vi "One Ring_2016_11_03_AMZ_LoopTPX_Beta.vi"() -> ()   [LabVIEW 2015]
uses:
  <vilib>/Platform/TimedLoop/XDataNode/timing_clust.ctl
  <vilib>/Platform/TimedLoop/XDataNode/nitl_modes.ctl
  <vilib>/Platform/TimedLoop/XDataNode/wakeup.ctl
  <vilib>/Utility/file.llb/Read From Spreadsheet File (DBL).vi
  <vilib>/Utility/file.llb/Write To Spreadsheet File (string).vi
  <vilib>/Platform/TimedLoop/XDataNode/XDataNode.xnode
  <vilib>/Platform/TimedLoop/XDataNode/XDNodeRunTimeDep.lvlib
  OE_Group/OE_Research/Programs/JW-PD/Instrument Libraries/Lake Shore 336/Lake Shore 336.lvlib
panel:
  in  "Stop \nCountdown 2":bool
  in  "Loop Wait 2":dbl format="%<%H:%M:%S>t"
  out "Wait Countdown 2":dbl format="%<%H:%M>t"
  out "all rows":dbl[][](array[numeric]) format="%0.3f"
  out "Repeat Loop":i32
  out "Measurement Repeat":bool
  out "Measurement Error":bool
  out "Stop buffer":dbl
  out "Start buffer":dbl
  out "Status":path
  out "Settle Time (s)":dbl
  out "Current Step":dbl
  out "D":dbl
  out "I":dbl
  out "P":dbl
  out "Out2 Ramp":dbl
  out "Out1 Ramp":dbl
  out "Temp Max Alarm":bool
  out "Temp Min Alarm":bool
  out "Out 2\nActive":bool
  out "Out 2\nRamp On":bool
  out "Out 1\nRamp On":bool
  out "Out 1\nActive":bool
  in  "Time Iteration (s)":dbl=30.0
  out "Electrical Measurements":path
  out "Temperature Measurements":path
  out "output control loop":dbl
  out "AutoTune Stage":dbl
  out "AutoTune Error":bool
  out "AutoTune Active":bool
  out "Array 2":i32[](array[numeric])
  out "Array":i32[](array[numeric])
  out "Start Time Num":dbl
  in  "Temp Sample Time (s)":dbl
  out "Current Rate (K/min)":dbl
  in  "Tab Control":T1(tab)
  in  "Light Bathe Cluster":T2={"TG to BG (TRF):  "=FALSE, "TG to BG Durration"=120.0, "TRF to TSP:   "=FALSE, "TG to BG Durration 2"=120.0, "Post Measure: "=TRUE, "TG to BG (TSP):"=FALSE, "TG to BG Durration 3"=120.0} {"TG to BG Durration 3" format="%<%H:%M:%S>t"; "TG to BG Durration 2" format="%<%H:%M:%S>t"; "TG to BG Durration" format="%<%H:%M:%S>t"}
  in  "Gated SMU4 is...":bool
  in  "Light is...":bool
  in  "SD Transport Tab":enum32{"Transport", "Gate Current"}(tab)
  out "Transport Graph":cluster{dbl[], "trace":dbl[]}[](graph) caption="Transfer"
  out "TSP Gate Current":cluster{"Y":dbl[], "Y":dbl[]}[](graph)
  in  "SD Transfer Tab":T3(tab)=enum."Saturation"
  out "Linear Transfer":cluster{"Y":dbl[], "Y":dbl[]}[](graph)
  out "Saturation Transfer":cluster{"Y":dbl[], "Y":dbl[]}[](graph)
  out "Linear Raw":cluster{"Y":dbl[], "Y":dbl[]}[](graph)
  out "Saturation Raw":cluster{"Y":dbl[], "Y":dbl[]}[](graph)
  out "TSF Gate Current":cluster{"Y":dbl[], "Y":dbl[]}[](graph)
  out "Off Current":dbl format="%#_3g"
  out "Mobility-Lin":dbl format="%#_3g"
  out "Trap Density-VT":dbl format="%#_3g"
  in  "First Step":dbl
  out "Trap Density-STS":dbl format="%#_3g"
  out "STS":dbl format="%#_3g"
  out "Vt":dbl format="%#_3g"
  in  "Transfer 2":bool=TRUE
  in  "Transport":bool=TRUE
  out "Error":errorcluster
  in  "Integration Time 3":u32(slide) scale=0.0..2.0
  in  "Integration Time":u32(slide) scale=0.0..2.0
  in  "Start 2":dbl=40.0 format="%.2f"
  in  "Stop 2":dbl=-40.0 format="%.2f"
  in  "Step 2":dbl=-1.0 format="%.2f"
  in  "Start":dbl=-2.0 format="%.2f"
  in  "Total Points":u16=2
  in  "Step":dbl=-38.0 format="%.2f"
  in  "Sample Properties:":T4={"Date Created"=timestamp(0 s since 1904-01-01), "Material"="", "Solvent"="", "Concentration"="", "Method"="", "Dielectric (d)"="", "Index (#)"="", "Index (ABC)"="", "Length"="", "Width"="", "Surface Treatment"="", "Comments"="", "T (K)"=294.0} {"T (K)" format="%#_4g"; "Date Created" format="%<%Y/%m/%d>T"}
  in  "Start":dbl format="%.2f"
  in  "Stop 3":dbl=-60.0 format="%.2f"
  in  "Step":dbl=-1.0 format="%.2f"
  in  "Start":dbl format="%.2f"
  in  "Total Points":u16=7
  in  "Step":dbl=-10.0 format="%.2f"
  out "TRF Path":path
  out "TSP Path":path
  in  "OK Button":bool
  in  "stop":bool
  out "Status LED":bool
  in  "Wait Time (s)":dbl format="%.1g"
  out "Wait Countdown":dbl format="%<%H:%M>t"
  out "Mobility-Sat":dbl format="%#_3g"
  out "On/Off":dbl format="%#_3g"
  in  "# of Loops":dbl=1.0
  in  "Loop Step":dbl
  in  "Loop Wait":dbl format="%<%H:%M:%S>t"
  in  "Stop \nCountdown":bool
  out "Delay Start":dbl format="%<%H:%M:%S>t"
  out "Light \nCount Down":dbl format="%<%H:%M:%S>t"
  in  "Light On Duration\n (min)":dbl
  in  "PR OVR":bool
  in  "PT OVR":bool
  in  "Reverse Scan (Y/N)":bool
  in  "Post Rate (K/min)":dbl format="%_2g"
  in  "Post Temp (K)":dbl format="%_4g"
  out "Status Table":string[][](table)
  out "Elapsed Time":dbl format="%<%H:%M:%S>t"
  out "Start Time":timestamp format="%<%I:%M:%S %p\n%x>T"
  out "Temp Graph":cluster{"Y":dbl[], "Y":dbl[]}[](graph)
  out "Room Temp (K)":dbl
  in  "Output 1 Range":enum16{"Off", "Low (On)", "Medium", "High"}(ring)=enum."High"
  in  "Output 2 Range":enum16{"Off", "Low (On)", "Medium", "High"}(ring)=enum."High" caption="Range (0:Off)"
  in  "Rate (K/min)":dbl=0.5 format="%.2f"
  out "Heater 3 Output":dbl format="%_3g"
  out "Heater 4 Output":dbl format="%_3g"
  in  "Sample Control":bool=TRUE
  in  "Radiation Sheild":bool=TRUE
  in  "Start (K)":dbl=80.0 format="%.2f"
  in  "# Steps":dbl=22.0
  in  "Stop (K)":dbl=300.0 format="%.2f"
  in  "Abort?":bool
  in  "TPX OK Button":bool
  out "TPX Transport Graph":cluster{"trace":dbl[], "trace":dbl[]}(graph)
  out "TPX Transfer Graph":cluster{"Y":dbl[], "Y":dbl[]}[](graph)
  out "Target":dbl caption="Target (K)"
  out "Setpoint (K)":dbl
  in  "Reset":bool
  out "Alarm":bool
  out "2":bool
  out "1":bool
  out "A:  Sample Stage":dbl format="%_6g"
  out "C:  Probe Arm":dbl format="%_6g"
  out "B:  Rad Shield":dbl format="%_6g"
  out "D:  Not Used":dbl format="%_6g"
  out "Heater 1 Output2":dbl format="%_3g"
  out "Heater 2 Output1":dbl format="%_3g"
  out "Mobility-Sat TPX":dbl caption="Mobility-Sat" format="%#_3g"
  out "On/Off TPX":dbl caption="On/Off" format="%#_3g"
  out "Vt TPX":dbl caption="Vt" format="%#_3g"
  out "STS TPX":dbl caption="STS" format="%#_3g"
  out "Trap Density STS TPX":dbl caption="Trap Density-STS" format="%#_3g"
  out "Trap Density VT TPX":dbl caption="Trap Density-VT" format="%#_3g"
  out "Mobility-Lin TPX":dbl caption="Mobility-Lin" format="%#_3g"
  out "Off Current TPX":dbl caption="Off Current" format="%#_3g"
  in  "User's Name":u16(ring) items=["Abdul", "Derek", "Jeremy", "Joshua", "Katelyn", "Oana", "Pete", "Zach"]
  in  "User's Email":string
  in  "Edit Users":bool
  in  "Top Gate Dielectric Properties":T5 {"Dielectric Constant (TG)" format="%#.2g"}
  in  "Gate Current Cluster":T6={"Gate Current (TSP)"={"Y2 axis on/off"=FALSE, "MINIMUM"=0.0, "MAXIMUM"=1.0, "Variable name"="Ig", "LIN or LOG axis"="LIN"}, "Gate Current (TRF)"={"Y2 axis on/off"=FALSE, "MINIMUM"=0.0, "MAXIMUM"=1.0, "Variable name"="Ig", "LIN or LOG axis"="LIN"}} {"Gate Current (TRF)"."MAXIMUM" format="%.3f"; "Gate Current (TRF)"."MINIMUM" format="%.3f"; "Gate Current (TSP)"."MAXIMUM" format="%.3f"; "Gate Current (TSP)"."MINIMUM" format="%.3f"}
  in  "Continue if error?":bool
  out "Error Loop #":dbl
  in  "Repeat if error?":bool
  in  "Name/Email List Location":path=path "C:/Program Files/One Ring 1.0/User_Directory.txt"
  in  "Text Editor Location":path=path "C:/Program Files/Notepad++/notepad++.exe"
  in  "Stability Time (s)":dbl=15.0
  in  "Setpoint Tolerance (K)":dbl=0.5
  in  "D: Low Alarm":dbl
  in  "D: High Alarm":dbl
  in  "Var1 sweep settings":T7={"sweep spacing (linear: 0)"=0, "sweep mode"=FALSE, "compliance (V)"=100.0, "compliance (A)"=0.001} {"compliance (A)" format="%^.2e"; "compliance (V)" format="%.2f"; "sweep spacing (linear: 0)" items=["linear", "log 10", "log 25", "log 50"]}
  in  "Var2 step settings":T8={"compliance (A)"=0.001, "compliance (V)"=100.0} {"compliance (V)" format="%.2f"; "compliance (A)" format="%^.2e"}
  in  "Var1 sweep settings 2":T7={"sweep spacing (linear: 0)"=0, "sweep mode"=FALSE, "compliance (V)"=100.0, "compliance (A)"=0.001} {"compliance (A)" format="%^.2e"; "compliance (V)" format="%.2f"; "sweep spacing (linear: 0)" items=["linear", "log 10", "log 25", "log 50"]}
  in  "Var2 step settings 2":T8={"compliance (A)"=0.001, "compliance (V)"=100.0} {"compliance (V)" format="%.2f"; "compliance (A)" format="%^.2e"}
  in  "B: Low Alarm":dbl
  in  "A: Low Alarm":dbl
  in  "B: High Alarm":dbl=350.0
  in  "A: High Alarm":dbl=350.0
  in  "C: Low Alarm":dbl
  in  "C: High Alarm":dbl
  in  "Alarm Reset 2":bool
  in  "P 2":dbl=200.0 caption="P"
  in  "I 2":dbl=50.0 caption="I"
  in  "D 2":dbl caption="D"
  in  "VISA Resource (TPX)":refnum<visa-resource-name>="GPIB9::12::INSTR"
  in  "SetPoint2\nOVR":dbl=294.0 caption="Setpoint Overide (K)"
  in  "VISA resource name":refnum<visa-resource-name>="GPIB0::17::INSTR"
  in  "Data Folder":path=path "C:/1DATA"
  in  "Image Folder:":path=path "C:/1Data/2012/zOops"
  out "Image File:":path=path "C:/Users/shuttle/Desktop"
  in  "Dielectric Constant:":dbl=3.9 format="%_2g"
  in  "Saved Folder:":path=path "C:/Users/shuttle/Desktop"
  # "Device Characteristics"
  # "Vg Sweep"
  # "Vd Step"
  # "Loops and Integration Time"
  # "Integration Time"
  # "Vd Step"
  # "Vg Step"
  # "Light Bath is..."
  # "Duration (hh:mm:ss)"
  # "Sample Properties:"
  # "%"
  # "nm"
  # "Device Properties:"
  # "um"
  # "um"
  # "Step 1:  Temperature Settings"
  # "Sample Stage"
  # "Radiation Shield"
  # "Instrument Status"
  # "Step 2:  Set the following in \"Super Duper\""
  # "%"
  # "%"
  # "K"
  # "K"
  # "1)   Sample Properties\n\n2)   Device Properties\n\n3)   Transfer and Transport Parameters"
  # "K"
  # "K"
  # "Step 3: End of Measurement Options"
  # "Device Characteristics"
  # "Lake Shore 336 Temperature Controller"
  # "Agilent 4155C Semiconductor Parameter Analyzer"
  # "One Ring Preferences"
  # "K"
  # "K"
  # "K"
  # "K"
  # "K"
  # "K"
  # "K"
  # "K"
  # "Notification Preferences"
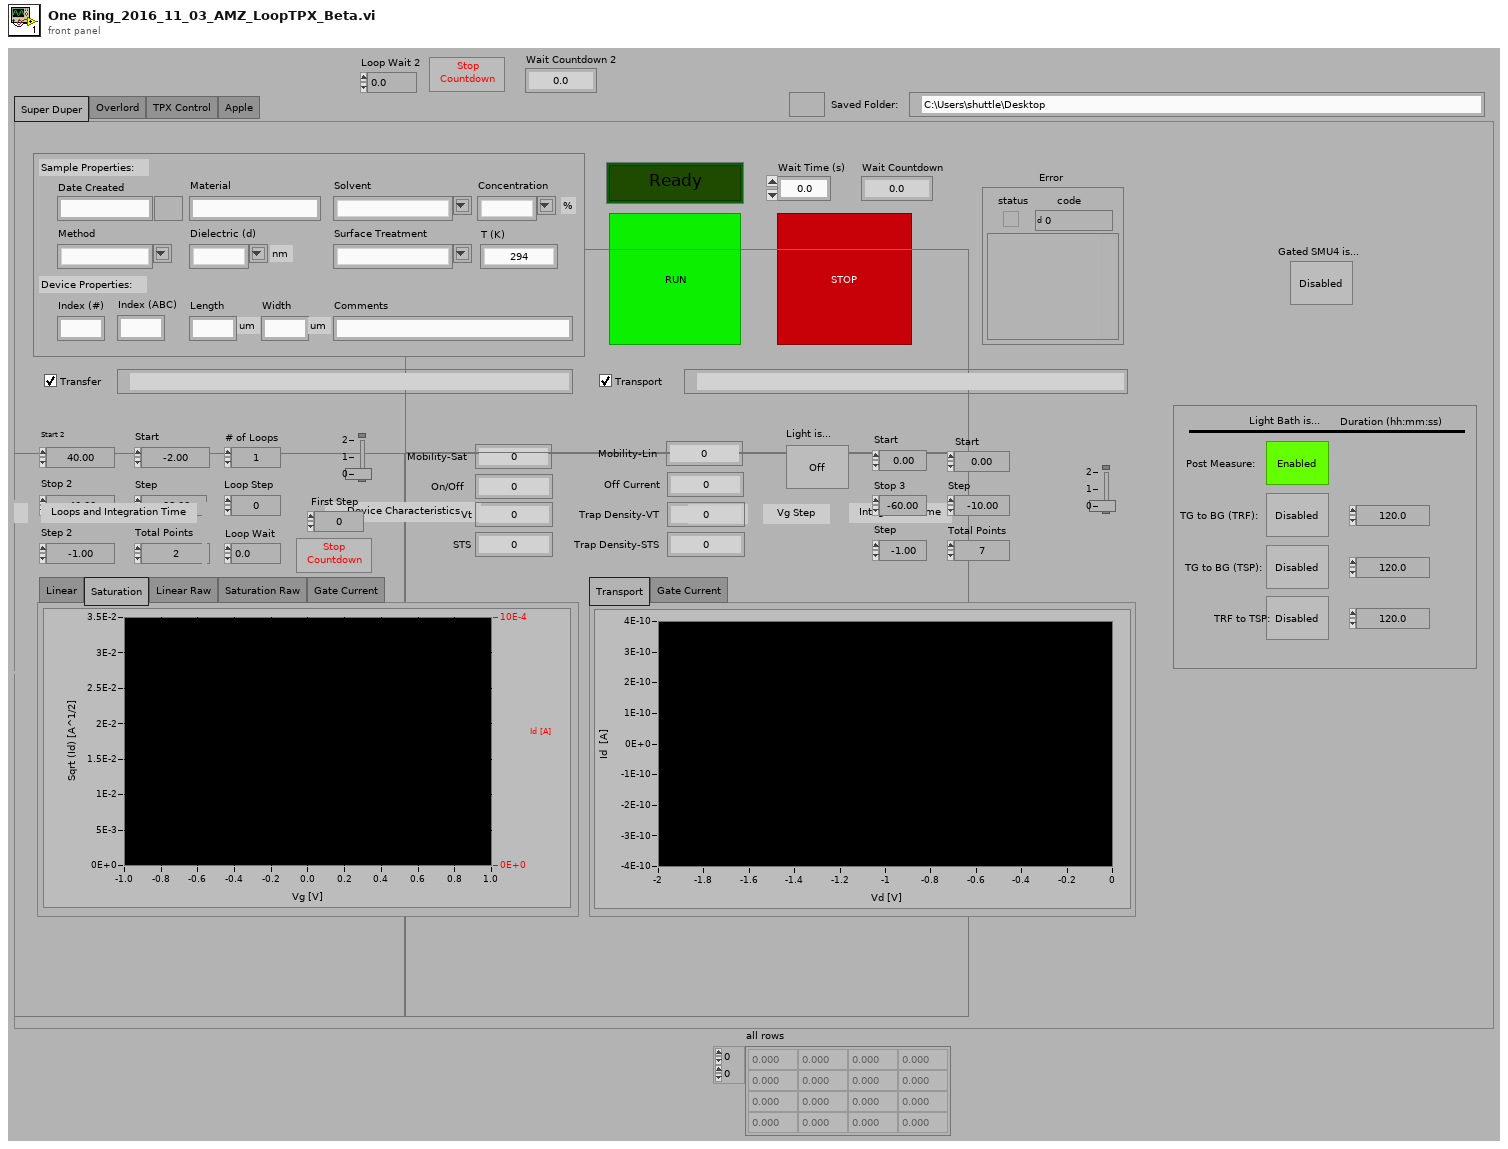
[diagram p1: front panel]
types:
  T1 = enum32{"Super Duper", "Overlord", "TPX Control", "Apple"}
  T2 = cluster{"TG to BG (TRF):  ":bool, "TG to BG Durration":dbl, "TRF to TSP:   ":bool, "TG to BG Durration 2":dbl, "Post Measure: ":bool, "TG to BG (TSP):":bool, "TG to BG Durration 3":dbl}
  T3 = enum32{"Linear", "Saturation", "Linear Raw", "Saturation Raw", "Gate Current"}
  T4 = cluster{"Date Created":timestamp, "Material":string, "Solvent":string, "Concentration":string, "Method":string, "Dielectric (d)":string, "Index (#)":string, "Index (ABC)":string, "Length":string, "Width":string, "Surface Treatment":string, "Comments":string, "T (K)":dbl}
  T5 = cluster{"Dielectric Constant (TG)":dbl, "Dielectric (d) (TG)":string}
  T6 = cluster{"Gate Current (TSP)":cluster{"Y2 axis on/off":bool, "MINIMUM":ext, "MAXIMUM":ext, "Variable name":string, "LIN or LOG axis":string}, "Gate Current (TRF)":cluster{"Y2 axis on/off":bool, "MINIMUM":ext, "MAXIMUM":ext, "Variable name":string, "LIN or LOG axis":string}}
  T7 = cluster{"sweep spacing (linear: 0)":u16, "sweep mode":bool, "compliance (V)":dbl, "compliance (A)":dbl}
  T8 = cluster{"compliance (A)":dbl, "compliance (V)":dbl}
  T9 = typedef "XDNodeRunTimeDep.lvlib/timing_clust.ctl" = cluster{"Expected End [f-1]":u64, "Actual End [f-1]":u64, "Finished Late? [f-1]":bool, "Expected End [i-1]":u64, "Actual End [i-1]":u64, "Finished Late? [i-1]":bool, "Expected Start [i]":u64, "Actual Start [i]":u64, "Expected Start [f]":u64, "Actual Start [f]":u64, "Source Name":string, "Structure Name":string, "Period":i64, "Deadline":i64, "Offset":i64, "Start":i64, "Priority":i32, "Timeout":i32, "Mode":T10, "Wakeup Reason":T11, "Error":errorcluster, "Source Type":string, "Secondary Source Type":string, "Global End Time":u64, "Global Start Time":u64, "Frame Duration":u64, "Iteration Duration":u64, "Assigned CPU":i32, "I/O Scan Engine Mode":u32}
  T10 = typedef "XDNodeRunTimeDep.lvlib/nitl_modes.ctl" = enum32{"No Change", "Process missed periods, maintain original phase", "Discard missed periods, maintain original phase", "Process missed periods, ignore original phase", "Discard missed periods, ignore original phase"}
  T11 = typedef "XDNodeRunTimeDep.lvlib/wakeup.ctl" = enum32{"Normal", "Aborted", "Asynchronous wakeup", "Timing source error", "Timed loop error", "Timeout"}
  T12 = cluster{"P":dbl, "I":dbl, "D":dbl, "SetPoint Out1":dbl, "SetPoint Out2":dbl, "1":bool, "2":bool, "output control loop":dbl, "AutoTune Error":bool, "AutoTune Active":bool, "AutoTune Stage":dbl, "Out1 Active":bool, "Out1 Ramp On":bool, "Out2 Active":bool, "Out2 Ramp On":bool, "Heater 2 Output 1":dbl, "Heater 1 Output 2":dbl, "Out1 Ramp":dbl, "Out2 Ramp":dbl}
  T13 = cluster{"A:  Sample Stage":dbl, "B:  Rad Shield":dbl, "B: Probe Arm":dbl, "Temp Max Alarm":bool, "Temp Min Alarm":bool}
  T14 = cluster{"Wait Countdown":dbl, "Wait Time (s)":dbl}
  T15 = cluster{"Step":dbl, "# of Loops":dbl, "Transfer 2":bool, "Start":dbl, "Total Points":u16, "Start 2":dbl, "Stop 2":dbl, "Step 2":dbl, "Loop Step":dbl, "Integration Time 3":u32, "Loop Wait":dbl, "First Step":dbl}
  T16 = cluster{bool, "Start":dbl, "Stop 3":dbl, "Step":dbl, "Start":dbl, "Step":dbl, "Total Points":u16, "Integration Time":u32}
  T17 = cluster{"Var1 sweep settings":cluster{"sweep spacing (linear: 0)":u16, "sweep mode":bool, "compliance (V)":dbl, "compliance (A)":dbl}, "Var1 sweep settings 2":cluster{"sweep spacing (linear: 0)":u16, "sweep mode":bool, "compliance (V)":dbl, "compliance (A)":dbl}, "Var2 step settings":cluster{"compliance (A)":dbl, "compliance (V)":dbl}, "Var2 step settings 2":cluster{"compliance (A)":dbl, "compliance (V)":dbl}}
  T18 = cluster{"Linear Transfer":cluster{dbl[], "trace":dbl[]}[], "Linear Raw":cluster{dbl[], dbl[]}[], "Saturation Transfer":cluster{dbl[], "trace":dbl[]}[], "Saturation Raw":cluster{dbl[], dbl[]}[], "Transport":cluster{dbl[], dbl[]}[], "TRF Gate Current":cluster{dbl[], dbl[]}[], "TSP Gate Current":cluster{dbl[], dbl[]}[]}
  T19 = cluster{"Mobility-Sat":dbl, "Mobility-Lin":dbl, "On/Off ":dbl, "Off I":dbl, "Vt":dbl, "STS":dbl, "Trap Density-VT":dbl, "Trap Density-STS":dbl}
  T20 = cluster{"Step":dbl, "# of Loops":dbl, bool, "Start":dbl, "Total Points":u16, "Start 2":dbl, "Stop 2":dbl, "Step 2":dbl, "Loop Step":dbl, "Integration Time 3":u32, "Loop Wait":dbl, "First Step":dbl}
  T21 = cluster{"Transport":bool, "Start":dbl, "Stop 3":dbl, "Step":dbl, "Start":dbl, "Step":dbl, "Total Points":u16, "Integration Time":u32}
  T22 = cluster{"Date Created":timestamp, "Material":string, "Solvent":string, "Concentration":string, "Method":string, "Dielectric (d)":string, "Index (#)":string, "Index (ABC)":string, "Length":string, "Width":string, "Surface Treatment":string, "Comments":string, "A:  Sample Stage":dbl}
  T23 = cluster{"Vt Max":i32, "Vt Min":i32, "Vt Ratio":i32, "Id Max":i32}
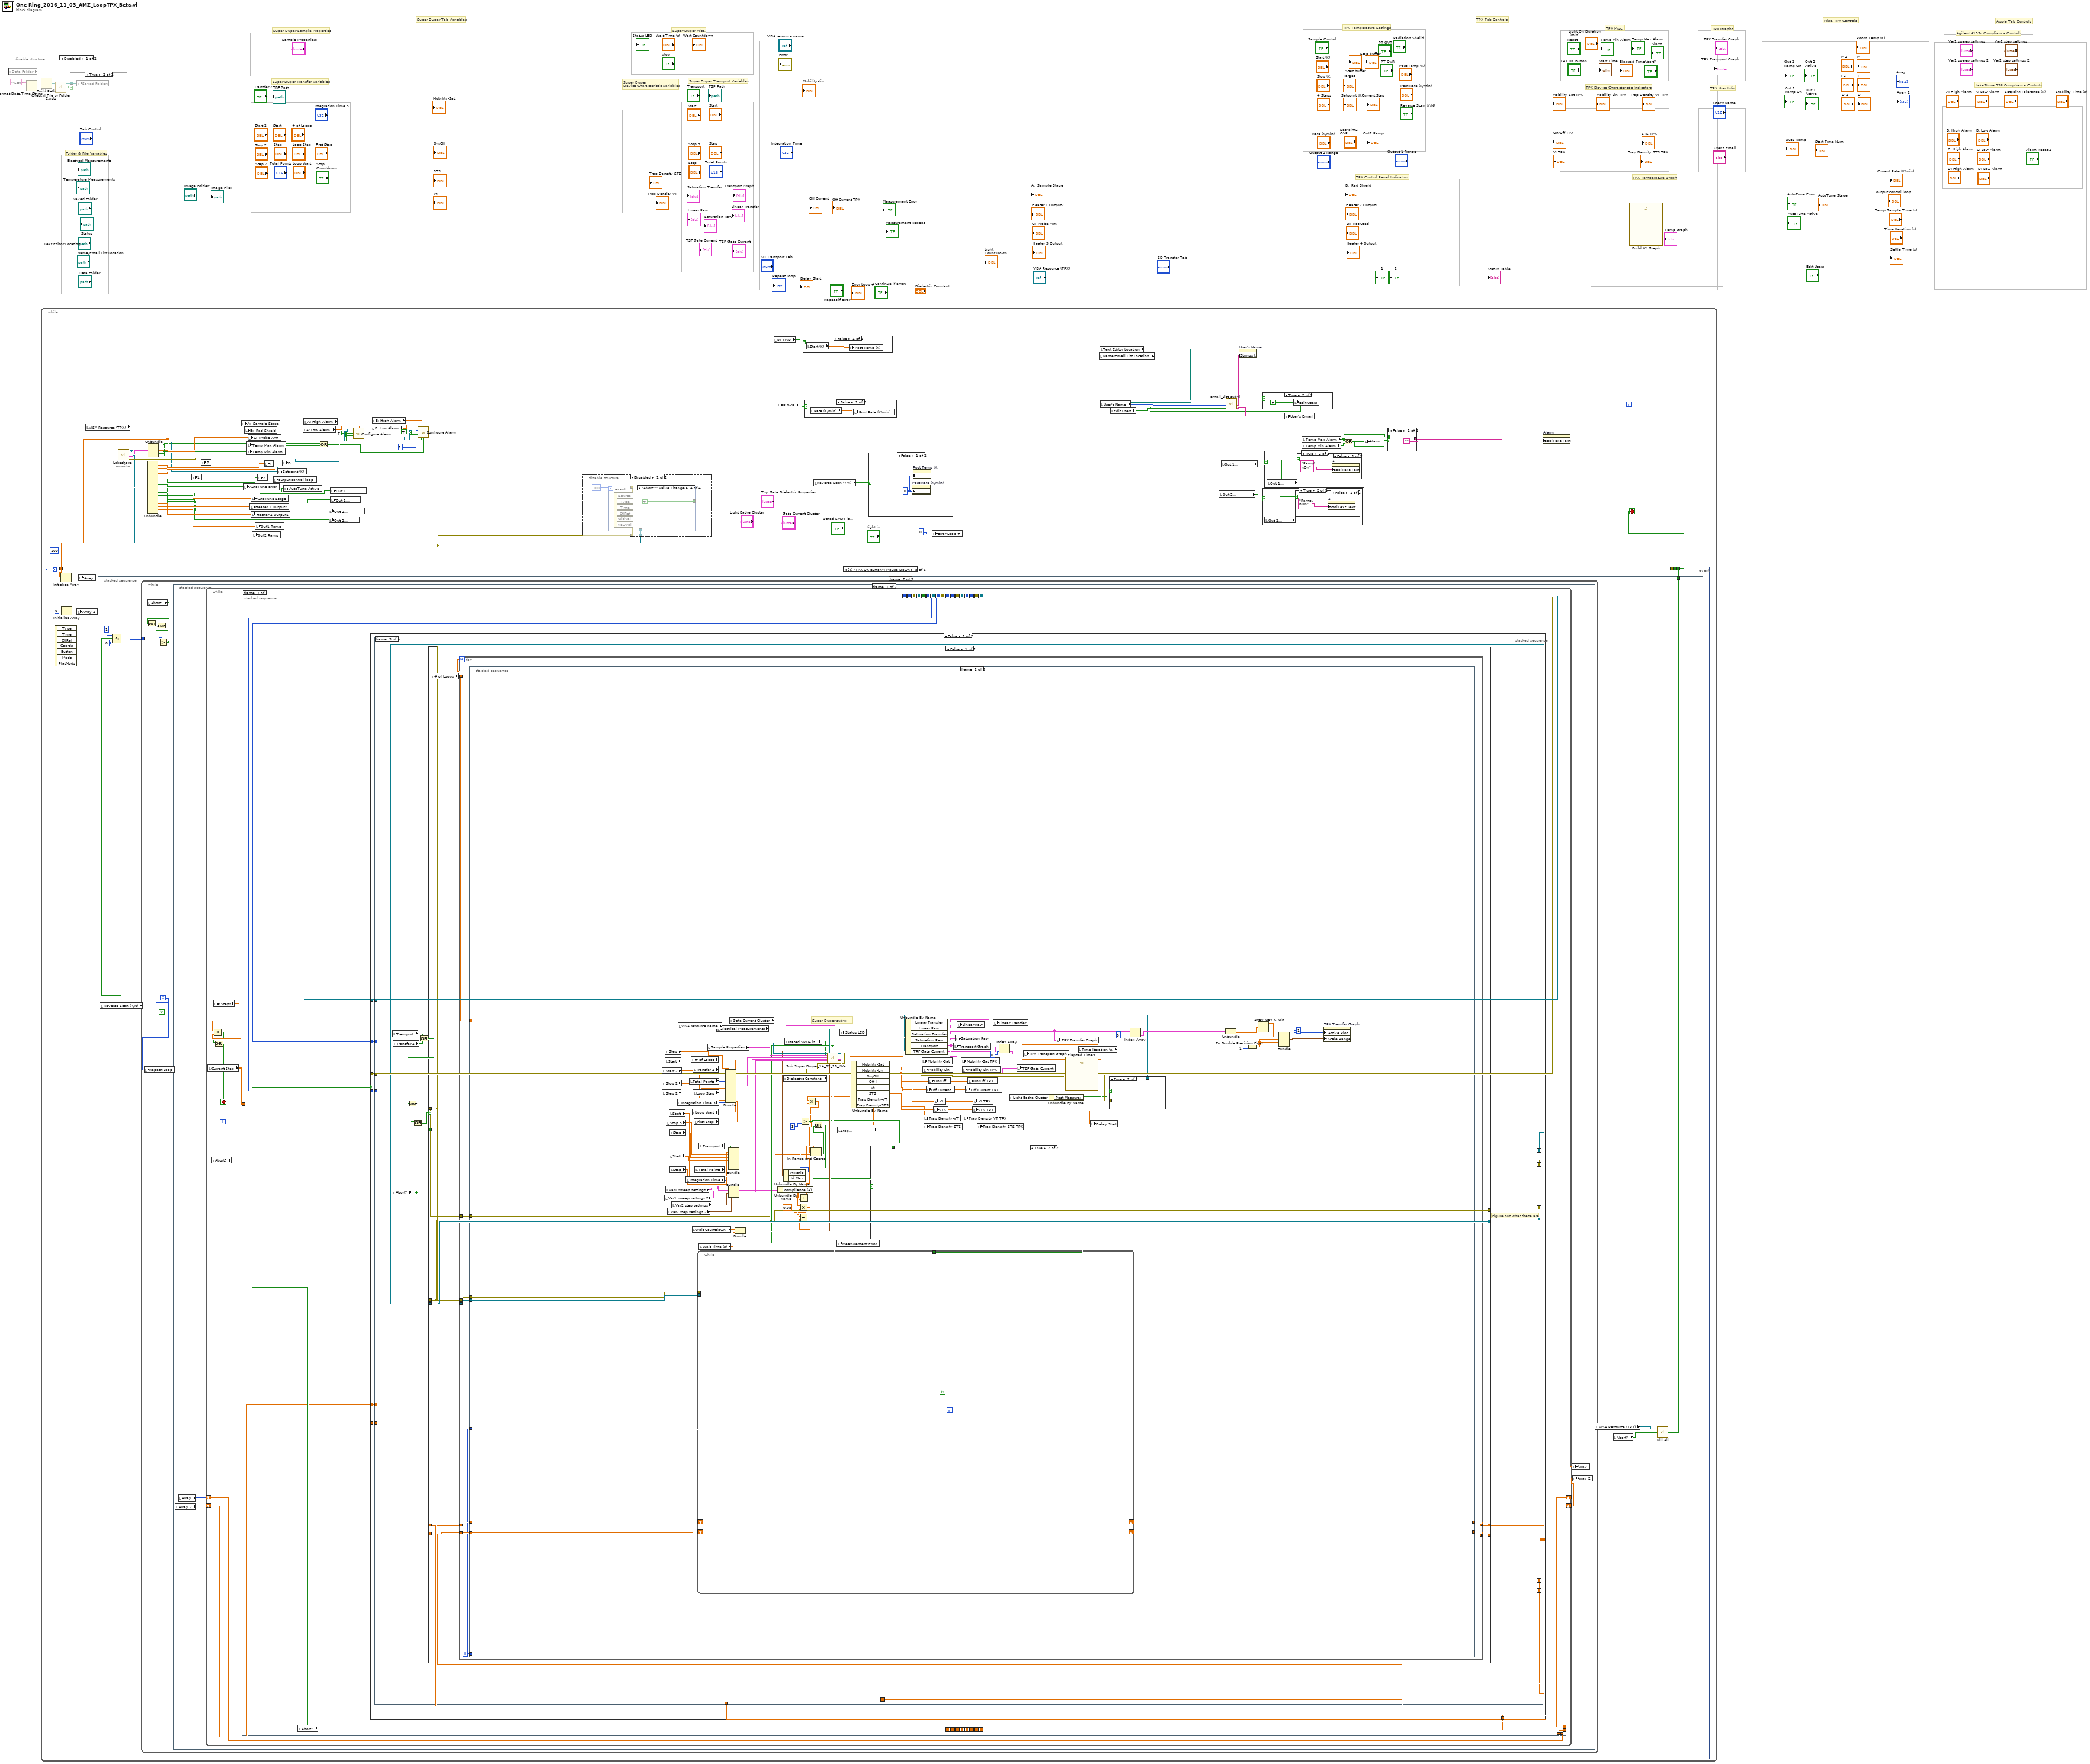
[diagram p0: block diagram]
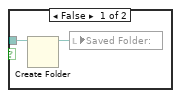
[diagram p2: hidden frame]
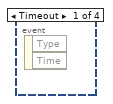
[diagram p4: hidden frame]
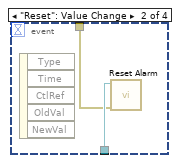
[diagram p5: hidden frame]
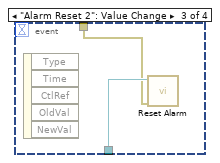
[diagram p6: hidden frame]
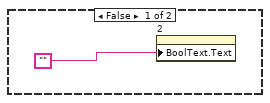
[diagram p8: hidden frame]
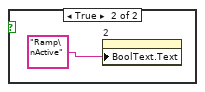
[diagram p9: hidden frame]
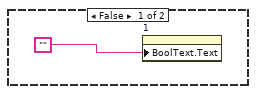
[diagram p10: hidden frame]
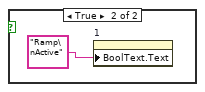
[diagram p11: hidden frame]
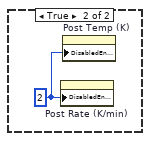
[diagram p14: hidden frame]
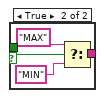
[diagram p16: hidden frame]
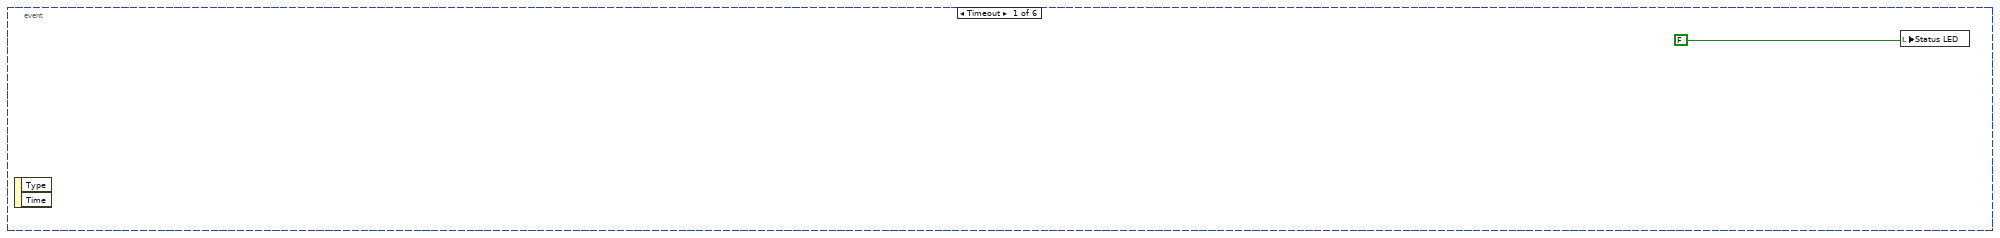
[diagram p17: hidden frame]
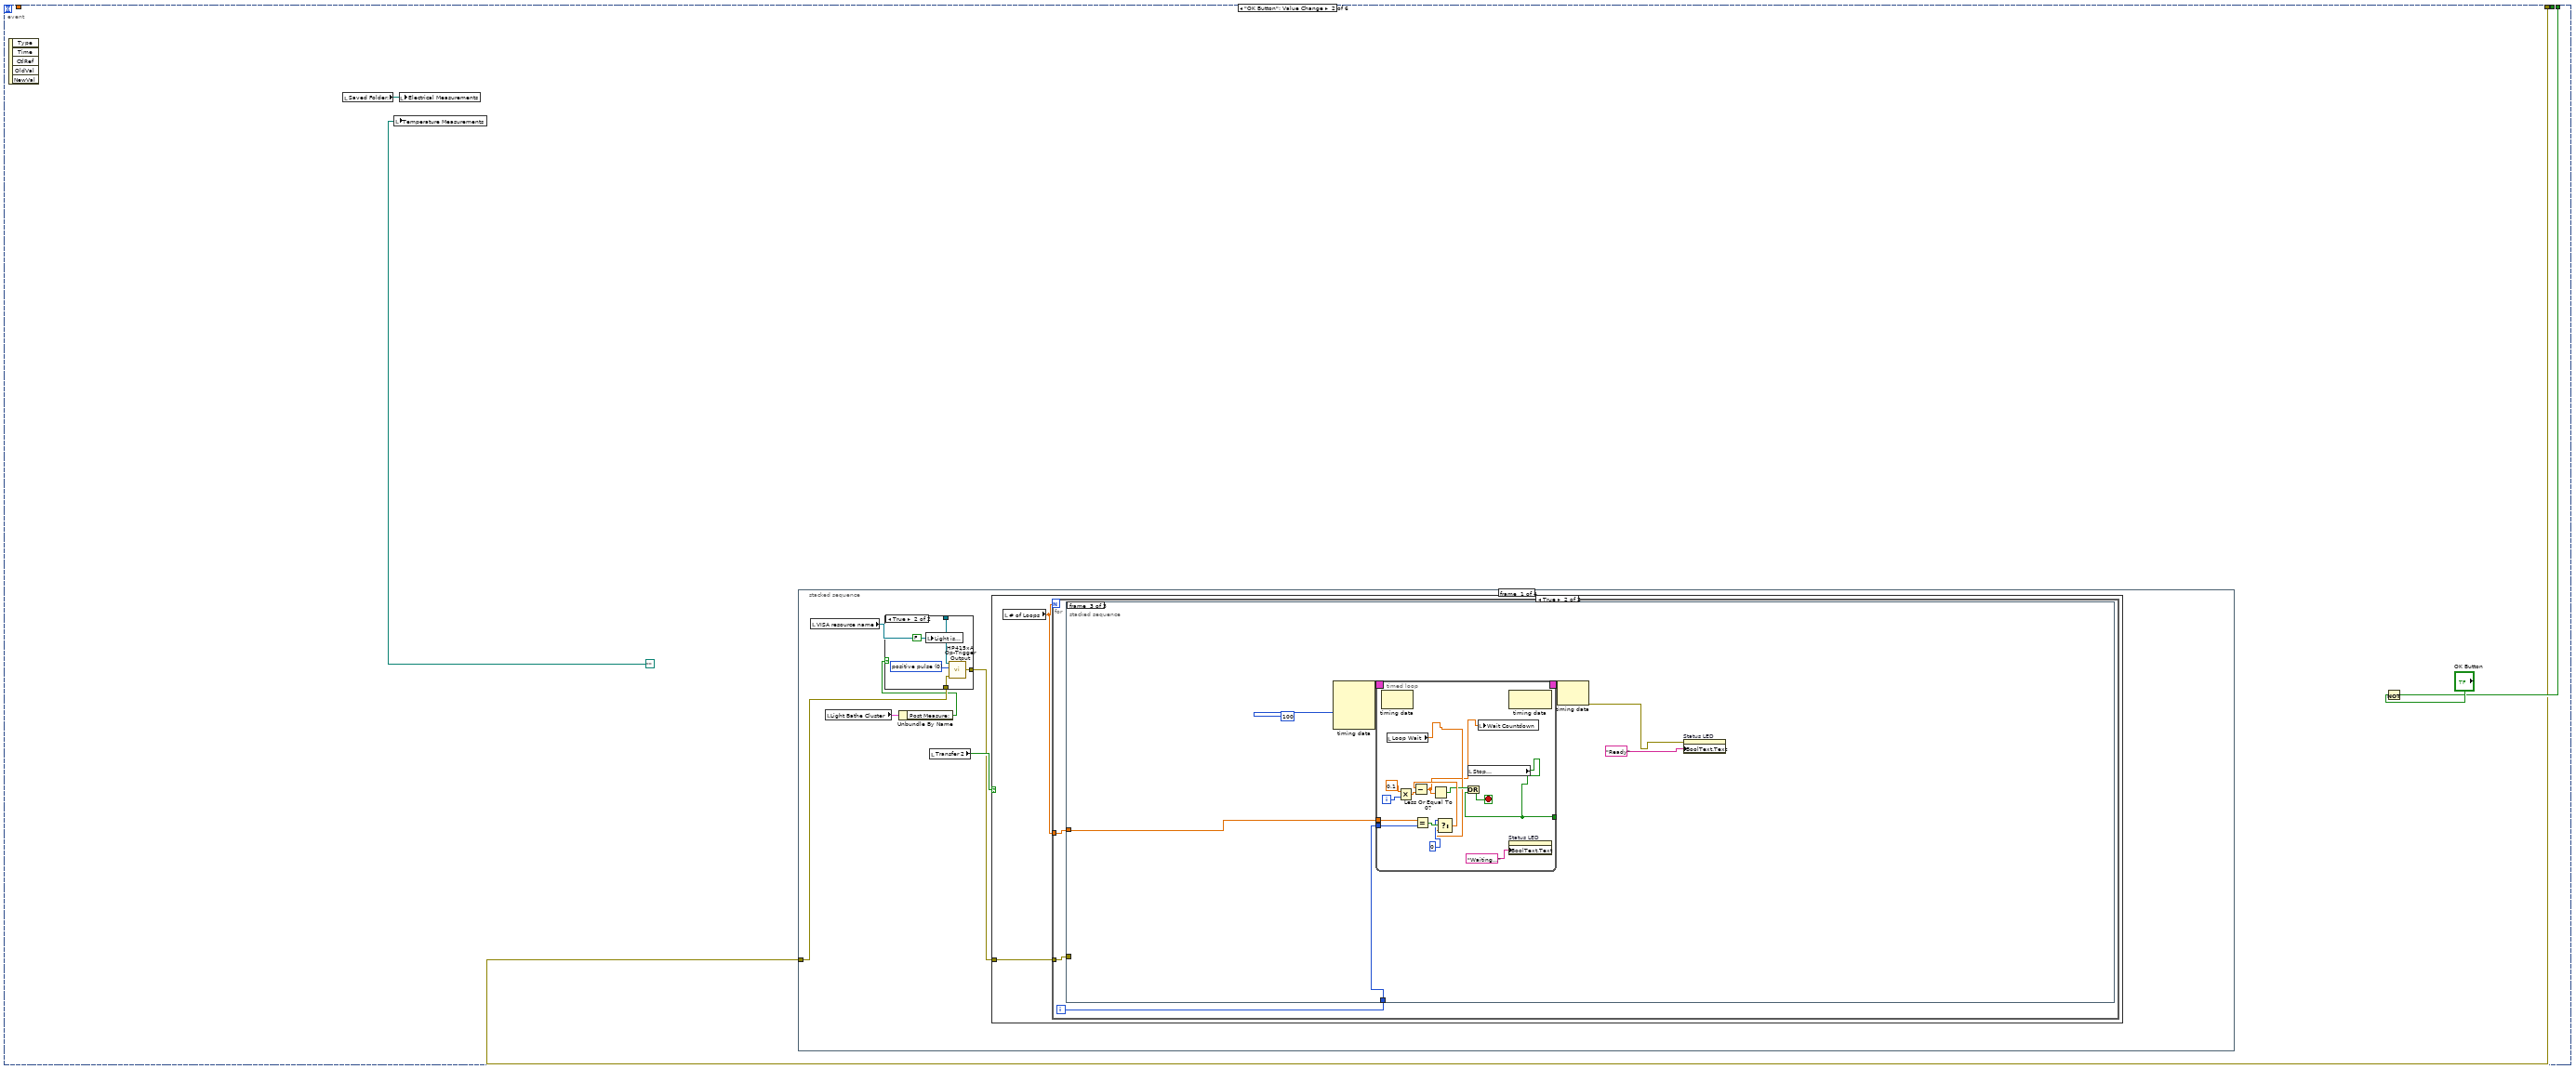
[diagram p18: hidden frame]
diagram:
  # "TPX User Info"
  # "TPX Temperature Graph"
  # "Misc. TPX Controls"
  # "Apple Tab Controls"
  # "LakeShore 336 Compliance Controls"
  # "Agilent 4155c Compliance Controls"
  # "TPX Graphs"
  # "TPX Tab Controls"
  # "TPX Misc."
  # "TPX Device Characteristic Indicators"
  # "TPX Control Panel Indicators"
  # "Folder & File Variables"
  # "TPX Temperature Settings"
  # "Super Duper Tab Variables"
  # "Super Duper Misc."
  # "Super Duper Sample Properties"
  # "Super Duper Transport Variables"
  # "Super Duper Transfer Variables"
  # "Super Duper\nDevice Characteristic Variables"
  n1 = disable-structure shown="Disabled" {
    frame Disabled {
      n2 = local read "Data Folder"() -> (w2:path)
      n3 = Format Date/Time String(time format string (%c)="%#Y") -> (date/time string=w6:string)  [unwired: 2 in]
      n4 = Build Path(base path=w2, name or relative path=w6) -> (appended path=w5:path)
      n5 = call <vilib>:"Check if File or Folder Exists.vi"("path"=w5) -> ("file or folder exists?"=w4:bool, "dup path"=w3:path)  [unwired: 8 in, 1 out]
      n6 = case shown="True" w4 {
        tunnel: w3 -> [w9 w10]
        frame False {
          n7 = Create Folder(path (use dialog)=w9) -> (created path=w8:path)  [unwired: 2 in, 2 out]
          n8 = local write "Saved Folder:"(w8) -> ()
        }
        frame True {
          n9 = local write "Saved Folder:"(w10) -> ()
        }
      }
    }
    frame Enabled {
    }
  }
  n10 = while {
    stop <- w58 stop-if-true
    w14 = TRUE
    w23 = TRUE
    n11 = local read "VISA Resource (TPX)"() -> (w29:refnum<visa-resource-name>)
    n12 = call "Lakeshore_monitor.vi"("VISA Resource (TPX)"=w29) -> ("error?"=w63:errorcluster, "Outputs"=w27:T12, "Inputs"=w28:T13, "VISA resource name"=w26:refnum<visa-resource-name>)  [unwired: 6 in]
    n13 = Unbundle(w27) -> ("P"=w43:dbl, "I"=w42:dbl, "D"=w41:dbl, "SetPoint Out2"=w40:dbl, "1"=w39:bool, "2"=w38:bool, "output control loop"=w37:dbl, "AutoTune Error"=w36:bool, "AutoTune Active"=w35:bool, "AutoTune Stage"=w34:dbl, "Out1 Active"=w20:bool, "Out1 Ramp On"=w19:bool, "Out2 Active"=w18:bool, "Out2 Ramp On"=w17:bool, "Heater 2 Output 1"=w33:dbl, "Heater 1 Output 2"=w30:dbl, "Out1 Ramp"=w32:dbl, "Out2 Ramp"=w31:dbl)  [unwired: 1 out]
    n14 = Unbundle(w28) -> ("A:  Sample Stage"=w64:dbl, "B:  Rad Shield"=w45:dbl, "B: Probe Arm"=w44:dbl, "Temp Max Alarm"=w25:bool, "Temp Min Alarm"=w24:bool)
    n15 = event shown="[4] \"TPX OK Button\": Mouse Down" {
      selector: _ -> [_ _ _ _ _ _]
      dyn-events: _ -> [_ _ _ _ _ _]
      timeout: 100 -> [_ _ _ _ _ _]
      tunnel: [_ w96 _ _ w324 w1775] -> w58
      tunnel: [_ _ _ _ _ w1776] -> _
      tunnel: w64 -> [_ _ _ _ w327 _]
      tunnel: w63 -> [_ w95 _ _ _ _]
      event Timeout {
        n16 = event-data() -> ()  [unwired: 1 in, 2 out]
        n17 = local write "Status LED"(FALSE) -> ()
      }
      event "OK Button": Value Change {
        n18 = event-data() -> ()  [unwired: 1 in, 5 out]
        n19 = local read "Saved Folder:"() -> (w94:path)
        n20 = local write "Temperature Measurements"(path "") -> ()
        n21 = local write "Electrical Measurements"(w94) -> ()
        n22 = stacked-sequence {
          tunnel: w95 -> [w101 _ w248 _]
          frame #0 {
            n23 = local read "VISA resource name"() -> (w102:refnum<visa-resource-name>)
            n24 = local read "Light Bathe Cluster"() -> (w99:T2)
            n25 = Unbundle By Name(w99) -> ("Post Measure:"=w98:bool)
            n26 = case shown="True" w98 {
              tunnel: w102 -> [_ w108]
              tunnel: w101 -> [w104 w107]
              tunnel: [w104 w106] -> w100
              frame False {
              }
              frame True {
                w109 = u32 0 items=["positive pulse  ", "negative pulse  ", "level high  ", "level low  "] ("trigger signal")
                n27 = local write "Light is..."(FALSE ("Light is...")) -> ()
                n28 = call "HP415xA Op-Trigger Output.vi"("error in (no error)"=w107, "trigger signal"=w109, "VISA session"=w108) -> ("error out"=w106:errorcluster)  [unwired: 1 in]
              }
            }
            n29 = local read "Transfer 2"() -> (w103:bool)
            n30 = case shown="True" w103 {
              tunnel: w100 -> [_ w111]
              frame False {
              }
              frame True {
                n31 = local read "# of Loops"() -> (w110:dbl)
                n32 = for {
                  N: w110 -> [_]
                  tunnel: w111 -> [w114]
                  tunnel: w110 -> [w112]
                  i -> [w113]
                  n33 = stacked-sequence {
                    tunnel: w114 -> [w117 _ _]
                    tunnel: w113 -> [w116 _ w198]
                    tunnel: w112 -> [_ _ w197]
                    frame #0 {
                      n34 = flat-sequence {
                        tunnel: w117 -> [w180]
                        tunnel: w116 -> [w179]
                        tunnel: [w119] -> w115
                        tunnel: w115 -> [w181]
                        frame #0 {
                          # "SuperDuper w/o TPX"
                          n35 = local read "Light Bathe Cluster"() -> (w121:T2)
                          n36 = local read "Top Gate Dielectric Properties"() -> (w118:T5)
                          n37 = local read "Start 2"() -> (w171:dbl)
                          n38 = local read "Stop 2"() -> (w170:dbl)
                          n39 = local read "Step 2"() -> (w169:dbl)
                          n40 = local read "Start"() -> (w173:dbl)
                          n41 = local read "Step"() -> (w176:dbl)
                          n42 = local read "Var1 sweep settings 2"() -> (w154:T7)
                          n43 = local read "Stop 3"() -> (w161:dbl)
                          n44 = local read "Var1 sweep settings"() -> (w155:T7)
                          n45 = local read "Gate Current Cluster"() -> (w123:T6)
                          n46 = local read "Wait Countdown"() -> (w146:dbl)
                          n47 = local read "Var2 step settings 2"() -> (w152:T8)
                          n48 = local read "Start"() -> (w162:dbl)
                          n49 = local read "Start"() -> (w159:dbl)
                          n50 = local read "Step"() -> (w160:dbl)
                          n51 = local read "Step"() -> (w158:dbl)
                          n52 = local read "Var2 step settings"() -> (w153:T8)
                          n53 = local read "Wait Time (s)"() -> (w145:dbl)
                          n54 = local read "Integration Time 3"() -> (w167:u32)
                          n55 = local read "VISA resource name"() -> (w148:refnum<visa-resource-name>)
                          n56 = local read "Integration Time"() -> (w156:u32)
                          n57 = local read "Total Points"() -> (w172:u16)
                          n58 = local read "# of Loops"() -> (w175:dbl)
                          n59 = local read "Loop Wait"() -> (w166:dbl)
                          n60 = local read "Transfer 2"() -> (w174:bool)
                          n61 = local read "Loop Step"() -> (w168:dbl)
                          n62 = local read "First Step"() -> (w165:dbl)
                          n63 = local read "Total Points"() -> (w157:u16)
                          n64 = local read "Sample Properties:"() -> (w177:T4)
                          n65 = Bundle("Wait Countdown"=w146, "Wait Time (s)"=w145) -> (w144:T14)  [unwired: 1 in]
                          n66 = local read "Saved Folder:"() -> (w178:path)
                          n67 = Bundle("Step"=w176, "# of Loops"=w175, "Transfer 2"=w174, "Start"=w173, "Total Points"=w172, "Start 2"=w171, "Stop 2"=w170, "Step 2"=w169, "Loop Step"=w168, "Integration Time 3"=w167, "Loop Wait"=w166, "First Step"=w165) -> (w164:T15)  [unwired: 1 in]
                          n68 = Bundle(FALSE, "Start"=w162, "Stop 3"=w161, "Step"=w160, "Start"=w159, "Step"=w158, "Total Points"=w157, "Integration Time"=w156) -> (w163:T16)  [unwired: 1 in]
                          n69 = Bundle("Var1 sweep settings"=w155, "Var1 sweep settings 2"=w154, "Var2 step settings"=w153, "Var2 step settings 2"=w152) -> (w151:T17)  [unwired: 1 in]
                          n70 = local read "Dielectric Constant:"() -> (w125:dbl)
                          n71 = local read "Gated SMU4 is..."() -> (w122:bool)
                          n72 = local read "Stop \nCountdown"() -> (w149:bool)
                          n73 = call "Sub Super Duper_14_02_18_JWa.vi"("VISA resource name"=w148, "Sample Properties:"=w177, "Gated SMU4 is..."=w122, "TRF Cluster"=w164, "TSP Cluster"=w163, "Compliance Cluster"=w151, "Light Bathe Cluster"=w121, "error in"=w180, "Saved Folder:"=w178, "Wait Cluster"=w144, "TG Dielectric Prop"=w118, "Stop \nCountdown"=w149, "Loop Count"=w179, "Gate Current Cluster"=w123, "Dielectric Constant (BG)"=w125) -> ("Status Indicator"=w147:bool, "TRF Path"=w119:path, "TSP Path"=w143:path, "Graph Cluster"=w126:T18, "Char Cluster"=w150:T19)  [unwired: 5 in, 3 out]
                          n74 = local write "Status LED"(w147) -> ()
                          n75 = Unbundle By Name(w150) -> ("Mobility-Sat"=w139:dbl, "Mobility-Lin"=w138:dbl, "On/Off"=w137:dbl, "Off I"=w136:dbl, "Vt"=w135:dbl, "STS"=w134:dbl, "Trap Density-VT"=w133:dbl, "Trap Density-STS"=w132:dbl)
                          n76 = local write "TRF Path"(w119) -> ()
                          n77 = local write "TSP Path"(w143) -> ()
                          n78 = local write "Status LED"(TRUE) -> ()
                          n79 = local write "Light is..."(FALSE) -> ()
                          n80 = local write "Mobility-Lin"(w138) -> ()
                          n81 = local write "Mobility-Sat"(w139) -> ()
                          n82 = local write "Off Current"(w136) -> ()
                          n83 = local write "On/Off"(w137) -> ()
                          n84 = local write "Vt"(w135) -> ()
                          n85 = Unbundle By Name(w126) -> ("Linear Transfer"=w131:cluster{dbl[], "trace":dbl[]}[], "Linear Raw"=w130:cluster{dbl[], dbl[]}[], "Saturation Transfer"=w129:cluster{dbl[], "trace":dbl[]}[], "Saturation Raw"=w128:cluster{dbl[], dbl[]}[], "Transport"=w127:cluster{dbl[], dbl[]}[], "TRF Gate Current"=w124:cluster{dbl[], dbl[]}[])
                          n86 = local write "Trap Density-STS"(w132) -> ()
                          n87 = local write "Trap Density-VT"(w133) -> ()
                          n88 = local write "STS"(w134) -> ()
                          n89 = property on="Status LED" class="Bool (strict)"("BoolText.Text"="Measuring\nTransfer") -> ()  [unwired: 2 in, 2 out]
                          n90 = local write "TSF Gate Current"(w124) -> ()
                          n91 = local write "Transport Graph"(w127) -> ()
                          n92 = local write "Saturation Raw"(w128) -> ()
                          n93 = local write "Linear Transfer"(w131) -> ()
                          n94 = local write "Saturation Transfer"(w129) -> ()
                          n95 = local write "Linear Raw"(w130) -> ()
                        }
                        frame #1 {
                          n96 = local read "Gated SMU4 is..."() -> (w182:bool)
                          n97 = case shown="True" w182 {
                            tunnel: w181 -> [_ w193]
                            frame False {
                            }
                            frame True {
                              n98 = Strip Path(path=w193) -> (stripped path=w191:path, name=w189:string)
                              n99 = Strip Path(path=w191) -> (stripped path=w190:path)  [unwired: 1 out]
                              n100 = Build Path(base path=w190, name or relative path="TRF_SMU4") -> (appended path=w185:path)
                              n101 = List Folder(path=w185) -> (filenames=w188:string[])  [unwired: 3 in, 3 out]
                              n102 = Search 1D Array(1D array=w188, element=w189) -> (index of element=w187:i32)  [unwired: 1 in]
                              n103 = Index Array(array=w188, index=w187) -> (element=w184:string)
                              n104 = Build Path(base path=w185, name or relative path=w184) -> (appended path=w186:path)
                              n105 = call-poly <vilib>:"Read From Spreadsheet File.vi"("file path (dialog if empty)"=w186) -> ("all rows"=→"all rows":dbl[][])  [unwired: 6 in, 4 out]
                            }
                          }
                        }
                      }
                    }
                    frame #1 {
                      n106 = local write "Status LED"(FALSE) -> ()
                    }
                    frame #2 {
                      n107 = node-c288(100) -> (w201:T9)  [unwired: 3 in]
                      n108 = timed-loop {
                        timing: w201 -> [_]
                        timing-out: [_] -> w200
                        tunnel: w198 -> [w211]
                        tunnel: w197 -> [w210]
                        tunnel: [w203] -> _
                        i -> [w215]
                        stop <- w206 stop-if-true
                        n109 = node-c288() -> ()  [unwired: 1 in, 1 out]
                        n110 = local read "Loop Wait"() -> (w205:dbl)
                        n111 = Multiply(x=0.1, y=w215) -> (x*y=w213:dbl)
                        n112 = Equal?(x=w210, y=w211) -> (x = y?=w212:bool)
                        n113 = Select(t=0, s=w212, f=w205) -> (s? t:f=w208:dbl)
                        n114 = Subtract(x=w208, y=w213) -> (x-y=w204:dbl)
                        n115 = Less Or Equal To 0?(x=w204) -> (x <= 0?=w207:bool)
                        n116 = local read "Stop \nCountdown"() -> (w203:bool)
                        n117 = Or(x=w207, y=w203) -> (x .or. y?=w206:bool)
                        n118 = local write "Wait Countdown"(w204) -> ()
                        n119 = node-c288() -> ()  [unwired: 1 in, 1 out]
                        n120 = property on="Status LED" class="Bool (strict)"("BoolText.Text"="Waiting...") -> ()  [unwired: 2 in, 2 out]
                      }
                      n121 = node-c288(w200) -> (w195:errorcluster)
                      n122 = property on="Status LED" class="Bool (strict)"(error in=w195, "BoolText.Text"="Ready") -> ()  [unwired: 1 in, 2 out]
                    }
                  }
                }
              }
            }
          }
          frame #1 {
            n123 = node-c288(1) -> (w225:T9)  [unwired: 1 in]
            n124 = timed-loop {
              timing: w225 -> [_]
              timing-out: [_] -> w224
              i -> [w233]
              stop <- w234 stop-if-true
              n125 = node-c288() -> ()  [unwired: 1 in, 1 out]
              n126 = local read "Wait Time (s)"() -> (w230:dbl)
              n127 = local read "Transport"() -> (w228:bool)
              n128 = Multiply(x=w233, y=0.001) -> (x*y=w231:dbl)
              n129 = local read "Transfer 2"() -> (w229:bool)
              n130 = And(x=w229, y=w228) -> (x .and. y?=w238:bool)
              n131 = Select(t="Waiting...", s=w238, f="Ready") -> (s? t:f=w227:string)
              n132 = Select(t=w230, s=w238, f=0) -> (s? t:f=w236:dbl)
              n133 = Subtract(x=w236, y=w231) -> (x-y=w226:dbl)
              n134 = Less Or Equal?(x=w226, y=0) -> (x <= y?=w234:bool)
              n135 = property on="Status LED" class="Bool (strict)"("BoolText.Text"=w227) -> ()  [unwired: 2 in, 2 out]
              n136 = local write "Wait Countdown"(w226) -> ()
              n137 = node-c288() -> ()  [unwired: 1 in, 1 out]
            }
            n138 = node-c288(w224) -> ()  [unwired: 1 out]
          }
          frame #2 {
            n139 = local read "Transport"() -> (w247:bool)
            n140 = case shown="True" w247 {
              tunnel: w248 -> [_ w250]
              frame False {
              }
              frame True {
                n141 = stacked-sequence {
                  tunnel: w250 -> [w302 _]
                  tunnel: 0 -> [w301 _]
                  frame #0 {
                    # "SuperDuper w/o TPX"
                    n142 = local read "Dielectric Constant:"() -> (w254:dbl)
                    n143 = local read "Start 2"() -> (w294:dbl)
                    n144 = local read "Stop 2"() -> (w293:dbl)
                    n145 = local read "Step 2"() -> (w292:dbl)
                    n146 = local read "Start"() -> (w296:dbl)
                    n147 = local read "Step"() -> (w298:dbl)
                    n148 = local read "Var1 sweep settings 2"() -> (w277:T7)
                    n149 = local read "Stop 3"() -> (w284:dbl)
                    n150 = local read "Var1 sweep settings"() -> (w278:T7)
                    n151 = local read "Wait Countdown"() -> (w270:dbl)
                    n152 = local read "Var2 step settings 2"() -> (w275:T8)
                    n153 = local read "Start"() -> (w285:dbl)
                    n154 = local read "Start"() -> (w282:dbl)
                    n155 = local read "Step"() -> (w283:dbl)
                    n156 = local read "Step"() -> (w281:dbl)
                    n157 = local read "Var2 step settings"() -> (w276:T8)
                    n158 = local read "Wait Time (s)"() -> (w269:dbl)
                    n159 = local read "Integration Time 3"() -> (w290:u32)
                    n160 = local read "VISA resource name"() -> (w272:refnum<visa-resource-name>)
                    n161 = local read "Gated SMU4 is..."() -> (w251:bool)
                    n162 = local read "Integration Time"() -> (w279:u32)
                    n163 = local read "Total Points"() -> (w295:u16)
                    n164 = local read "# of Loops"() -> (w297:dbl)
                    n165 = local read "Loop Wait"() -> (w289:dbl)
                    n166 = local read "Loop Step"() -> (w291:dbl)
                    n167 = local read "First Step"() -> (w288:dbl)
                    n168 = local read "Total Points"() -> (w280:u16)
                    n169 = local read "Transport"() -> (w264:bool)
                    n170 = local read "Sample Properties:"() -> (w299:T4)
                    n171 = Bundle("Wait Countdown"=w270, "Wait Time (s)"=w269) -> (w268:T14)  [unwired: 1 in]
                    n172 = local read "Saved Folder:"() -> (w300:path)
                    n173 = Bundle("Step"=w298, "# of Loops"=w297, FALSE, "Start"=w296, "Total Points"=w295, "Start 2"=w294, "Stop 2"=w293, "Step 2"=w292, "Loop Step"=w291, "Integration Time 3"=w290, "Loop Wait"=w289, "First Step"=w288) -> (w287:T20)  [unwired: 1 in]
                    n174 = Bundle("Transport"=w264, "Start"=w285, "Stop 3"=w284, "Step"=w283, "Start"=w282, "Step"=w281, "Total Points"=w280, "Integration Time"=w279) -> (w286:T21)  [unwired: 1 in]
                    n175 = Bundle("Var1 sweep settings"=w278, "Var1 sweep settings 2"=w277, "Var2 step settings"=w276, "Var2 step settings 2"=w275) -> (w274:T17)  [unwired: 1 in]
                    n176 = local read "Gate Current Cluster"() -> (w253:T6)
                    n177 = local read "Stop \nCountdown"() -> (w273:bool)
                    n178 = call "Sub Super Duper_14_02_18_JWa.vi"("VISA resource name"=w272, "Sample Properties:"=w299, "Gated SMU4 is..."=w251, "TRF Cluster"=w287, "TSP Cluster"=w286, "Compliance Cluster"=w274, "error in"=w302, "Saved Folder:"=w300, "Wait Cluster"=w268, "Stop \nCountdown"=w273, "Loop Count"=w301, "Gate Current Cluster"=w253, "Dielectric Constant (BG)"=w254) -> ("Status Indicator"=w271:bool, "TRF Path"=w267:path, "TSP Path"=w266:path, "Graph Cluster"=w261:T18, "Char Cluster"=w255:T19)  [unwired: 7 in, 3 out]
                    n179 = Unbundle By Name(w261) -> ("Linear Transfer"=w260:cluster{dbl[], "trace":dbl[]}[], "Linear Raw"=w259:cluster{dbl[], dbl[]}[], "Saturation Transfer"=w258:cluster{dbl[], "trace":dbl[]}[], "Saturation Raw"=w257:cluster{dbl[], dbl[]}[], "Transport"=w256:cluster{dbl[], dbl[]}[], "TRF Gate Current"=w252:cluster{dbl[], dbl[]}[])
                    n180 = local write "Status LED"(w271) -> ()
                    n181 = property on="Status LED" class="Bool (strict)"("BoolText.Text"="Measuring\nTransport") -> ()  [unwired: 2 in, 2 out]
                    n182 = local write "Status LED"(TRUE) -> ()
                    n183 = local write "TRF Path"(w267) -> ()
                    n184 = local write "TSP Path"(w266) -> ()
                    n185 = local write "TSF Gate Current"(w252) -> ()
                    n186 = local write "Transport Graph"(w256) -> ()
                    n187 = local write "Saturation Raw"(w257) -> ()
                    n188 = local write "Linear Transfer"(w260) -> ()
                    n189 = local write "Saturation Transfer"(w258) -> ()
                    n190 = local write "Linear Raw"(w259) -> ()
                    n191 = Unbundle By Name(w255) -> ()  [unwired: 2 out]
                  }
                  frame #1 {
                    n192 = local write "Status LED"(FALSE) -> ()
                    n193 = property on="Status LED" class="Bool (strict)"("BoolText.Text"="Ready") -> ()  [unwired: 2 in, 2 out]
                  }
                }
              }
            }
          }
          frame #3 {
            n194 = local read "Light Bathe Cluster"() -> (w306:T2)
            n195 = Unbundle By Name(w306) -> ("Post Measure:"=w305:bool)
            n196 = local read "VISA resource name"() -> (w307:refnum<visa-resource-name>)
            n197 = case shown="True" w305 {
              tunnel: w307 -> [_ w309]
              frame False {
              }
              frame True {
                w310 = u32 1 items=["positive pulse  ", "negative pulse  ", "level high  ", "level low  "] ("trigger signal")
                n198 = local write "Light is..."(TRUE ("Light is...")) -> ()
                n199 = call "HP415xA Op-Trigger Output.vi"("trigger signal"=w310, "VISA session"=w309) -> ()  [unwired: 2 in, 1 out]
              }
            }
          }
        }
        n200 = Not(x="OK Button") -> (.not. x?=w96:bool)
      }
      event "Light Bathe Cluster.TG to BG (TRF):": Value Change {
        n201 = event-data() -> ()  [unwired: 1 in, 5 out]
        n202 = local read "Light Bathe Cluster"() -> (w312:T2)
        n203 = Unbundle By Name(w312) -> ("TG to BG (TRF):"=w311:bool)
        n204 = case shown="False" w311 {
          frame False {
            n205 = local write "Gated SMU4 is..."(FALSE ("Gated SMU4 is...")) -> ()
          }
          frame True {
            n206 = local write "Gated SMU4 is..."(TRUE ("Gated SMU4 is...")) -> ()
          }
        }
      }
      event "Light is...": Mouse Down {
        n207 = event-data() -> ()  [unwired: 1 in, 7 out]
        n208 = local read "Light Bathe Cluster"() -> (w317:T2)
        n209 = Bundle By Name(cluster=w317, "Post Measure:"=FALSE) -> (w315:T2)
        n210 = local write "Light Bathe Cluster"(w315) -> ()
        n211 = local read "Light is..."() -> (w319:bool)
        n212 = local read "VISA resource name"() -> (w318:refnum<visa-resource-name>)
        n213 = case shown="True" w319 {
          tunnel: w318 -> [w320 w322]
          frame False {
            w321 = u32 1 items=["positive pulse  ", "negative pulse  ", "level high  ", "level low  "] ("trigger signal")
            n214 = call "HP415xA Op-Trigger Output.vi"("trigger signal"=w321, "VISA session"=w320) -> ()  [unwired: 2 in, 1 out]
          }
          frame True {
            w323 = u32 0 items=["positive pulse  ", "negative pulse  ", "level high  ", "level low  "] ("trigger signal")
            n215 = call "HP415xA Op-Trigger Output.vi"("trigger signal"=w323, "VISA session"=w322) -> ()  [unwired: 2 in, 1 out]
          }
        }
      }
      event "TPX OK Button": Mouse Down {
        n216 = event-data() -> ()  [unwired: 1 in, 7 out]
        n217 = Initialize Array(w327) -> (w326:dbl[])  [unwired: 1 in]
        n218 = Initialize Array(0) -> (w325:i32[])  [unwired: 1 in]
        n219 = local write "Array 2"(w325) -> ()
        n220 = local write "Array"(w326) -> ()
        n221 = stacked-sequence {
          tunnel: [_ w409 _] -> w324
          frame #0 {
            w354 = "XXX"
            w335 = "TPX"
            n222 = local read "Start (K)"() -> (w337:dbl)
            n223 = local read "Saved Folder:"() -> (w368:path)
            n224 = local write "Current Step"(0) -> ()
            n225 = Build Path(base path=w368, name or relative path=w335) -> (appended path=w367:path)
            n226 = call <vilib>:"Check if File or Folder Exists.vi"("path"=w367) -> ("file or folder exists?"=w369:bool, "dup path"=w370:path)  [unwired: 8 in, 1 out]
            n227 = case shown="False" w369 {
              tunnel: w370 -> [w403 w404]
              tunnel: [w402 w404] -> w349
              frame False {
                n228 = Create Folder(path (use dialog)=w403) -> (created path=w402:path)  [unwired: 2 in, 2 out]
              }
              frame True {
              }
            }
            n229 = local read "Sample Properties:"() -> (w366:T4)
            n230 = Unbundle(w366) -> ("Index (#)"=w365:string, "Index (ABC)"=w364:string, "Length"=w357:string, "Width"=w352:string)  [unwired: 9 out]
            n231 = Concatenate Strings(w365, w364) -> (w363:string)
            n232 = Decimal String To Number(string=w357) -> (number=w360:i32)  [unwired: 2 in, 1 out]
            n233 = Decimal String To Number(string=w352) -> (number=w353:i32)  [unwired: 2 in, 1 out]
            n234 = Number To Decimal String(number=w360) -> (decimal integer string=w356:string)  [unwired: 1 in]
            n235 = Number To Decimal String(number=w353) -> (decimal integer string=w345:string)  [unwired: 1 in]
            n236 = Equal?(x=w356, y=w354) -> (x = y?=w361:bool)
            n237 = Equal?(x=w345, y=w354) -> (x = y?=w362:bool)
            n238 = Select(t=w354, s=w361, f=w356) -> (s? t:f=w355:string)
            n239 = Select(t=w354, s=w362, f=w345) -> (s? t:f=w351:string)
            n240 = Number To Decimal String(number=w337) -> (decimal integer string=w347:string)  [unwired: 1 in]
            n241 = local read "Stop (K)"() -> (w336:dbl)
            n242 = while {
              tunnel: w337 -> [w377]
              tunnel: w336 -> [w376]
              stop <- w371 continue-if-true
              n243 = local read "A: High Alarm"() -> (w381:dbl)
              n244 = Max & Min(x=w377, y=w376) -> (max(x,y)=w384:dbl)  [unwired: 1 out]
              n245 = Greater Or Equal?(x=w384, y=w381) -> (x >= y?=w371:bool)
              n246 = call "Prompt User for Input"("Enable"=w371) -> ("Stopping Temp"=w375:dbl, "Starting Temp"=w374:dbl, "High Alarm Value"=w382:dbl)  [unwired: 14 in, 2 out]
              n247 = Greater Than 0?(x=w382) -> (x > 0?=w383:bool)
              n248 = Greater Than 0?(x=w375) -> (x > 0?=w378:bool)
              n249 = Greater Than 0?(x=w374) -> (x > 0?=w379:bool)
              n250 = Select(t=w382, s=w383, f=w381) -> (s? t:f=w380:dbl)
              n251 = local write "A: High Alarm"(w380) -> ()
              n252 = Select(t=w375, s=w378, f=w376) -> (s? t:f=w372:dbl)
              n253 = local write "Stop (K)"(w372) -> ()
              n254 = Select(t=w374, s=w379, f=w377) -> (s? t:f=w373:dbl)
              n255 = local write "Start (K)"(w373) -> ()
            }
            n256 = Number To Decimal String(number=w336) -> (decimal integer string=w346:string)  [unwired: 1 in]
            n257 = call "Build Text4"("Start"=w347, "Index"=w363, "Length"=w355, "Width"=w351, "Stop"=w346) -> ("Result"=w350:string)  [unwired: 9 in, 1 out]
            n258 = Build Path(base path=w349, name or relative path=w350) -> (appended path=w348:path)
            n259 = call <vilib>:"Check if File or Folder Exists.vi"("path"=w348) -> ("file or folder exists?"=w359:bool, "dup path"=w358:path)  [unwired: 8 in, 1 out]
            n260 = case shown="True" w359 {
              tunnel: w358 -> [w388 w390]
              tunnel: [w388 w389] -> w341
              frame False {
              }
              frame True {
                n261 = while {
                  tunnel: w390 -> [w392]
                  tunnel: [w391] -> w389
                  i -> [w394]
                  stop <- w395 stop-if-true
                  n262 = Increment(x=w394) -> (x+1=w393:i32)
                  n263 = Path To String(path=w392) -> (string=w401:string)
                  n264 = Number To Decimal String(number=w393) -> (decimal integer string=w399:string)  [unwired: 1 in]
                  n265 = Concatenate Strings(w401, "_", w399) -> (w398:string)
                  n266 = String To Path(string=w398) -> (path=w397:path)
                  n267 = call <vilib>:"Check if File or Folder Exists.vi"("path"=w397) -> ("file or folder exists?"=w396:bool, "dup path"=w391:path)  [unwired: 8 in, 1 out]
                  n268 = Not(x=w396) -> (.not. x?=w395:bool)
                }
              }
            }
            n269 = local write "Temperature Measurements"(w341) -> ()
            n270 = Strip Path(path=w341) -> (stripped path=w333:path, name=w331:string)
            n271 = Search and Replace String(input string=w331, search string=w335, replace string="STATUS") -> (result string=w332:string)  [unwired: 5 in, 3 out]
            n272 = Build Path(base path=w333, name or relative path=w332) -> (appended path=w330:path)
            n273 = Search and Replace String(input string=w331, search string=w335, replace string="ELEC") -> (result string=w339:string)  [unwired: 5 in, 3 out]
            n274 = local write "Status"(w330) -> ()
            n275 = Build Path(base path=w333, name or relative path=w339) -> (appended path=w338:path)
            n276 = call <vilib>:"Check if File or Folder Exists.vi"("path"=w338) -> ("file or folder exists?"=w344:bool, "dup path"=w343:path)  [unwired: 8 in, 1 out]
            n277 = case shown="False" w344 {
              tunnel: w343 -> [w386 w387]
              tunnel: [w385 w387] -> w342
              frame False {
                n278 = Create Folder(path (use dialog)=w386) -> (created path=w385:path)  [unwired: 2 in, 2 out]
              }
              frame True {
              }
            }
            n279 = local write "Electrical Measurements"(w342) -> ()
          }
          frame #1 {
            n280 = local read "Reverse Scan (Y/N)"() -> (w406:bool)
            n281 = Select(t=1, s=w406, f=0) -> (s? t:f=w405:i32)
            n282 = while {
              tunnel: w405 -> [w417]
              i -> [w416]
              stop <- w412 continue-if-true
              n283 = local write "Repeat Loop"(w416) -> ()
              n284 = local read "Abort?"() -> (w414:bool)
              n285 = Not(x=w414) -> (.not. x?=w415:bool)
              n286 = Greater?(x=w417, y=w416) -> (0:w413:bool)
              n287 = And(x=w415, y=w413) -> (x .and. y?=w412:bool)
              n288 = stacked-sequence {
                frame #0 {
                  n289 = local read "Array 2"() -> (w420:i32[])
                  n290 = local read "Array"() -> (w421:i32[])
                  n291 = while {
                    shift-right: [w428] -> w419
                    shift-left: w421 -> [w430]
                    shift-right: [w427] -> w418
                    shift-left: w420 -> [w429]
                    stop <- w424 stop-if-true
                    n292 = local read "Current Step"() -> (w426:dbl)
                    n293 = local read "Abort?"() -> (w423:bool)
                    n294 = local read "# Steps"() -> (w422:dbl)
                    n295 = Less Or Equal?(x=w422, y=w426) -> (x <= y?=w425:bool)
                    n296 = Compound Arithmetic op=OR(w425, w423) -> (w424:bool)
                    n297 = stacked-sequence {
                      seq-local: [w491 _ _ _ _ _ _] -> [_ _ w595 _ _ _ _]
                      seq-local: [w490 _ _ _ _ _ _] -> [_ _ w594 _ _ _ _]
                      seq-local: [w489 _ _ _ _ _ _] -> [_ _ w593 _ _ _ _]
                      seq-local: [w471 _ _ _ _ _ _] -> [_ _ w586 _ _ _ _]
                      seq-local: [w472 _ _ _ _ _ _] -> [_ _ w585 _ _ _ _]
                      seq-local: [w451 _ _ _ _ _ _] -> [_ _ w584 _ _ _ _]
                      seq-local: [_ _ w592 _ _ _ _] -> [_ _ _ _ w790 _ _]
                      seq-local: [_ _ w591 _ _ _ _] -> [_ _ _ _ w788 _ _]
                      seq-local: [_ _ w590 _ _ _ _] -> [_ _ _ _ w793 _ _]
                      seq-local: [_ _ w588 _ _ _ _] -> [_ _ _ _ w786 _ _]
                      seq-local: [_ _ w587 _ _ _ _] -> [_ _ _ _ w785 _ _]
                      seq-local: [_ _ w583 _ _ _ _] -> [_ _ _ _ w782 _ _]
                      seq-local: [_ _ _ _ w792 _ _] -> [_ _ _ _ _ w987 _]
                      seq-local: [_ _ _ _ w791 _ _] -> [_ _ _ _ _ w986 _]
                      seq-local: [_ _ _ _ w787 _ _] -> [_ _ _ _ _ w985 _]
                      seq-local: [_ _ _ _ w784 _ _] -> [_ _ _ _ _ w984 _]
                      seq-local: [_ _ _ _ w783 _ _] -> [_ _ _ _ _ w983 _]
                      seq-local: [_ _ _ _ w781 _ _] -> [_ _ _ _ _ w982 _]
                      seq-local: [_ _ _ _ _ w990 _] -> [_ _ _ _ _ _ _]
                      seq-local: [_ _ _ _ _ w989 _] -> [_ _ _ _ _ _ w1053]
                      seq-local: [_ _ _ _ _ w988 _] -> [_ _ _ _ _ _ w1052]
                      seq-local: [_ _ _ _ _ w985 _] -> [_ _ _ _ _ _ w1050]
                      seq-local: [_ _ _ _ _ w984 _] -> [_ _ _ _ _ _ w1049]
                      seq-local: [_ _ _ _ _ w983 _] -> [_ _ _ _ _ _ w1048]
                      seq-local: [_ _ _ _ _ w982 _] -> [_ _ _ _ _ _ w1045]
                      tunnel: w426 -> [w449 _ _ _ _ _ _]
                      tunnel: w430 -> [w471 _ _ _ _ _ _]
                      tunnel: w429 -> [w472 _ _ _ _ _ _]
                      tunnel: [_ _ _ _ _ _ w1047] -> w428
                      tunnel: [_ _ _ _ _ _ w1046] -> w427
                      frame #0 {
                        # "This frame resets and configures the instrument for the rest\nof the frames."
                        n298 = local read "Sample Control"() -> (w492:bool)
                        n299 = local write "Current Step"(w449) -> ()
                        n300 = local read "Start Time Num"() -> (w464:dbl)
                        n301 = local read "Time Iteration (s)"() -> (w463:dbl)
                        n302 = call "Elapsed Time5"("Time Target (s)"=w463, "Auto Reset"=TRUE) -> ("Present (s)"=w465:dbl)  [unwired: 10 in, 7 out]
                        n303 = case shown="True" w492 {
                          tunnel: w449 -> [_ w552]
                          tunnel: [_ w533] -> w491
                          tunnel: [_ w527] -> w490
                          tunnel: [_ w542] -> w489
                          tunnel: [_ w500] -> w484
                          tunnel: [_ w530] -> w468
                          tunnel: [_ w529] -> w467
                          tunnel: [_ w528] -> w466
                          tunnel: [_ w498] -> w451
                          frame False {
                          }
                          frame True {
                            w497 = FALSE
                            w498 = 1
                            w501 = 2
                            w516 = TRUE
                            w547 = 1
                            w542 = 2
                            w550 = TRUE
                            n304 = local read "VISA Resource (TPX)"() -> (w540:refnum<visa-resource-name>)
                            n305 = local read "Start (K)"() -> (w554:dbl)
                            n306 = local read "Stop (K)"() -> (w557:dbl)
                            n307 = local read "# Steps"() -> (w555:dbl)
                            n308 = Subtract(x=w557, y=w554) -> (x-y=w556:dbl)
                            n309 = Divide(x=w556, y=w555) -> (x/y=w553:dbl)
                            n310 = Multiply(x=w553, y=w552) -> (x*y=w551:dbl)
                            n311 = Add(x=w554, y=w551) -> (x+y=w500:dbl)
                            n312 = local read "A: High Alarm"() -> (w494:dbl)
                            n313 = local write "Target"(w500) -> ()
                            n314 = local read "A:  Sample Stage"() -> (w496:dbl)
                            n315 = call "Reset Min and Max.vi"("Reset Min/Max Data (T: Yes)"=TRUE, "VISA resource name"=w540) -> ("error out"=w539:errorcluster, "VISA resource name out"=w536:refnum<visa-resource-name>)  [unwired: 8 in]
                            n316 = local write "SetPoint2\nOVR"(w500) -> ()
                            n317 = local read "A: Low Alarm"() -> (w493:dbl)
                            n318 = call "Configure Input Parameters.vi"("VISA resource name"=w536, "Input Name (\"\")"="Sample Stage", "Input (0:A)"=0, "Sensor Type and Range (0:Disabled)"=1, "error in (no error)"=w539, "Curve (0:None)"=2, "Temperature Limit (0)"=w494) -> ("VISA resource name out"=w565:refnum<visa-resource-name>, "error out"=w566:errorcluster)  [unwired: 7 in]
                            n319 = call "Configure Alarm.vi"("VISA resource name"=w565, "High Value (0.00000)"=w494, "Low Value (0.00000)"=w493, "Enable Alarm (F: Off)"=w550, "error in (no error)"=w566, "Enable Beep (F: Off)"=w550, "Enable Display (F: Off)"=w550) -> ("VISA resource name out"=w562:refnum<visa-resource-name>, "error out"=w561:errorcluster)  [unwired: 7 in]
                            n320 = call "Configure Heater Output.vi"("VISA resource name"=w562, "Mode (0:Off)"=w547, "Heater Output (1:1)"=w542, "Input (0:None)"=w547, "error in (no error)"=w561, "Heater Out Display (1:Current)"=2) -> ("VISA resource name out"=w559:refnum<visa-resource-name>, "error out"=w537:errorcluster)  [unwired: 8 in]
                            n321 = local read "Output 1 Range"() -> (w499:enum16{"Off", "Low (On)", "Medium", "High"})
                            n322 = local read "P 2"() -> (w504:dbl)
                            n323 = local read "D 2"() -> (w502:dbl)
                            n324 = local read "I 2"() -> (w503:dbl)
                            n325 = call "Configure PID.vi"("VISA resource name"=w559, "Output's Control Loop (1:1)"=w542, "Gain (P) (50.0)"=w504, "Reset (I) (20.0)"=w503, "error in (no error)"=w537, "Rate (D) (0.0 %)"=w502) -> ("VISA resource name out"=w535:refnum<visa-resource-name>, "error out"=w534:errorcluster)  [unwired: 8 in]
                            n326 = local read "Output 2 Range"() -> (w558:enum16{"Off", "Low (On)", "Medium", "High"})
                            n327 = local read "Rate (K/min)"() -> (w495:dbl)
                            n328 = Greater Than 0?(x=w495) -> (x > 0?=w523:bool)
                            n329 = Greater Than 0?(x=w495) -> (x > 0?=w541:bool)
                            n330 = call "Configure Setpoint and Ramp.vi"("VISA resource name"=w535, "Output's Control Loop (1:1)"=w542, "Setpoint (0.00000)"=w496, "Setpoint Ramping \nEnable (F: Off)"=w497, "error in (no error)"=w534) -> ("VISA resource name out"=w546:refnum<visa-resource-name>, "error out"=w545:errorcluster)  [unwired: 9 in]
                            n331 = call "Configure Setpoint and Ramp.vi"("VISA resource name"=w546, "Output's Control Loop (1:1)"=w542, "Setpoint (0.00000)"=w500, "Setpoint Ramping \nEnable (F: Off)"=w541, "error in (no error)"=w545, "Ramp Rate (0.0)"=w495) -> ("VISA resource name out"=w544:refnum<visa-resource-name>, "error out"=w543:errorcluster)  [unwired: 8 in]
                            n332 = call "Configure Output Range and Manual Value.vi"("VISA resource name"=w544, "Output (1:1)"=w542, "Range (0:Off)"=w558, "error in (no error)"=w543) -> ("VISA resource name out"=w506:refnum<visa-resource-name>, "error out"=w508:errorcluster)  [unwired: 10 in]
                            n333 = call "Configure Input Parameters.vi"("VISA resource name"=w506, "Input Name (\"\")"="Radiation Shield", "Input (0:A)"=1, "Sensor Type and Range (0:Disabled)"=1, "error in (no error)"=w508, "Curve (0:None)"=2, "Temperature Limit (0)"=w494) -> ("VISA resource name out"=w510:refnum<visa-resource-name>, "error out"=w509:errorcluster)  [unwired: 7 in]
                            n334 = call "Configure Alarm.vi"("VISA resource name"=w510, "High Value (0.00000)"=w494, "Low Value (0.00000)"=w493, "Input (0:A)"=w498, "Enable Alarm (F: Off)"=w516, "error in (no error)"=w509, "Enable Beep (F: Off)"=w516, "Enable Display (F: Off)"=w516) -> ("VISA resource name out"=w513:refnum<visa-resource-name>, "error out"=w514:errorcluster)  [unwired: 6 in]
                            n335 = call "Configure Heater Output.vi"("VISA resource name"=w513, "Mode (0:Off)"=w498, "Heater Output (1:1)"=w498, "Input (0:None)"=w501, "error in (no error)"=w514, "Heater Out Display (1:Current)"=w501) -> ("VISA resource name out"=w515:refnum<visa-resource-name>, "error out"=w524:errorcluster)  [unwired: 8 in]
                            n336 = call "Configure PID.vi"("VISA resource name"=w515, "Output's Control Loop (1:1)"=w498, "Gain (P) (50.0)"=w504, "Reset (I) (20.0)"=w503, "error in (no error)"=w524, "Rate (D) (0.0 %)"=w502) -> ("VISA resource name out"=w525:refnum<visa-resource-name>, "error out"=w526:errorcluster)  [unwired: 8 in]
                            n337 = call "Configure Setpoint and Ramp.vi"("VISA resource name"=w525, "Output's Control Loop (1:1)"=w498, "Setpoint (0.00000)"=w496, "Setpoint Ramping \nEnable (F: Off)"=w497, "error in (no error)"=w526) -> ("VISA resource name out"=w519:refnum<visa-resource-name>, "error out"=w520:errorcluster)  [unwired: 9 in]
                            n338 = call "Configure Setpoint and Ramp.vi"("VISA resource name"=w519, "Output's Control Loop (1:1)"=w498, "Setpoint (0.00000)"=w500, "Setpoint Ramping \nEnable (F: Off)"=w523, "error in (no error)"=w520, "Ramp Rate (0.0)"=w495) -> ("VISA resource name out"=w521:refnum<visa-resource-name>, "error out"=w522:errorcluster)  [unwired: 8 in]
                            n339 = call "Configure Output Range and Manual Value.vi"("VISA resource name"=w521, "Output (1:1)"=w498, "Range (0:Off)"=w499, "error in (no error)"=w522) -> ("VISA resource name out"=w505:refnum<visa-resource-name>, "error out"=w507:errorcluster)  [unwired: 10 in]
                            n340 = call "Lakeshore_monitor.vi"("error? 2"=w507, "VISA Resource (TPX)"=w505) -> ("error?"=w527:errorcluster, "Outputs"=w531:T12, "Inputs"=w532:T13, "VISA resource name"=w533:refnum<visa-resource-name>)  [unwired: 5 in]
                            n341 = Unbundle(w531) -> ()  [unwired: 19 out]
                            n342 = Unbundle(w532) -> ("A:  Sample Stage"=w530:dbl, "B:  Rad Shield"=w529:dbl, "B: Probe Arm"=w528:dbl)  [unwired: 2 out]
                          }
                        }
                        n343 = Subtract(x=w465, y=w464) -> (x-y=w461:dbl)
                        n344 = Number To Fractional String(number=w484) -> (F-format string=w482:string)  [unwired: 3 in]
                        n345 = Number To Decimal String(number=w449) -> (decimal integer string=w485:string)  [unwired: 1 in]
                        n346 = Bundle("Array 2"=w472, "Array"=w471) -> (w470:cluster{"Array 2":dbl[], "Array":dbl[]})  [unwired: 1 in]
                        n347 = local read "Temperature Measurements"() -> (w487:path)
                        n348 = Build Array(w470) -> (w469:cluster{"Array 2":dbl[], "Array":dbl[]}[])
                        n349 = local write "Temp Graph"(w469) -> ()
                        n350 = Build Array("Step #", w485, "Setpoint", w482) -> (w475:string[])
                        n351 = Build Array("Elapsed Time(s)", "A: Sample Stage (K)", "B: Rad Shield (K)", "C: Probe Arm (K)", "Time", "Date") -> (w474:string[])
                        n352 = Number To Fractional String(number=w468) -> (F-format string=w459:string)  [unwired: 3 in]
                        n353 = Number To Decimal String(number=w461) -> (decimal integer string=w454:string)  [unwired: 1 in]
                        n354 = Get Date/Time In Seconds() -> (seconds since 1Jan1904=w460:timestamp)
                        n355 = Number To Fractional String(number=w467) -> (F-format string=w456:string)  [unwired: 3 in]
                        n356 = Number To Fractional String(number=w466) -> (F-format string=w455:string)  [unwired: 3 in]
                        n357 = Get Date/Time In Seconds() -> (seconds since 1Jan1904=w442:timestamp)
                        n358 = local read "# Steps"() -> (w446:dbl)
                        n359 = Get Date/Time String(seconds (now)=w442, want seconds? (F)=TRUE) -> (time string=w444:string)  [unwired: 1 in, 1 out]
                        n360 = local read "Status Table"() -> (w438:string[][])
                        n361 = Number To Decimal String(number=w449) -> (decimal integer string=w448:string)  [unwired: 1 in]
                        n362 = Number To Decimal String(number=w446) -> (decimal integer string=w445:string)  [unwired: 1 in]
                        n363 = Concatenate Strings("Initializing loop #", w448, " of ", w445) -> (w439:string)
                        n364 = Build Array(w444, w439) -> (w437:string[])
                        n365 = Insert Into Array(array=w438, new element=w437) -> (w431:string[][])  [unwired: 2 in]
                        n366 = Array Size(array=w431) -> (size(s)=w440:i32[])
                        n367 = Get Date/Time String(seconds (now)=w460, want seconds? (F)=TRUE) -> (date string=w457:string, time string=w458:string)  [unwired: 1 in]
                        n368 = Build Array(w454, w459, w456, w455, w458, w457) -> (w452:string[])
                        n369 = Build Array(w475, w474, w452) -> (w473:string[][])
                        n370 = call-poly <vilib>:"Write To Spreadsheet File.vi"("append to file? (new file:F)"=TRUE, "2D data"=w473, "file path (dialog if empty)"=w487) -> ()  [unwired: 5 in, 1 out]
                        n371 = local read "Status"() -> (w436:path)
                        n372 = local write "Status Table"(w431) -> ()
                        n373 = Index Array(array=w440, index=0) -> (element=w433:i32)
                        n374 = Decrement(x=w433) -> (x-1=w432:i32)
                        n375 = Bundle(w432, 0) -> (w434:cluster{i32, i32})  [unwired: 1 in]
                        n376 = property on="Status Table" class="Tbl (strict)"("Index Values"=w434) -> ()  [unwired: 2 in, 2 out]
                        n377 = call-poly <vilib>:"Write To Spreadsheet File.vi"("2D data"=w431, "file path (dialog if empty)"=w436) -> ()  [unwired: 6 in, 1 out]
                      }
                      frame #1 {
                        n378 = local read "Target"() -> (w579:dbl)
                        n379 = Number To Fractional String(number=w579) -> (F-format string=w580:string)  [unwired: 3 in]
                        n380 = Get Date/Time In Seconds() -> (seconds since 1Jan1904=w575:timestamp)
                        n381 = Concatenate Strings("Starting Setpoint Ramping to ", w580) -> (w570:string)
                        n382 = Get Date/Time String(seconds (now)=w575, want seconds? (F)=TRUE) -> (time string=w577:string)  [unwired: 1 in, 1 out]
                        n383 = local read "Status Table"() -> (w572:string[][])
                        n384 = Build Array(w577, w570) -> (w571:string[])
                        n385 = call <vilib>:"Space Constant.vi"() -> ("String"=w578:string)
                        n386 = Array Size(array=w572) -> (size(s)=w573:i32[])
                        n387 = Insert Into Array(array=w572, new element=w571) -> (w569:string[][])  [unwired: 2 in]
                        n388 = Build Array(w578) -> (w581:string[])
                        n389 = local read "Status"() -> (w568:path)
                        n390 = Build Array (concatenate)(w569, w581) -> (w567:string[][])
                        n391 = Index Array(array=w573, index=0) -> ()  [unwired: 1 out]
                        n392 = local write "Status Table"(w567) -> ()
                        n393 = call-poly <vilib>:"Write To Spreadsheet File.vi"("2D data"=w567, "file path (dialog if empty)"=w568) -> ()  [unwired: 6 in, 1 out]
                      }
                      frame #2 {
                        # "Initilizes LabView variables to corespond to the\ncurrent instrument status."
                        n394 = local read "Abort?"() -> (w589:bool)
                        n395 = case shown="False" w589 {
                          tunnel: w595 -> [w609 w766]
                          tunnel: w594 -> [w608 w765]
                          tunnel: w593 -> [w607 w767]
                          tunnel: [w606 w765] -> w592
                          tunnel: [w605 w767] -> w591
                          tunnel: [w604 w766] -> w590
                          tunnel: [w603 _] -> w588
                          tunnel: [w602 _] -> w587
                          tunnel: w586 -> [w601 _]
                          tunnel: w585 -> [w600 _]
                          tunnel: w584 -> [w597 _]
                          tunnel: [w596 _] -> w583
                          frame False {
                            n396 = node-c288() -> (w599:T9)  [unwired: 4 in]
                            n397 = timed-loop {
                              tunnel: w609 -> [w680]
                              tunnel: w608 -> [w679]
                              tunnel: w607 -> [w666]
                              tunnel: [w641] -> w606
                              tunnel: [w666] -> w605
                              tunnel: [w642] -> w604
                              shift-right: [w669] -> w603
                              shift-left: w601 -> [w678]
                              shift-right: [w670] -> w602
                              shift-left: w600 -> [w674]
                              timing: w599 -> [_]
                              timing-out: [_] -> w598
                              tunnel: w597 -> [w636]
                              tunnel: [w636] -> w596
                              i -> [w631]
                              stop <- w690 stop-if-true
                              w645 = TRUE
                              n398 = node-c288() -> ()  [unwired: 1 in, 1 out]
                              n399 = local read "SetPoint2\nOVR"() -> (w653:dbl)
                              n400 = local read "Rate (K/min)"() -> (w637:dbl)
                              n401 = local read "Output 2 Range"() -> (w689:enum16{"Off", "Low (On)", "Medium", "High"})
                              n402 = local read "Output 1 Range"() -> (w654:enum16{"Off", "Low (On)", "Medium", "High"})
                              n403 = local read "Start Time Num"() -> (w676:dbl)
                              n404 = local read "Time Iteration (s)"() -> (w684:dbl)
                              n405 = local read "Target"() -> (w665:dbl)
                              n406 = call "Elapsed Time"("Time Target (s)"=w684, "Auto Reset"=TRUE) -> ("Present (s)"=w675:dbl, "Time has Elapsed"=w686:bool)  [unwired: 10 in, 6 out]
                              n407 = call "Lakeshore_monitor.vi"("error? 2"=w679, "VISA Resource (TPX)"=w680) -> ("error?"=w687:errorcluster, "Outputs"=w696:T12, "Inputs"=w697:T13, "VISA resource name"=w688:refnum<visa-resource-name>)  [unwired: 5 in]
                              n408 = Unbundle(w696) -> ("P"=w698:dbl, "I"=w699:dbl, "D"=w700:dbl, "SetPoint Out2"=w701:dbl, "1"=w702:bool, "2"=w703:bool, "output control loop"=w704:dbl, "AutoTune Error"=w705:bool, "AutoTune Active"=w706:bool, "AutoTune Stage"=w707:dbl, "Out1 Active"=w708:bool, "Out1 Ramp On"=w709:bool, "Out2 Active"=w692:bool, "Out2 Ramp On"=w693:bool, "Heater 2 Output 1"=w710:dbl, "Heater 1 Output 2"=w713:dbl, "Out1 Ramp"=w711:dbl, "Out2 Ramp"=w712:dbl)  [unwired: 1 out]
                              n409 = Unbundle(w697) -> ("A:  Sample Stage"=w677:dbl, "B:  Rad Shield"=w683:dbl, "B: Probe Arm"=w682:dbl, "Temp Max Alarm"=w695:bool, "Temp Min Alarm"=w694:bool)
                              n410 = Build Array (concatenate)(w678, w677) -> (w669:dbl[])
                              n411 = local write "A:  Sample Stage"(w677) -> ()
                              n412 = local write "1"(w702) -> ()
                              n413 = local write "AutoTune Error"(w705) -> ()
                              n414 = local write "B:  Rad Shield"(w683) -> ()
                              n415 = Subtract(x=w675, y=w676) -> (x-y=w673:dbl)
                              n416 = Build Array (concatenate)(w674, w673) -> (w670:dbl[])
                              n417 = local write "Temp Max Alarm"(w695) -> ()
                              n418 = local write "Temp Min Alarm"(w694) -> ()
                              n419 = local write "P"(w698) -> ()
                              n420 = local write "C:  Probe Arm"(w682) -> ()
                              n421 = local write "Heater 1 Output2"(w713) -> ()
                              n422 = local write "AutoTune Stage"(w707) -> ()
                              n423 = local write "Heater 2 Output1"(w710) -> ()
                              n424 = local write "Out2 Ramp"(w712) -> ()
                              n425 = event shown="[3] \"Abort?\": Value Change" {
                                selector: _ -> [_ _ _ _]
                                dyn-events: _ -> [_ _ _ _]
                                timeout: 100 -> [_ _ _ _]
                                tunnel: [_ _ _ TRUE] -> _
                                tunnel: w680 -> [_ w742 w744 _]
                                tunnel: w679 -> [_ w741 w743 _]
                                event Timeout {
                                n426 = event-data() -> ()  [unwired: 1 in, 2 out]
                                }
                                event "Reset": Value Change {
                                n427 = event-data() -> ()  [unwired: 1 in, 5 out]
                                n428 = call "Reset Alarm.vi"("error in (no error)"=w741, "VISA resource name"=w742) -> ()  [unwired: 8 in, 2 out]
                                }
                                event "Alarm Reset 2": Value Change {
                                n429 = event-data() -> ()  [unwired: 1 in, 5 out]
                                n430 = call "Reset Alarm.vi"("error in (no error)"=w743, "VISA resource name"=w744) -> ()  [unwired: 8 in, 2 out]
                                }
                                event "Abort?": Value Change {
                                n431 = event-data() -> ()  [unwired: 1 in, 6 out]
                                }
                              }
                              n432 = local write "Out1 Ramp"(w711) -> ()
                              n433 = local write "2"(w703) -> ()
                              n434 = Not Equal?(x=w653, y=w665) -> (x != y?=w664:bool)
                              n435 = local write "I"(w699) -> ()
                              n436 = local write "output control loop"(w704) -> ()
                              n437 = Bundle(w670, w669) -> (w671:cluster{dbl[], dbl[]})  [unwired: 1 in]
                              n438 = local write "Setpoint (K)"(w701) -> ()
                              n439 = local write "D"(w700) -> ()
                              n440 = case shown="True" w664 {
                                tunnel: w688 -> [w728 w738]
                                tunnel: w687 -> [w727 w737]
                                tunnel: [w728 w732] -> w668
                                tunnel: [w727 w730] -> w667
                                tunnel: w666 -> [_ w736]
                                tunnel: w653 -> [_ w734]
                                tunnel: w653 -> [_ w735]
                                tunnel: w636 -> [_ w729]
                                frame False {
                                }
                                frame True {
                                n441 = local write "Target"(w735) -> ()
                                n442 = call "Configure Setpoint and Ramp.vi"("VISA resource name"=w738, "Output's Control Loop (1:1)"=w736, "Setpoint (0.00000)"=w734, "error in (no error)"=w737) -> ("VISA resource name out"=w733:refnum<visa-resource-name>, "error out"=w731:errorcluster)  [unwired: 10 in]
                                n443 = call "Configure Setpoint and Ramp.vi"("VISA resource name"=w733, "Output's Control Loop (1:1)"=w729, "Setpoint (0.00000)"=w734, "error in (no error)"=w731) -> ("VISA resource name out"=w732:refnum<visa-resource-name>, "error out"=w730:errorcluster)  [unwired: 10 in]
                                }
                              }
                              n444 = local read "A: Low Alarm"() -> (w650:dbl)
                              n445 = local write "AutoTune Active"(w706) -> ()
                              n446 = local read "A: High Alarm"() -> (w651:dbl)
                              n447 = Build Array(w671) -> (w672:cluster{dbl[], dbl[]}[])
                              n448 = Not(x=w692) -> (.not. x?=w714:bool)
                              n449 = local read "Abort?"() -> (w610:bool)
                              n450 = Compound Arithmetic op=OR(w695, w694, w610) -> (w613:bool)
                              n451 = local write "Elapsed Time"(w673) -> ()
                              n452 = Greater Than 0?(x=w637) -> (x > 0?=w652:bool)
                              n453 = local write "Temp Graph"(w672) -> ()
                              n454 = And(x=w693, y=w714) -> (x .and. y?=w691:bool)
                              n455 = local write "Out 2\nRamp On"(w693) -> ()
                              n456 = local write "Out 2\nActive"(w692) -> ()
                              n457 = local write "Out 1\nRamp On"(w709) -> ()
                              n458 = local write "Out 1\nActive"(w708) -> ()
                              n459 = call "Configure Setpoint and Ramp.vi"("VISA resource name"=w668, "Output's Control Loop (1:1)"=w666, "Setpoint (0.00000)"=w653, "Setpoint Ramping \nEnable (F: Off)"=w652, "error in (no error)"=w667, "Ramp Rate (0.0)"=w637) -> ("VISA resource name out"=w662:refnum<visa-resource-name>, "error out"=w661:errorcluster)  [unwired: 8 in]
                              n460 = local write "Abort?"(w613) -> ()
                              n461 = Or(x=w691, y=w610) -> (x .or. y?=w690:bool)
                              n462 = local read "Out 2\nRamp On"() -> (w611:bool)
                              n463 = local read "Out 1\nRamp On"() -> (w612:bool)
                              n464 = call "Configure Setpoint and Ramp.vi"("VISA resource name"=w662, "Output's Control Loop (1:1)"=w636, "Setpoint (0.00000)"=w653, "Setpoint Ramping \nEnable (F: Off)"=w652, "error in (no error)"=w661, "Ramp Rate (0.0)"=w637) -> ("VISA resource name out"=w659:refnum<visa-resource-name>, "error out"=w660:errorcluster)  [unwired: 8 in]
                              n465 = call "Configure Output Range and Manual Value.vi"("VISA resource name"=w659, "Output (1:1)"=w666, "Range (0:Off)"=w689, "error in (no error)"=w660) -> ("VISA resource name out"=w658:refnum<visa-resource-name>, "error out"=w657:errorcluster)  [unwired: 10 in]
                              n466 = call "Configure Output Range and Manual Value.vi"("VISA resource name"=w658, "Output (1:1)"=w636, "Range (0:Off)"=w654, "error in (no error)"=w657) -> ("VISA resource name out"=w656:refnum<visa-resource-name>, "error out"=w655:errorcluster)  [unwired: 10 in]
                              n467 = call "Configure Alarm.vi"("VISA resource name"=w656, "High Value (0.00000)"=w651, "Low Value (0.00000)"=w650, "Enable Alarm (F: Off)"=w645, "Enable Latching (F: Off)"=w645, "error in (no error)"=w655, "Enable Beep (F: Off)"=w645, "Enable Display (F: Off)"=w613) -> ("VISA resource name out"=w649:refnum<visa-resource-name>, "error out"=w648:errorcluster)  [unwired: 6 in]
                              n468 = local read "P 2"() -> (w640:dbl)
                              n469 = local read "D 2"() -> (w638:dbl)
                              n470 = call "Configure Alarm.vi"("VISA resource name"=w649, "High Value (0.00000)"=w651, "Low Value (0.00000)"=w650, "Input (0:A)"=w636, "Enable Alarm (F: Off)"=w645, "Enable Latching (F: Off)"=w645, "error in (no error)"=w648, "Enable Beep (F: Off)"=w645, "Enable Display (F: Off)"=w613) -> ("VISA resource name out"=w647:refnum<visa-resource-name>, "error out"=w646:errorcluster)  [unwired: 5 in]
                              n471 = local read "I 2"() -> (w639:dbl)
                              n472 = call "Configure PID.vi"("VISA resource name"=w647, "Output's Control Loop (1:1)"=2, "Gain (P) (50.0)"=w640, "Reset (I) (20.0)"=w639, "error in (no error)"=w646, "Rate (D) (0.0 %)"=w638) -> ("VISA resource name out"=w643:refnum<visa-resource-name>, "error out"=w644:errorcluster)  [unwired: 8 in]
                              n473 = case shown="True" w612 {
                                frame False {
                                n474 = property on="1" class="Bool (strict)"("BoolText.Text"="") -> ()  [unwired: 2 in, 2 out]
                                }
                                frame True {
                                n475 = local read "Out 1\nActive"() -> (w720:bool)
                                n476 = case shown="False" w720 {
                                frame False {
                                n477 = property on="1" class="Bool (strict)"("BoolText.Text"="Ramp\nOn") -> ()  [unwired: 2 in, 2 out]
                                }
                                frame True {
                                n478 = property on="1" class="Bool (strict)"("BoolText.Text"="Ramp\nActive") -> ()  [unwired: 2 in, 2 out]
                                }
                                }
                                }
                              }
                              n479 = case shown="False" w611 {
                                frame False {
                                n480 = property on="2" class="Bool (strict)"("BoolText.Text"="") -> ()  [unwired: 2 in, 2 out]
                                }
                                frame True {
                                n481 = local read "Out 2\nActive"() -> (w716:bool)
                                n482 = case shown="True" w716 {
                                frame False {
                                n483 = property on="2" class="Bool (strict)"("BoolText.Text"="Ramp\nOn") -> ()  [unwired: 2 in, 2 out]
                                }
                                frame True {
                                n484 = property on="2" class="Bool (strict)"("BoolText.Text"="Ramp\nActive") -> ()  [unwired: 2 in, 2 out]
                                }
                                }
                                }
                              }
                              n485 = call "Configure PID.vi"("VISA resource name"=w643, "Gain (P) (50.0)"=w640, "Reset (I) (20.0)"=w639, "error in (no error)"=w644, "Rate (D) (0.0 %)"=w638) -> ("VISA resource name out"=w642:refnum<visa-resource-name>, "error out"=w641:errorcluster)  [unwired: 9 in]
                              n486 = Quotient & Remainder(x=w631, y=3) -> (x-y*floor(x/y)=w634:i32)  [unwired: 1 out]
                              n487 = Get Date/Time In Seconds() -> (seconds since 1Jan1904=w622:timestamp)
                              n488 = case shown="0, Default" w634 {
                                tunnel: ["." ".." "..."] -> w633
                                frame 0, Default {
                                }
                                frame 1 {
                                }
                                frame 2 {
                                }
                              }
                              n489 = Get Date/Time String(seconds (now)=w622, want seconds? (F)=TRUE) -> (time string=w624:string)  [unwired: 1 in, 1 out]
                              n490 = local read "Status Table"() -> (w619:string[][])
                              n491 = local read "User's Name"() -> (w629:u16)
                              n492 = Concatenate Strings("Ramping", w633) -> (w615:string)
                              n493 = Build Array(w624, w615) -> (w618:string[])
                              n494 = local read "Text Editor Location"() -> (w627:path)
                              n495 = local read "Name/Email List Location"() -> (w628:path)
                              n496 = local read "Edit Users"() -> (w625:bool)
                              n497 = Array Size(array=w619) -> (size(s)=w620:i32[])
                              n498 = Index Array(array=w620, index=0) -> (element=w617:i32)
                              n499 = call "Email_List_subvi.vi"("Open File"=w625, "Name Ring In"=w629, "List Location"=w628, "Text Editor Location"=w627) -> ("String"=w630:string, "Names Out"=w626:string[])  [unwired: 5 in, 1 out]
                              n500 = case shown="True" w625 {
                                frame False {
                                }
                                frame True {
                                n501 = local write "Edit Users"(FALSE) -> ()
                                }
                              }
                              n502 = Decrement(x=w617) -> (x-1=w616:i32)
                              n503 = Replace Array Subset(array=w619, new element=w618, index (row)=w616) -> (w614:string[][])  [unwired: 1 in]
                              n504 = case shown="True" w686 {
                                tunnel: w677 -> [_ w761]
                                tunnel: w673 -> [_ w750]
                                tunnel: w683 -> [_ w754]
                                tunnel: w682 -> [_ w751]
                                tunnel: w614 -> [_ w746]
                                frame False {
                                }
                                frame True {
                                n505 = local read "Temperature Measurements"() -> (w762:path)
                                n506 = Number To Fractional String(number=w761) -> (F-format string=w757:string)  [unwired: 3 in]
                                n507 = Number To Decimal String(number=w750) -> (decimal integer string=w749:string)  [unwired: 1 in]
                                n508 = Get Date/Time In Seconds() -> (seconds since 1Jan1904=w758:timestamp)
                                n509 = Number To Fractional String(number=w754) -> (F-format string=w753:string)  [unwired: 3 in]
                                n510 = Number To Fractional String(number=w751) -> (F-format string=w752:string)  [unwired: 3 in]
                                n511 = Get Date/Time String(seconds (now)=w758, want seconds? (F)=TRUE) -> (date string=w755:string, time string=w756:string)  [unwired: 1 in]
                                n512 = Build Array(w749, w757, w753, w752, w756, w755) -> (w760:string[])
                                n513 = local read "Status"() -> (w747:path)
                                n514 = call-poly <vilib>:"Write To Spreadsheet File.vi"("append to file? (new file:F)"=TRUE, "1D data"=w760, "file path (dialog if empty)"=w762) -> ()  [unwired: 5 in, 1 out]
                                n515 = call-poly <vilib>:"Write To Spreadsheet File.vi"("2D data"=w746, "file path (dialog if empty)"=w747) -> ()  [unwired: 6 in, 1 out]
                                }
                              }
                              n516 = local write "Status Table"(w614) -> ()
                              n517 = local write "User's Email"(w630) -> ()
                              n518 = property on="User's Name" class="Ring (strict)"("Strings []"=w626) -> ()  [unwired: 2 in, 2 out]
                              n519 = node-c288() -> ()  [unwired: 1 in, 1 out]
                            }
                            n520 = node-c288(w598) -> ()  [unwired: 1 out]
                          }
                          frame True {
                          }
                        }
                      }
                      frame #3 {
                        n521 = Get Date/Time In Seconds() -> (seconds since 1Jan1904=w776:timestamp)
                        n522 = Get Date/Time String(seconds (now)=w776, want seconds? (F)=TRUE) -> (time string=w778:string)  [unwired: 1 in, 1 out]
                        n523 = local read "Status Table"() -> (w773:string[][])
                        n524 = Build Array(w778, "Ramping Complete") -> (w772:string[])
                        n525 = call <vilib>:"Space Constant.vi"() -> ("String"=w779:string)
                        n526 = Array Size(array=w773) -> (size(s)=w774:i32[])
                        n527 = Insert Into Array(array=w773, new element=w772) -> (w770:string[][])  [unwired: 2 in]
                        n528 = Build Array(w779) -> (w780:string[])
                        n529 = local read "Status"() -> (w769:path)
                        n530 = Build Array (concatenate)(w770, w780) -> (w768:string[][])
                        n531 = Index Array(array=w774, index=0) -> ()  [unwired: 1 out]
                        n532 = local write "Status Table"(w768) -> ()
                        n533 = call-poly <vilib>:"Write To Spreadsheet File.vi"("2D data"=w768, "file path (dialog if empty)"=w769) -> ()  [unwired: 6 in, 1 out]
                      }
                      frame #4 {
                        n534 = local read "Abort?"() -> (w789:bool)
                        n535 = case shown="False" w789 {
                          tunnel: w793 -> [w800 w967]
                          tunnel: [w805 w967] -> w792
                          tunnel: [w804 w966] -> w791
                          tunnel: w790 -> [w801 w966]
                          tunnel: w788 -> [w803 _]
                          tunnel: [w802 _] -> w787
                          tunnel: w786 -> [w799 _]
                          tunnel: w785 -> [w798 _]
                          tunnel: [w797 _] -> w784
                          tunnel: [w796 _] -> w783
                          tunnel: w782 -> [w795 _]
                          tunnel: [w794 _] -> w781
                          frame False {
                            n536 = node-c288() -> (w807:T9)  [unwired: 4 in]
                            n537 = timed-loop {
                              tunnel: w800 -> [w892]
                              timing: w807 -> [_]
                              timing-out: [_] -> w806
                              tunnel: [w842] -> w805
                              tunnel: [w841] -> w804
                              tunnel: w801 -> [w891]
                              tunnel: w803 -> [w864]
                              tunnel: [w864] -> w802
                              tunnel: w801 -> [w881]
                              tunnel: w800 -> [w880]
                              shift-right: [w872] -> w797
                              shift-left: w799 -> [w877]
                              shift-right: [w871] -> w796
                              shift-left: w798 -> [w876]
                              tunnel: w795 -> [w837]
                              tunnel: [w837] -> w794
                              i -> [w831]
                              stop <- w889 stop-if-true
                              n538 = node-c288() -> ()  [unwired: 1 in, 1 out]
                              n539 = local read "SetPoint2\nOVR"() -> (w857:dbl)
                              n540 = local read "Rate (K/min)"() -> (w856:dbl)
                              n541 = local read "Time Iteration (s)"() -> (w887:dbl)
                              n542 = local read "Start Time Num"() -> (w879:dbl)
                              n543 = call "Lakeshore_monitor.vi"("error? 2"=w891, "VISA Resource (TPX)"=w892) -> ("error?"=w868:errorcluster, "Outputs"=w910:T12, "Inputs"=w909:T13, "VISA resource name"=w869:refnum<visa-resource-name>)  [unwired: 5 in]
                              n544 = Unbundle(w910) -> ("P"=w908:dbl, "I"=w907:dbl, "D"=w906:dbl, "SetPoint Out2"=w905:dbl, "1"=w904:bool, "2"=w903:bool, "output control loop"=w902:dbl, "AutoTune Error"=w901:bool, "AutoTune Active"=w900:bool, "AutoTune Stage"=w899:dbl, "Out1 Active"=w898:bool, "Out1 Ramp On"=w897:bool, "Out2 Active"=w912:bool, "Out2 Ramp On"=w911:bool, "Heater 2 Output 1"=w896:dbl, "Heater 1 Output 2"=w893:dbl, "Out1 Ramp"=w895:dbl, "Out2 Ramp"=w894:dbl)  [unwired: 1 out]
                              n545 = Unbundle(w909) -> ("A:  Sample Stage"=w875:dbl, "B:  Rad Shield"=w884:dbl, "B: Probe Arm"=w883:dbl, "Temp Max Alarm"=w813:bool, "Temp Min Alarm"=w812:bool)
                              n546 = call "Elapsed Time2"("Time Target (s)"=w887, "Auto Reset"=TRUE) -> ("Present (s)"=w878:dbl, "Time has Elapsed"=w885:bool)  [unwired: 10 in, 6 out]
                              n547 = local read "Target"() -> (w866:dbl)
                              n548 = local write "A:  Sample Stage"(w875) -> ()
                              n549 = local write "1"(w904) -> ()
                              n550 = local write "AutoTune Error"(w901) -> ()
                              n551 = Build Array (concatenate)(w877, w875) -> (w872:dbl[])
                              n552 = local write "B:  Rad Shield"(w884) -> ()
                              n553 = local write "Temp Max Alarm"(w813) -> ()
                              n554 = local write "Temp Min Alarm"(w812) -> ()
                              n555 = local write "P"(w908) -> ()
                              n556 = event shown="[0] Timeout" {
                                selector: _ -> [_ _ _ _]
                                dyn-events: _ -> [_ _ _ _]
                                timeout: 100 -> [_ _ _ _]
                                tunnel: [_ _ _ TRUE] -> _
                                tunnel: w880 -> [_ w941 w943 _]
                                tunnel: w881 -> [_ w940 w942 _]
                                event Timeout {
                                n557 = event-data() -> ()  [unwired: 1 in, 2 out]
                                }
                                event "Reset": Value Change {
                                n558 = event-data() -> ()  [unwired: 1 in, 5 out]
                                n559 = call "Reset Alarm.vi"("error in (no error)"=w940, "VISA resource name"=w941) -> ()  [unwired: 8 in, 2 out]
                                }
                                event "Alarm Reset 2": Value Change {
                                n560 = event-data() -> ()  [unwired: 1 in, 5 out]
                                n561 = call "Reset Alarm.vi"("error in (no error)"=w942, "VISA resource name"=w943) -> ()  [unwired: 8 in, 2 out]
                                }
                                event "Abort?": Value Change {
                                n562 = event-data() -> ()  [unwired: 1 in, 6 out]
                                }
                              }
                              n563 = local write "C:  Probe Arm"(w883) -> ()
                              n564 = local read "Setpoint Tolerance (K)"() -> (w915:dbl)
                              n565 = local write "Heater 1 Output2"(w893) -> ()
                              n566 = local write "AutoTune Stage"(w899) -> ()
                              n567 = local write "Heater 2 Output1"(w896) -> ()
                              n568 = local write "Out2 Ramp"(w894) -> ()
                              n569 = local write "Out1 Ramp"(w895) -> ()
                              n570 = Subtract(x=w878, y=w879) -> (x-y=w862:dbl)
                              n571 = Build Array (concatenate)(w876, w862) -> (w871:dbl[])
                              n572 = Not Equal?(x=w866, y=w857) -> (x != y?=w870:bool)
                              n573 = local write "2"(w903) -> ()
                              n574 = local write "I"(w907) -> ()
                              n575 = local write "output control loop"(w902) -> ()
                              n576 = local write "Setpoint (K)"(w905) -> ()
                              n577 = case shown="True" w870 {
                                tunnel: w869 -> [w930 w939]
                                tunnel: w868 -> [w929 w938]
                                tunnel: [w930 w934] -> w865
                                tunnel: [w929 w933] -> w867
                                tunnel: w857 -> [_ w932]
                                tunnel: w864 -> [_ w937]
                                tunnel: w837 -> [_ w931]
                                frame False {
                                }
                                frame True {
                                n578 = local write "Target"(w932) -> ()
                                n579 = call "Configure Setpoint and Ramp.vi"("VISA resource name"=w939, "Output's Control Loop (1:1)"=w937, "Setpoint (0.00000)"=w932, "error in (no error)"=w938) -> ("VISA resource name out"=w936:refnum<visa-resource-name>, "error out"=w935:errorcluster)  [unwired: 10 in]
                                n580 = call "Configure Setpoint and Ramp.vi"("VISA resource name"=w936, "Output's Control Loop (1:1)"=w931, "Setpoint (0.00000)"=w932, "error in (no error)"=w935) -> ("VISA resource name out"=w934:refnum<visa-resource-name>, "error out"=w933:errorcluster)  [unwired: 10 in]
                                }
                              }
                              n581 = local read "Output 1 Range"() -> (w855:enum16{"Off", "Low (On)", "Medium", "High"})
                              n582 = local read "Output 2 Range"() -> (w888:enum16{"Off", "Low (On)", "Medium", "High"})
                              n583 = local write "D"(w906) -> ()
                              n584 = local write "AutoTune Active"(w900) -> ()
                              n585 = Bundle(w871, w872) -> (w874:cluster{dbl[], dbl[]})  [unwired: 1 in]
                              n586 = local read "Target"() -> (w916:dbl)
                              n587 = local read "Abort?"() -> (w808:bool)
                              n588 = Build Array(w874) -> (w873:cluster{dbl[], dbl[]}[])
                              n589 = Compound Arithmetic op=OR(w813, w812, w808) -> (w811:bool)
                              n590 = local read "A: Low Alarm"() -> (w845:dbl)
                              n591 = local read "A: High Alarm"() -> (w846:dbl)
                              n592 = local write "Elapsed Time"(w862) -> ()
                              n593 = Greater Than 0?(x=w856) -> (x > 0?=w836:bool)
                              n594 = Subtract(x=w916, y=w915) -> (x-y=w913:dbl)
                              n595 = Add(x=w916, y=w915) -> (x+y=w914:dbl)
                              n596 = local write "Temp Graph"(w873) -> ()
                              n597 = local write "Out 2\nRamp On"(w911) -> ()
                              n598 = local write "Out 2\nActive"(w912) -> ()
                              n599 = local write "Out 1\nRamp On"(w897) -> ()
                              n600 = local write "Out 1\nActive"(w898) -> ()
                              n601 = local write "Settle Time (s)"(w862) -> ()
                              n602 = In Range and Coerce(upper limit=w914, x=w875, lower limit=w913) -> (In Range?=w890:bool)  [unwired: 1 out]
                              n603 = call "Configure Setpoint and Ramp.vi"("VISA resource name"=w865, "Output's Control Loop (1:1)"=w864, "Setpoint (0.00000)"=w857, "Setpoint Ramping \nEnable (F: Off)"=w836, "error in (no error)"=w867, "Ramp Rate (0.0)"=w856) -> ("VISA resource name out"=w861:refnum<visa-resource-name>, "error out"=w860:errorcluster)  [unwired: 8 in]
                              n604 = Or(x=w890, y=w808) -> (x .or. y?=w889:bool)
                              n605 = local read "Out 2\nRamp On"() -> (w809:bool)
                              n606 = local read "Out 1\nRamp On"() -> (w810:bool)
                              n607 = call "Configure Setpoint and Ramp.vi"("VISA resource name"=w861, "Output's Control Loop (1:1)"=w837, "Setpoint (0.00000)"=w857, "Setpoint Ramping \nEnable (F: Off)"=w836, "error in (no error)"=w860, "Ramp Rate (0.0)"=w856) -> ("VISA resource name out"=w859:refnum<visa-resource-name>, "error out"=w858:errorcluster)  [unwired: 8 in]
                              n608 = call "Configure Output Range and Manual Value.vi"("VISA resource name"=w859, "Output (1:1)"=w864, "Range (0:Off)"=w888, "error in (no error)"=w858) -> ("VISA resource name out"=w854:refnum<visa-resource-name>, "error out"=w853:errorcluster)  [unwired: 10 in]
                              n609 = call "Configure Output Range and Manual Value.vi"("VISA resource name"=w854, "Output (1:1)"=w837, "Range (0:Off)"=w855, "error in (no error)"=w853) -> ("VISA resource name out"=w852:refnum<visa-resource-name>, "error out"=w851:errorcluster)  [unwired: 10 in]
                              n610 = call "Configure Alarm.vi"("VISA resource name"=w852, "High Value (0.00000)"=w846, "Low Value (0.00000)"=w845, "error in (no error)"=w851) -> ("VISA resource name out"=w850:refnum<visa-resource-name>, "error out"=w849:errorcluster)  [unwired: 10 in]
                              n611 = local write "Abort?"(w811) -> ()
                              n612 = case shown="True" w810 {
                                frame False {
                                n613 = property on="1" class="Bool (strict)"("BoolText.Text"="") -> ()  [unwired: 2 in, 2 out]
                                }
                                frame True {
                                n614 = local read "Out 1\nActive"() -> (w922:bool)
                                n615 = case shown="False" w922 {
                                frame False {
                                n616 = property on="1" class="Bool (strict)"("BoolText.Text"="Ramp\nOn") -> ()  [unwired: 2 in, 2 out]
                                }
                                frame True {
                                n617 = property on="1" class="Bool (strict)"("BoolText.Text"="Ramp\nActive") -> ()  [unwired: 2 in, 2 out]
                                }
                                }
                                }
                              }
                              n618 = case shown="False" w809 {
                                frame False {
                                n619 = property on="2" class="Bool (strict)"("BoolText.Text"="") -> ()  [unwired: 2 in, 2 out]
                                }
                                frame True {
                                n620 = local read "Out 2\nActive"() -> (w918:bool)
                                n621 = case shown="True" w918 {
                                frame False {
                                n622 = property on="2" class="Bool (strict)"("BoolText.Text"="Ramp\nOn") -> ()  [unwired: 2 in, 2 out]
                                }
                                frame True {
                                n623 = property on="2" class="Bool (strict)"("BoolText.Text"="Ramp\nActive") -> ()  [unwired: 2 in, 2 out]
                                }
                                }
                                }
                              }
                              n624 = local read "P 2"() -> (w840:dbl)
                              n625 = local read "D 2"() -> (w838:dbl)
                              n626 = call "Configure Alarm.vi"("VISA resource name"=w850, "High Value (0.00000)"=w846, "Low Value (0.00000)"=w845, "Input (0:A)"=w837, "error in (no error)"=w849) -> ("VISA resource name out"=w848:refnum<visa-resource-name>, "error out"=w847:errorcluster)  [unwired: 9 in]
                              n627 = local read "I 2"() -> (w839:dbl)
                              n628 = call "Configure PID.vi"("VISA resource name"=w848, "Output's Control Loop (1:1)"=2, "Gain (P) (50.0)"=w840, "Reset (I) (20.0)"=w839, "error in (no error)"=w847, "Rate (D) (0.0 %)"=w838) -> ("VISA resource name out"=w844:refnum<visa-resource-name>, "error out"=w843:errorcluster)  [unwired: 8 in]
                              n629 = call "Configure PID.vi"("VISA resource name"=w844, "Output's Control Loop (1:1)"=w837, "Gain (P) (50.0)"=w840, "Reset (I) (20.0)"=w839, "error in (no error)"=w843, "Rate (D) (0.0 %)"=w838) -> ("VISA resource name out"=w842:refnum<visa-resource-name>, "error out"=w841:errorcluster)  [unwired: 8 in]
                              n630 = Get Date/Time In Seconds() -> (seconds since 1Jan1904=w822:timestamp)
                              n631 = Get Date/Time String(seconds (now)=w822, want seconds? (F)=TRUE) -> (time string=w824:string)  [unwired: 1 in, 1 out]
                              n632 = local read "Text Editor Location"() -> (w827:path)
                              n633 = local read "User's Name"() -> (w829:u16)
                              n634 = local read "Status Table"() -> (w819:string[][])
                              n635 = Quotient & Remainder(x=w831, y=3) -> (x-y*floor(x/y)=w834:i32)  [unwired: 1 out]
                              n636 = local read "Edit Users"() -> (w825:bool)
                              n637 = local read "Name/Email List Location"() -> (w828:path)
                              n638 = case shown="True" w825 {
                                frame False {
                                }
                                frame True {
                                n639 = local write "Edit Users"(FALSE) -> ()
                                }
                              }
                              n640 = case shown="2" w834 {
                                tunnel: ["." ".." "..."] -> w833
                                frame 0, Default {
                                }
                                frame 1 {
                                }
                                frame 2 {
                                }
                              }
                              n641 = Array Size(array=w819) -> (size(s)=w820:i32[])
                              n642 = call "Email_List_subvi.vi"("Open File"=w825, "Name Ring In"=w829, "List Location"=w828, "Text Editor Location"=w827) -> ("String"=w830:string, "Names Out"=w826:string[])  [unwired: 5 in, 1 out]
                              n643 = Concatenate Strings("Reaching Setpoint Tolerance", w833) -> (w815:string)
                              n644 = Build Array(w824, w815) -> (w818:string[])
                              n645 = Index Array(array=w820, index=0) -> (element=w817:i32)
                              n646 = local write "User's Email"(w830) -> ()
                              n647 = property on="User's Name" class="Ring (strict)"("Strings []"=w826) -> ()  [unwired: 2 in, 2 out]
                              n648 = Decrement(x=w817) -> (x-1=w816:i32)
                              n649 = Replace Array Subset(array=w819, new element=w818, index (row)=w816) -> (w814:string[][])  [unwired: 1 in]
                              n650 = case shown="True" w885 {
                                tunnel: w875 -> [_ w960]
                                tunnel: w862 -> [_ w959]
                                tunnel: w884 -> [_ w951]
                                tunnel: w883 -> [_ w948]
                                tunnel: w814 -> [_ w945]
                                frame False {
                                }
                                frame True {
                                n651 = local read "Temperature Measurements"() -> (w961:path)
                                n652 = Number To Decimal String(number=w959) -> (decimal integer string=w955:string)  [unwired: 1 in]
                                n653 = Number To Fractional String(number=w960) -> (F-format string=w954:string)  [unwired: 3 in]
                                n654 = Get Date/Time In Seconds() -> (seconds since 1Jan1904=w956:timestamp)
                                n655 = Number To Fractional String(number=w951) -> (F-format string=w950:string)  [unwired: 3 in]
                                n656 = Number To Fractional String(number=w948) -> (F-format string=w949:string)  [unwired: 3 in]
                                n657 = Get Date/Time String(seconds (now)=w956, want seconds? (F)=TRUE) -> (date string=w952:string, time string=w953:string)  [unwired: 1 in]
                                n658 = Build Array(w955, w954, w950, w949, w953, w952) -> (w958:string[])
                                n659 = local read "Status"() -> (w946:path)
                                n660 = call-poly <vilib>:"Write To Spreadsheet File.vi"("append to file? (new file:F)"=TRUE, "1D data"=w958, "file path (dialog if empty)"=w961) -> ()  [unwired: 5 in, 1 out]
                                n661 = call-poly <vilib>:"Write To Spreadsheet File.vi"("2D data"=w945, "file path (dialog if empty)"=w946) -> ()  [unwired: 6 in, 1 out]
                                }
                              }
                              n662 = local write "Status Table"(w814) -> ()
                              n663 = node-c288() -> ()  [unwired: 1 in, 1 out]
                            }
                            n664 = node-c288(w806) -> ()  [unwired: 1 out]
                          }
                          frame True {
                          }
                        }
                      }
                      frame #5 {
                        # "Autotune crap"
                        n665 = Get Date/Time In Seconds() -> (seconds since 1Jan1904=w976:timestamp)
                        n666 = Get Date/Time String(seconds (now)=w976, want seconds? (F)=TRUE) -> (time string=w978:string)  [unwired: 1 in, 1 out]
                        n667 = local read "Status Table"() -> (w973:string[][])
                        n668 = Concatenate Strings("Setpoint Tolerance Reached") -> (w971:string)
                        n669 = Build Array(w978, w971) -> (w972:string[])
                        n670 = Array Size(array=w973) -> (size(s)=w974:i32[])
                        n671 = Insert Into Array(array=w973, new element=w972) -> (w970:string[][])  [unwired: 2 in]
                        n672 = call <vilib>:"Space Constant.vi"() -> ("String"=w979:string)
                        n673 = Index Array(array=w974, index=0) -> ()  [unwired: 1 out]
                        n674 = Build Array(w979) -> (w980:string[])
                        n675 = Build Array (concatenate)(w970, w980) -> (w968:string[][])
                        n676 = local write "Status Table"(w968) -> ()
                        n677 = local read "Status"() -> (w969:path)
                        n678 = call-poly <vilib>:"Write To Spreadsheet File.vi"("2D data"=w968, "file path (dialog if empty)"=w969) -> ()  [unwired: 6 in, 1 out]
                        n679 = disable-structure shown="Enabled" {
                          disable-tunnel: [w996 _] -> w990
                          disable-tunnel: [w995 w1044] -> w989
                          disable-tunnel: [w994 w1043] -> w988
                          disable-tunnel: w987 -> [w993 w1044]
                          disable-tunnel: w986 -> [w992 w1043]
                          frame Disabled {
                            n680 = local read "Abort?"() -> (w991:bool)
                            n681 = case shown="False" w991 {
                              tunnel: [w1001 _] -> w996
                              tunnel: [w1000 w1042] -> w995
                              tunnel: [w999 w1041] -> w994
                              tunnel: w993 -> [w998 w1042]
                              tunnel: w992 -> [w997 w1041]
                              frame False {
                                n682 = while {
                                tunnel: [w1016] -> w1001
                                tunnel: [w1011] -> w1000
                                tunnel: [w1010] -> w999
                                tunnel: w998 -> [w1007]
                                tunnel: w997 -> [w1006]
                                stop <- w1002 continue-if-true
                                w1015 = TRUE
                                n683 = call "Lakeshore_monitor.vi"("error? 2"=w1006, "VISA Resource (TPX)"=w1007) -> ("error?"=w1010:errorcluster, "Outputs"=w1038:T12, "Inputs"=w1037:T13, "VISA resource name"=w1011:refnum<visa-resource-name>)  [unwired: 5 in]
                                n684 = Unbundle(w1038) -> ("P"=w1021:dbl, "I"=w1022:dbl, "D"=w1023:dbl, "SetPoint Out2"=w1024:dbl, "1"=w1025:bool, "2"=w1026:bool, "output control loop"=w1027:dbl, "AutoTune Error"=w1016:bool, "AutoTune Active"=w1017:bool, "AutoTune Stage"=w1028:dbl, "Out1 Active"=w1029:bool, "Out1 Ramp On"=w1030:bool, "Out2 Active"=w1031:bool, "Out2 Ramp On"=w1032:bool, "Heater 2 Output 1"=w1033:dbl, "Heater 1 Output 2"=w1036:dbl, "Out1 Ramp"=w1034:dbl, "Out2 Ramp"=w1035:dbl)  [unwired: 1 out]
                                n685 = Unbundle(w1037) -> ("A:  Sample Stage"=w1018:dbl, "B:  Rad Shield"=w1019:dbl, "B: Probe Arm"=w1020:dbl, "Temp Max Alarm"=w1009:bool, "Temp Min Alarm"=w1008:bool)
                                n686 = local write "A:  Sample Stage"(w1018) -> ()
                                n687 = local write "1"(w1025) -> ()
                                n688 = local write "AutoTune Error"(w1016) -> ()
                                n689 = local write "B:  Rad Shield"(w1019) -> ()
                                n690 = local write "Room Temp (K)"(w1020) -> ()
                                n691 = local write "Temp Max Alarm"(w1009) -> ()
                                n692 = local write "Temp Min Alarm"(w1008) -> ()
                                n693 = local write "P"(w1021) -> ()
                                n694 = local write "Heater 1 Output2"(w1036) -> ()
                                n695 = local write "AutoTune Stage"(w1028) -> ()
                                n696 = local write "Out2 Ramp"(w1035) -> ()
                                n697 = local write "Out1 Ramp"(w1034) -> ()
                                n698 = local write "2"(w1026) -> ()
                                n699 = local write "I"(w1022) -> ()
                                n700 = local write "Heater 2 Output1"(w1033) -> ()
                                n701 = Wait (ms)(milliseconds to wait=100) -> ()  [unwired: 1 out]
                                n702 = local write "output control loop"(w1027) -> ()
                                n703 = local write "Setpoint (K)"(w1024) -> ()
                                n704 = local write "D"(w1023) -> ()
                                n705 = local write "AutoTune Active"(w1017) -> ()
                                n706 = local read "A: Low Alarm"() -> (w1013:dbl)
                                n707 = local read "A: High Alarm"() -> (w1014:dbl)
                                n708 = Or(x=w1009, y=w1008) -> (x .or. y?=w1012:bool)
                                n709 = local write "Out 2\nRamp On"(w1032) -> ()
                                n710 = local write "Out 2\nActive"(w1031) -> ()
                                n711 = local write "Out 1\nRamp On"(w1030) -> ()
                                n712 = local write "Out 1\nActive"(w1029) -> ()
                                n713 = local read "Abort?"() -> (w1004:bool)
                                n714 = call "Configure Alarm.vi"("VISA resource name"=w1011, "High Value (0.00000)"=w1014, "Low Value (0.00000)"=w1013, "Enable Alarm (F: Off)"=w1015, "Enable Latching (F: Off)"=w1015, "error in (no error)"=w1010, "Enable Beep (F: Off)"=w1015, "Enable Display (F: Off)"=w1012) -> ()  [unwired: 6 in, 2 out]
                                n715 = Not(x=w1016) -> (.not. x?=w1040:bool)
                                n716 = Not(x=w1004) -> (.not. x?=w1005:bool)
                                n717 = And(x=w1017, y=w1040) -> (x .and. y?=w1003:bool)
                                n718 = And(x=w1003, y=w1005) -> (x .and. y?=w1002:bool)
                                }
                              }
                              frame True {
                              }
                            }
                          }
                          frame Enabled {
                          }
                        }
                      }
                      frame #6 {
                        n719 = local read "Abort?"() -> (w1051:bool)
                        n720 = case shown="False" w1051 {
                          tunnel: w1053 -> [w1061 _]
                          tunnel: w1052 -> [w1060 _]
                          tunnel: w1050 -> [w1059 _]
                          tunnel: w1049 -> [w1058 _]
                          tunnel: w1048 -> [w1057 _]
                          tunnel: [w1056 _] -> w1047
                          tunnel: [w1055 _] -> w1046
                          tunnel: w1045 -> [w1054 _]
                          frame False {
                            n721 = stacked-sequence {
                              seq-local: [w1069 _ _ _] -> [_ w1336 _ _]
                              seq-local: [w1068 _ _ _] -> [_ w1335 _ _]
                              seq-local: [w1064 _ _ _] -> [_ w1310 _ _]
                              seq-local: [w1063 _ _ _] -> [_ w1331 _ _]
                              seq-local: [_ w1334 _ _] -> [_ _ w1369 _]
                              seq-local: [_ w1333 _ _] -> [_ _ w1368 _]
                              seq-local: [_ w1329 _ _] -> [_ _ w1366 _]
                              seq-local: [_ w1328 _ _] -> [_ _ w1365 _]
                              seq-local: [_ _ w1367 _] -> [_ _ _ w1700]
                              seq-local: [_ _ w1364 _] -> [_ _ _ w1702]
                              seq-local: [_ _ w1363 _] -> [_ _ _ w1701]
                              seq-local: [_ _ w1362 _] -> [_ _ _ w1699]
                              tunnel: w1061 -> [w1071 _ _ _]
                              tunnel: w1060 -> [w1070 _ _ _]
                              tunnel: w1059 -> [w1067 _ _ _]
                              tunnel: w1058 -> [w1066 _ _ _]
                              tunnel: w1057 -> [w1065 _ _ _]
                              tunnel: w1054 -> [w1062 _ _ _]
                              tunnel: [_ _ _ w1698] -> w1056
                              tunnel: [_ _ _ w1697] -> w1055
                              frame #0 {
                                n722 = while {
                                tunnel: w1071 -> [w1096]
                                tunnel: w1070 -> [w1095]
                                tunnel: [w1092] -> w1069
                                tunnel: [w1091] -> w1068
                                tunnel: w1067 -> [w1090]
                                shift-right: [w1087] -> w1064
                                shift-left: w1066 -> [w1089]
                                shift-right: [w1086] -> w1063
                                shift-left: w1065 -> [w1088]
                                tunnel: w1062 -> [w1072]
                                stop <- w1073 stop-if-true
                                n723 = node-c288() -> (w1098:T9)  [unwired: 4 in]
                                n724 = timed-loop {
                                timing: w1098 -> [_]
                                timing-out: [_] -> w1097
                                tunnel: w1096 -> [w1219]
                                tunnel: w1095 -> [w1218]
                                shift-right: [w1242] -> w1093
                                shift-left: i32[] [] -> [w1241]
                                tunnel: [w1104] -> w1092
                                tunnel: [w1150] -> w1091
                                tunnel: w1090 -> [w1180]
                                shift-right: [w1191] -> w1087
                                shift-left: w1089 -> [w1194]
                                shift-right: [w1192] -> w1086
                                shift-left: w1088 -> [w1193]
                                tunnel: [w1172] -> w1074
                                tunnel: w1072 -> [w1149]
                                i -> [w1141]
                                stop <- w1110 stop-if-true
                                w1159 = TRUE
                                w1220 = TRUE
                                # "10 minute wait until measurement taken regardless of actual temperature"
                                n725 = node-c288() -> ()  [unwired: 1 in, 1 out]
                                n726 = local read "Sample Properties:"() -> (w1209:T4)
                                n727 = local read "Target"() -> (w1182:dbl)
                                n728 = local read "Stability Time (s)"() -> (w1244:dbl)
                                n729 = Unbundle(w1209) -> ("Date Created"=w1208:timestamp, "Material"=w1207:string, "Solvent"=w1206:string, "Concentration"=w1205:string, "Method"=w1204:string, "Dielectric (d)"=w1203:string, "Index (#)"=w1202:string, "Index (ABC)"=w1201:string, "Length"=w1200:string, "Width"=w1199:string, "Surface Treatment"=w1198:string, "Comments"=w1197:string)  [unwired: 1 out]
                                n730 = call "Lakeshore_monitor.vi"("error? 2"=w1218, "VISA Resource (TPX)"=w1219) -> ("error?"=w1186:errorcluster, "Outputs"=w1221:T12, "Inputs"=w1222:T13, "VISA resource name"=w1184:refnum<visa-resource-name>)  [unwired: 5 in]
                                n731 = local read "SetPoint2\nOVR"() -> (w1167:dbl)
                                n732 = Not Equal?(x=w1182, y=w1167) -> (x != y?=w1181:bool)
                                n733 = local read "Rate (K/min)"() -> (w1166:dbl)
                                n734 = local read "Time Iteration (s)"() -> (w1213:dbl)
                                n735 = Unbundle(w1221) -> ("P"=w1238:dbl, "I"=w1237:dbl, "D"=w1236:dbl, "SetPoint Out2"=w1235:dbl, "1"=w1234:bool, "2"=w1233:bool, "output control loop"=w1232:dbl, "AutoTune Error"=w1240:bool, "AutoTune Active"=w1239:bool, "AutoTune Stage"=w1231:dbl, "Out1 Active"=w1230:bool, "Out1 Ramp On"=w1229:bool, "Out2 Active"=w1228:bool, "Out2 Ramp On"=w1227:bool, "Heater 2 Output 1"=w1226:dbl, "Heater 1 Output 2"=w1223:dbl, "Out1 Ramp"=w1225:dbl, "Out2 Ramp"=w1224:dbl)  [unwired: 1 out]
                                n736 = Unbundle(w1222) -> ("A:  Sample Stage"=w1190:dbl, "B:  Rad Shield"=w1212:dbl, "B: Probe Arm"=w1211:dbl, "Temp Max Alarm"=w1217:bool, "Temp Min Alarm"=w1216:bool)
                                n737 = Bundle("Date Created"=w1208, "Material"=w1207, "Solvent"=w1206, "Concentration"=w1205, "Method"=w1204, "Dielectric (d)"=w1203, "Index (#)"=w1202, "Index (ABC)"=w1201, "Length"=w1200, "Width"=w1199, "Surface Treatment"=w1198, "Comments"=w1197, "A:  Sample Stage"=w1190) -> (w1210:T22)  [unwired: 1 in]
                                n738 = call "Elapsed Time3"("Time Target (s)"=w1213, "Auto Reset"=TRUE) -> ("Present (s)"=w1195:dbl, "Time has Elapsed"=w1189:bool)  [unwired: 10 in, 6 out]
                                n739 = local write "Sample Properties:"(w1210) -> ()
                                n740 = Build Array (concatenate)(w1241, w1190) -> (w1242:dbl[])
                                n741 = Multiply(x=w1244, y=1) -> (x*y=w1243:dbl)
                                n742 = Less Or Equal?(x=w1243, y=w1141) -> (x <= y?=w1174:bool)
                                n743 = local write "A:  Sample Stage"(w1190) -> ()
                                n744 = local write "1"(w1234) -> ()
                                n745 = local write "AutoTune Error"(w1240) -> ()
                                n746 = local write "B:  Rad Shield"(w1212) -> ()
                                n747 = local write "Temp Max Alarm"(w1217) -> ()
                                n748 = local write "Temp Min Alarm"(w1216) -> ()
                                n749 = local write "P"(w1238) -> ()
                                n750 = local write "C:  Probe Arm"(w1211) -> ()
                                n751 = local read "Start Time Num"() -> (w1196:dbl)
                                n752 = local write "Heater 1 Output2"(w1223) -> ()
                                n753 = local write "AutoTune Stage"(w1231) -> ()
                                n754 = local write "Heater 2 Output1"(w1226) -> ()
                                n755 = local write "Out2 Ramp"(w1224) -> ()
                                n756 = local read "Output 2 Range"() -> (w1215:enum16{"Off", "Low (On)", "Medium", "High"})
                                n757 = local write "Out1 Ramp"(w1225) -> ()
                                n758 = local write "2"(w1233) -> ()
                                n759 = local write "I"(w1237) -> ()
                                n760 = local read "Abort?"() -> (w1118:bool)
                                n761 = case shown="True" w1181 {
                                tunnel: w1186 -> [w1269 w1280]
                                tunnel: [w1269 w1273] -> w1185
                                tunnel: w1184 -> [w1270 w1279]
                                tunnel: [w1270 w1274] -> w1183
                                tunnel: w1167 -> [_ w1272]
                                tunnel: w1167 -> [_ w1278]
                                tunnel: w1180 -> [_ w1277]
                                tunnel: w1149 -> [_ w1271]
                                frame False {
                                }
                                frame True {
                                n762 = local write "Target"(w1278) -> ()
                                n763 = call "Configure Setpoint and Ramp.vi"("VISA resource name"=w1279, "Output's Control Loop (1:1)"=w1277, "Setpoint (0.00000)"=w1272, "error in (no error)"=w1280) -> ("VISA resource name out"=w1276:refnum<visa-resource-name>, "error out"=w1275:errorcluster)  [unwired: 10 in]
                                n764 = call "Configure Setpoint and Ramp.vi"("VISA resource name"=w1276, "Output's Control Loop (1:1)"=w1271, "Setpoint (0.00000)"=w1272, "error in (no error)"=w1275) -> ("VISA resource name out"=w1274:refnum<visa-resource-name>, "error out"=w1273:errorcluster)  [unwired: 10 in]
                                }
                                }
                                n765 = Subtract(x=w1195, y=w1196) -> (x-y=w1177:dbl)
                                n766 = local write "Elapsed Time"(w1177) -> ()
                                n767 = local write "output control loop"(w1232) -> ()
                                n768 = local write "Setpoint (K)"(w1235) -> ()
                                n769 = Greater Than 0?(x=w1190) -> (x > 0?=w1187:bool)
                                n770 = case shown="True" w1187 {
                                tunnel: w1194 -> [_ w1288]
                                tunnel: w1193 -> [_ w1287]
                                tunnel: w1177 -> [_ w1286]
                                tunnel: [_ w1283] -> w1192
                                tunnel: [_ w1282] -> w1191
                                tunnel: w1190 -> [_ w1281]
                                frame False {
                                }
                                frame True {
                                n771 = Build Array (concatenate)(w1287, w1286) -> (w1283:dbl[])
                                n772 = Build Array (concatenate)(w1288, w1281) -> (w1282:dbl[])
                                n773 = Bundle(w1283, w1282) -> (w1284:cluster{dbl[], dbl[]})  [unwired: 1 in]
                                n774 = Build Array(w1284) -> (w1285:cluster{dbl[], dbl[]}[])
                                n775 = local write "Temp Graph"(w1285) -> ()
                                }
                                }
                                n776 = local write "D"(w1236) -> ()
                                n777 = local write "AutoTune Active"(w1239) -> ()
                                n778 = And(x=w1187, y=w1189) -> (x .and. y?=w1188:bool)
                                n779 = local read "A: Low Alarm"() -> (w1157:dbl)
                                n780 = local read "A: High Alarm"() -> (w1158:dbl)
                                n781 = local read "Output 1 Range"() -> (w1160:enum16{"Off", "Low (On)", "Medium", "High"})
                                n782 = local read "Settle Time (s)"() -> (w1178:dbl)
                                n783 = Compound Arithmetic op=OR(w1217, w1216, w1118) -> (w1123:bool)
                                n784 = local write "Out 2\nActive"(w1228) -> ()
                                n785 = local write "Out 1\nActive"(w1230) -> ()
                                n786 = Greater Than 0?(x=w1166) -> (x > 0?=w1165:bool)
                                n787 = call "Configure Setpoint and Ramp.vi"("VISA resource name"=w1183, "Output's Control Loop (1:1)"=w1180, "Setpoint (0.00000)"=w1167, "Setpoint Ramping \nEnable (F: Off)"=w1165, "error in (no error)"=w1185, "Ramp Rate (0.0)"=w1166) -> ("VISA resource name out"=w1171:refnum<visa-resource-name>, "error out"=w1170:errorcluster)  [unwired: 8 in]
                                n788 = local write "Abort?"(w1123) -> ()
                                n789 = local read "Out 2\nRamp On"() -> (w1121:bool)
                                n790 = local read "Out 1\nRamp On"() -> (w1122:bool)
                                n791 = local write "Out 2\nRamp On"(w1227) -> ()
                                n792 = local write "Out 1\nRamp On"(w1229) -> ()
                                n793 = call "Configure Setpoint and Ramp.vi"("VISA resource name"=w1171, "Output's Control Loop (1:1)"=w1149, "Setpoint (0.00000)"=w1167, "Setpoint Ramping \nEnable (F: Off)"=w1165, "error in (no error)"=w1170, "Ramp Rate (0.0)"=w1166) -> ("VISA resource name out"=w1169:refnum<visa-resource-name>, "error out"=w1168:errorcluster)  [unwired: 8 in]
                                n794 = call "Configure Output Range and Manual Value.vi"("VISA resource name"=w1169, "Output (1:1)"=w1180, "Range (0:Off)"=w1215, "error in (no error)"=w1168) -> ("VISA resource name out"=w1164:refnum<visa-resource-name>, "error out"=w1163:errorcluster)  [unwired: 10 in]
                                n795 = call "Configure Output Range and Manual Value.vi"("VISA resource name"=w1164, "Output (1:1)"=w1149, "Range (0:Off)"=w1160, "error in (no error)"=w1163) -> ("VISA resource name out"=w1162:refnum<visa-resource-name>, "error out"=w1161:errorcluster)  [unwired: 10 in]
                                n796 = call "Configure Alarm.vi"("VISA resource name"=w1162, "High Value (0.00000)"=w1158, "Low Value (0.00000)"=w1157, "Enable Alarm (F: Off)"=w1220, "Enable Latching (F: Off)"=w1220, "error in (no error)"=w1161, "Enable Beep (F: Off)"=w1220, "Enable Display (F: Off)"=w1123) -> ("VISA resource name out"=w1156:refnum<visa-resource-name>, "error out"=w1155:errorcluster)  [unwired: 6 in]
                                n797 = Subtract(x=w1177, y=w1178) -> (x-y=w1175:dbl)
                                n798 = Greater Or Equal?(x=w1175, y=600) -> (x >= y?=w1172:bool)
                                n799 = Build Array(w1174, w1118, w1172) -> (w1173:bool[])
                                n800 = Or Array Elements(Boolean array=w1173) -> (logical OR=w1111:bool)
                                n801 = case shown="True" w1122 {
                                frame False {
                                n802 = property on="1" class="Bool (strict)"("BoolText.Text"="") -> ()  [unwired: 2 in, 2 out]
                                }
                                frame True {
                                n803 = local read "Out 1\nActive"() -> (w1262:bool)
                                n804 = case shown="False" w1262 {
                                frame False {
                                n805 = property on="1" class="Bool (strict)"("BoolText.Text"="Ramp\nOn") -> ()  [unwired: 2 in, 2 out]
                                }
                                frame True {
                                n806 = property on="1" class="Bool (strict)"("BoolText.Text"="Ramp\nActive") -> ()  [unwired: 2 in, 2 out]
                                }
                                }
                                }
                                }
                                n807 = case shown="False" w1121 {
                                frame False {
                                n808 = property on="2" class="Bool (strict)"("BoolText.Text"="") -> ()  [unwired: 2 in, 2 out]
                                }
                                frame True {
                                n809 = local read "Out 2\nActive"() -> (w1258:bool)
                                n810 = case shown="True" w1258 {
                                frame False {
                                n811 = property on="2" class="Bool (strict)"("BoolText.Text"="Ramp\nOn") -> ()  [unwired: 2 in, 2 out]
                                }
                                frame True {
                                n812 = property on="2" class="Bool (strict)"("BoolText.Text"="Ramp\nActive") -> ()  [unwired: 2 in, 2 out]
                                }
                                }
                                }
                                }
                                n813 = local read "P 2"() -> (w1148:dbl)
                                n814 = local read "D 2"() -> (w1146:dbl)
                                n815 = local read "I 2"() -> (w1147:dbl)
                                n816 = local read "Target"() -> (w1120:dbl)
                                n817 = local read "Text Editor Location"() -> (w1137:path)
                                n818 = local read "User's Name"() -> (w1139:u16)
                                n819 = call "Configure Alarm.vi"("VISA resource name"=w1156, "High Value (0.00000)"=w1158, "Low Value (0.00000)"=w1157, "Input (0:A)"=w1149, "Enable Alarm (F: Off)"=w1159, "Enable Latching (F: Off)"=w1159, "error in (no error)"=w1155, "Enable Beep (F: Off)"=w1159, "Enable Display (F: Off)"=w1123) -> ("VISA resource name out"=w1154:refnum<visa-resource-name>, "error out"=w1153:errorcluster)  [unwired: 5 in]
                                n820 = call "Configure PID.vi"("VISA resource name"=w1154, "Output's Control Loop (1:1)"=2, "Gain (P) (50.0)"=w1148, "Reset (I) (20.0)"=w1147, "error in (no error)"=w1153, "Rate (D) (0.0 %)"=w1146) -> ("VISA resource name out"=w1152:refnum<visa-resource-name>, "error out"=w1151:errorcluster)  [unwired: 8 in]
                                n821 = call "Configure PID.vi"("VISA resource name"=w1152, "Output's Control Loop (1:1)"=w1149, "Gain (P) (50.0)"=w1148, "Reset (I) (20.0)"=w1147, "error in (no error)"=w1151, "Rate (D) (0.0 %)"=w1146) -> ("VISA resource name out"=w1104:refnum<visa-resource-name>, "error out"=w1150:errorcluster)  [unwired: 8 in]
                                n822 = Quotient & Remainder(x=w1141, y=3) -> (x-y*floor(x/y)=w1144:i32)  [unwired: 1 out]
                                n823 = local read "Edit Users"() -> (w1135:bool)
                                n824 = Get Date/Time In Seconds() -> (seconds since 1Jan1904=w1132:timestamp)
                                n825 = local read "Delay Start"() -> (w1109:dbl)
                                n826 = local read "VISA resource name"() -> (w1103:refnum<visa-resource-name>)
                                n827 = event shown="[1] \"Light is...\": Mouse Down" {
                                selector: _ -> [_ _]
                                dyn-events: _ -> [_ _]
                                timeout: 10 -> [_ _]
                                tunnel: w1103 -> [_ w1249]
                                event Timeout {
                                n828 = event-data() -> ()  [unwired: 1 in, 2 out]
                                }
                                event "Light is...": Mouse Down {
                                n829 = event-data() -> ()  [unwired: 1 in, 2 out]
                                n830 = local read "Light Bathe Cluster"() -> (w1248:T2)
                                n831 = Bundle By Name(cluster=w1248, "Post Measure:"=FALSE) -> (w1247:T2)
                                n832 = local write "Light Bathe Cluster"(w1247) -> ()
                                n833 = local read "Light is..."() -> (w1250:bool)
                                n834 = case shown="True" w1250 {
                                tunnel: w1249 -> [w1251 w1253]
                                frame False {
                                w1252 = u32 1 items=["positive pulse  ", "negative pulse  ", "level high  ", "level low  "] ("trigger signal")
                                n835 = call "HP415xA Op-Trigger Output.vi"("trigger signal"=w1252, "VISA session"=w1251) -> ()  [unwired: 2 in, 1 out]
                                }
                                frame True {
                                w1254 = u32 0 items=["positive pulse  ", "negative pulse  ", "level high  ", "level low  "] ("trigger signal")
                                n836 = call "HP415xA Op-Trigger Output.vi"("trigger signal"=w1254, "VISA session"=w1253) -> ()  [unwired: 2 in, 1 out]
                                }
                                }
                                }
                                }
                                n837 = local read "Light On Duration\n (min)"() -> (w1115:dbl)
                                n838 = local read "Time Iteration (s)"() -> (w1101:dbl)
                                n839 = call "Elapsed Time10"("Time Target (s)"=w1101) -> ("Present (s)"=w1117:dbl)  [unwired: 11 in, 7 out]
                                n840 = Subtract(x=w1117, y=w1109) -> (x-y=w1113:dbl)
                                n841 = Multiply(x=w1115, y=60) -> (x*y=w1112:dbl)
                                n842 = Subtract(x=w1112, y=w1113) -> (x-y=w1116:dbl)
                                n843 = local write "Light \nCount Down"(w1116) -> ()
                                n844 = Less Or Equal To 0?(x=w1116) -> (x <= 0?=w1106:bool)
                                n845 = local read "Name/Email List Location"() -> (w1138:path)
                                n846 = local read "Light Bathe Cluster"() -> (w1100:T2)
                                n847 = Get Date/Time String(seconds (now)=w1132, want seconds? (F)=TRUE) -> (time string=w1134:string)  [unwired: 1 in, 1 out]
                                n848 = case shown="True" w1135 {
                                frame False {
                                }
                                frame True {
                                n849 = local write "Edit Users"(FALSE) -> ()
                                }
                                }
                                n850 = case shown="2" w1144 {
                                tunnel: ["." ".." "..."] -> w1143
                                frame 0, Default {
                                }
                                frame 1 {
                                }
                                frame 2 {
                                }
                                }
                                n851 = Unbundle By Name(w1100) -> ("Post Measure:"=w1099:bool)
                                n852 = And(x=w1099, y=w1106) -> (x .and. y?=w1105:bool)
                                n853 = case shown="True" w1105 {
                                tunnel: w1103 -> [_ w1256]
                                frame False {
                                }
                                frame True {
                                w1255 = u32 0 items=["positive pulse  ", "negative pulse  ", "level high  ", "level low  "] ("trigger signal")
                                n854 = call "HP415xA Op-Trigger Output.vi"("trigger signal"=w1255, "VISA session"=w1256) -> ()  [unwired: 2 in, 1 out]
                                }
                                }
                                n855 = Select(t=w1106, s=w1099, f=TRUE) -> (s? t:f=w1108:bool)
                                n856 = And(x=w1108, y=w1111) -> (x .and. y?=w1110:bool)
                                n857 = local read "Status Table"() -> (w1129:string[][])
                                n858 = Number To Fractional String(number=w1120) -> (F-format string=w1119:string)  [unwired: 3 in]
                                n859 = call "Email_List_subvi.vi"("Open File"=w1135, "Name Ring In"=w1139, "List Location"=w1138, "Text Editor Location"=w1137) -> ("String"=w1140:string, "Names Out"=w1136:string[])  [unwired: 5 in, 1 out]
                                n860 = Concatenate Strings("Waiting for Temperature to Settle to ", w1119, w1143) -> (w1127:string)
                                n861 = Build Array(w1134, w1127) -> (w1128:string[])
                                n862 = Array Size(array=w1129) -> (size(s)=w1130:i32[])
                                n863 = local write "User's Email"(w1140) -> ()
                                n864 = property on="User's Name" class="Ring (strict)"("Strings []"=w1136) -> ()  [unwired: 2 in, 2 out]
                                n865 = Index Array(array=w1130, index=0) -> (element=w1126:i32)
                                n866 = node-c288() -> ()  [unwired: 1 in, 1 out]
                                n867 = Decrement(x=w1126) -> (x-1=w1125:i32)
                                n868 = Replace Array Subset(array=w1129, new element=w1128, index (row)=w1125) -> (w1124:string[][])  [unwired: 1 in]
                                n869 = case shown="True" w1188 {
                                tunnel: w1190 -> [_ w1304]
                                tunnel: w1177 -> [_ w1303]
                                tunnel: w1212 -> [_ w1295]
                                tunnel: w1211 -> [_ w1292]
                                tunnel: w1124 -> [_ w1289]
                                frame False {
                                }
                                frame True {
                                n870 = local read "Temperature Measurements"() -> (w1305:path)
                                n871 = Number To Decimal String(number=w1303) -> (decimal integer string=w1299:string)  [unwired: 1 in]
                                n872 = Number To Fractional String(number=w1304) -> (F-format string=w1298:string)  [unwired: 3 in]
                                n873 = Get Date/Time In Seconds() -> (seconds since 1Jan1904=w1300:timestamp)
                                n874 = Number To Fractional String(number=w1295) -> (F-format string=w1294:string)  [unwired: 3 in]
                                n875 = Number To Fractional String(number=w1292) -> (F-format string=w1293:string)  [unwired: 3 in]
                                n876 = Get Date/Time String(seconds (now)=w1300, want seconds? (F)=TRUE) -> (date string=w1296:string, time string=w1297:string)  [unwired: 1 in]
                                n877 = Build Array(w1299, w1298, w1294, w1293, w1297, w1296) -> (w1302:string[])
                                n878 = local read "Status"() -> (w1290:path)
                                n879 = call-poly <vilib>:"Write To Spreadsheet File.vi"("append to file? (new file:F)"=TRUE, "1D data"=w1302, "file path (dialog if empty)"=w1305) -> ()  [unwired: 5 in, 1 out]
                                n880 = call-poly <vilib>:"Write To Spreadsheet File.vi"("2D data"=w1289, "file path (dialog if empty)"=w1290) -> ()  [unwired: 6 in, 1 out]
                                }
                                }
                                n881 = local write "Status Table"(w1124) -> ()
                                }
                                n882 = node-c288(w1097) -> ()  [unwired: 1 out]
                                n883 = local read "Setpoint Tolerance (K)"() -> (w1084:dbl)
                                n884 = local read "Target"() -> (w1083:dbl)
                                n885 = Array Max & Min(array=w1093) -> (max value=w1082:dbl, min value=w1081:dbl)  [unwired: 2 out]
                                n886 = local read "Abort?"() -> (w1075:bool)
                                n887 = Subtract(x=w1083, y=w1084) -> (x-y=w1079:dbl)
                                n888 = Add(x=w1083, y=w1084) -> (x+y=w1080:dbl)
                                n889 = In Range and Coerce(upper limit=w1080, x=w1082, lower limit=w1079) -> (In Range?=w1085:bool)  [unwired: 1 out]
                                n890 = In Range and Coerce(upper limit=w1080, x=w1081, lower limit=w1079) -> (In Range?=w1078:bool)  [unwired: 1 out]
                                n891 = And(x=w1085, y=w1078) -> (x .and. y?=w1076:bool)
                                n892 = Build Array(w1076, w1075, w1074) -> (w1077:bool[])
                                n893 = Or Array Elements(Boolean array=w1077) -> (logical OR=w1073:bool)
                                }
                              }
                              frame #1 {
                                n894 = Get Date/Time In Seconds() -> (seconds since 1Jan1904=w1321:timestamp)
                                n895 = local read "Time Iteration (s)"() -> (w1347:dbl)
                                n896 = local read "Start Time Num"() -> (w1346:dbl)
                                n897 = call "Elapsed Time7"("Time Target (s)"=w1347, "Auto Reset"=TRUE) -> ("Present (s)"=w1345:dbl)  [unwired: 10 in, 7 out]
                                n898 = Get Date/Time String(seconds (now)=w1321, want seconds? (F)=TRUE) -> (time string=w1323:string)  [unwired: 1 in, 1 out]
                                n899 = local read "Status Table"() -> (w1318:string[][])
                                n900 = Subtract(x=w1345, y=w1346) -> (x-y=w1330:dbl)
                                n901 = local read "Temperature Measurements"() -> (w1341:path)
                                n902 = Build Array (concatenate)(w1331, w1330) -> (w1328:dbl[])
                                n903 = call "Lakeshore_monitor.vi"("error? 2"=w1335, "VISA Resource (TPX)"=w1336) -> ("error?"=w1333:errorcluster, "Inputs"=w1339:T13, "VISA resource name"=w1334:refnum<visa-resource-name>)  [unwired: 5 in, 1 out]
                                n904 = Array Size(array=w1318) -> (size(s)=w1319:i32[])
                                n905 = Unbundle(w1339) -> ("A:  Sample Stage"=w1311:dbl, "B:  Rad Shield"=w1338:dbl, "B: Probe Arm"=w1337:dbl)  [unwired: 2 out]
                                n906 = Build Array (concatenate)(w1310, w1311) -> (w1329:dbl[])
                                n907 = Number To Fractional String(number=w1311) -> (F-format string=w1312:string)  [unwired: 3 in]
                                n908 = Bundle(w1328, w1329) -> (w1332:cluster{dbl[], dbl[]})  [unwired: 1 in]
                                n909 = Concatenate Strings("Temperature Reached ", w1312) -> (w1316:string)
                                n910 = Build Array(w1323, w1316) -> (w1317:string[])
                                n911 = Insert Into Array(array=w1318, new element=w1317) -> (w1315:string[][])  [unwired: 2 in]
                                n912 = call <vilib>:"Space Constant.vi"() -> ("String"=w1324:string)
                                n913 = local write "A:  Sample Stage"(w1311) -> ()
                                n914 = Build Array(w1332) -> (w1327:cluster{dbl[], dbl[]}[])
                                n915 = local write "B:  Rad Shield"(w1338) -> ()
                                n916 = Build Array("Measurement Start...") -> (w1343:string[])
                                n917 = local write "C:  Probe Arm"(w1337) -> ()
                                n918 = Index Array(array=w1319, index=0) -> ()  [unwired: 1 out]
                                n919 = Build Array(w1324) -> (w1325:string[])
                                n920 = local write "Temp Graph"(w1327) -> ()
                                n921 = Build Array (concatenate)(w1315, w1325) -> (w1313:string[][])
                                n922 = local write "Status Table"(w1313) -> ()
                                n923 = local read "Status"() -> (w1314:path)
                                n924 = Number To Fractional String(number=w1311) -> (F-format string=w1350:string)  [unwired: 3 in]
                                n925 = Number To Decimal String(number=w1330) -> (decimal integer string=w1355:string)  [unwired: 1 in]
                                n926 = Get Date/Time In Seconds() -> (seconds since 1Jan1904=w1349:timestamp)
                                n927 = Number To Fractional String(number=w1338) -> (F-format string=w1353:string)  [unwired: 3 in]
                                n928 = Number To Fractional String(number=w1337) -> (F-format string=w1354:string)  [unwired: 3 in]
                                n929 = call-poly <vilib>:"Write To Spreadsheet File.vi"("2D data"=w1313, "file path (dialog if empty)"=w1314) -> ()  [unwired: 6 in, 1 out]
                                n930 = Get Date/Time String(seconds (now)=w1349, want seconds? (F)=TRUE) -> (date string=w1352:string, time string=w1351:string)  [unwired: 1 in]
                                n931 = Build Array(w1355, w1350, w1353, w1354, w1351, w1352) -> (w1357:string[])
                                n932 = Build Array(w1343, w1357) -> (w1344:string[][])
                                n933 = call-poly <vilib>:"Write To Spreadsheet File.vi"("append to file? (new file:F)"=TRUE, "2D data"=w1344, "file path (dialog if empty)"=w1341) -> ()  [unwired: 5 in, 1 out]
                              }
                              frame #2 {
                                # "Figure out what these are"
                                n934 = local read "Abort?"() -> (w1370:bool)
                                n935 = local read "Transport"() -> (w1360:bool)
                                n936 = local read "Transfer 2"() -> (w1361:bool)
                                n937 = Or(x=w1360, y=w1361) -> (x .or. y?=w1359:bool)
                                n938 = Not(x=w1359) -> (.not. x?=w1371:bool)
                                n939 = Or(x=w1371, y=w1370) -> (x .or. y?=w1358:bool)
                                n940 = case shown="False" w1358 {
                                tunnel: w1368 -> [w1379 _]
                                tunnel: w1370 -> [_ w1665]
                                tunnel: w1369 -> [w1375 w1664]
                                tunnel: w1368 -> [w1374 w1663]
                                tunnel: [w1378 _] -> w1367
                                tunnel: w1366 -> [w1377 _]
                                tunnel: w1365 -> [w1376 _]
                                tunnel: [w1375 w1664] -> w1364
                                tunnel: [w1374 w1663] -> w1363
                                tunnel: [w1373 _] -> w1362
                                frame False {
                                n941 = local read "# of Loops"() -> (w1372:dbl)
                                n942 = for {
                                N: w1372 -> [_]
                                tunnel: w1379 -> [w1388]
                                tunnel: [w1387] -> w1378 mode=concatenating
                                tunnel: w1377 -> [w1386]
                                tunnel: w1376 -> [w1385]
                                tunnel: w1375 -> [w1384]
                                tunnel: w1374 -> [w1383]
                                tunnel: [w1382] -> w1373 mode=concatenating
                                tunnel: w1372 -> [w1381]
                                i -> [w1380]
                                n943 = stacked-sequence {
                                tunnel: w1388 -> [_ w1399 _]
                                tunnel: [_ w1446 _] -> w1387
                                tunnel: w1386 -> [_ w1445 _]
                                tunnel: w1385 -> [_ w1444 _]
                                tunnel: w1384 -> [_ w1443 _]
                                tunnel: w1383 -> [_ w1442 _]
                                tunnel: [_ w1441 _] -> w1382
                                tunnel: w1381 -> [_ _ w1638]
                                tunnel: w1380 -> [_ _ w1637]
                                tunnel: w1380 -> [_ w1390 _]
                                frame #0 {
                                n944 = flat-sequence {
                                frame #0 {
                                n945 = disable-structure shown="Disabled" {
                                frame Disabled {
                                n946 = while {
                                stop <- _ stop-if-true
                                }
                                }
                                frame Enabled {
                                }
                                }
                                }
                                frame #1 {
                                n947 = local write "Status LED"(TRUE) -> ()
                                }
                                }
                                }
                                frame #1 {
                                # "Super Duper subvi"
                                n948 = local read "Start 2"() -> (w1474:dbl)
                                n949 = local read "Stop 2"() -> (w1473:dbl)
                                n950 = local read "Step 2"() -> (w1472:dbl)
                                n951 = local read "Var1 sweep settings 2"() -> (w1457:T7)
                                n952 = local read "Start"() -> (w1476:dbl)
                                n953 = local read "Step"() -> (w1479:dbl)
                                n954 = local read "Var1 sweep settings"() -> (w1430:T7)
                                n955 = local read "Stop 3"() -> (w1463:dbl)
                                n956 = local read "Var2 step settings 2"() -> (w1455:T8)
                                n957 = local read "Start"() -> (w1464:dbl)
                                n958 = local read "Start"() -> (w1461:dbl)
                                n959 = local read "Step"() -> (w1462:dbl)
                                n960 = local read "Step"() -> (w1460:dbl)
                                n961 = local read "Var2 step settings"() -> (w1456:T8)
                                n962 = local read "Integration Time 3"() -> (w1470:u32)
                                n963 = local read "VISA resource name"() -> (w1448:refnum<visa-resource-name>)
                                n964 = local read "Integration Time"() -> (w1458:u32)
                                n965 = local read "Total Points"() -> (w1475:u16)
                                n966 = local read "# of Loops"() -> (w1478:dbl)
                                n967 = local read "Loop Wait"() -> (w1469:dbl)
                                n968 = local read "Wait Countdown"() -> (w1452:dbl)
                                n969 = local read "Transfer 2"() -> (w1477:bool)
                                n970 = local read "Loop Step"() -> (w1471:dbl)
                                n971 = local read "First Step"() -> (w1468:dbl)
                                n972 = local read "Total Points"() -> (w1459:u16)
                                n973 = local read "Transport"() -> (w1465:bool)
                                n974 = local read "Wait Time (s)"() -> (w1451:dbl)
                                n975 = local read "Sample Properties:"() -> (w1480:T4)
                                n976 = local read "Electrical Measurements"() -> (w1481:path)
                                n977 = Bundle("Step"=w1479, "# of Loops"=w1478, "Transfer 2"=w1477, "Start"=w1476, "Total Points"=w1475, "Start 2"=w1474, "Stop 2"=w1473, "Step 2"=w1472, "Loop Step"=w1471, "Integration Time 3"=w1470, "Loop Wait"=w1469, "First Step"=w1468) -> (w1467:T15)  [unwired: 1 in]
                                n978 = Bundle("Transport"=w1465, "Start"=w1464, "Stop 3"=w1463, "Step"=w1462, "Start"=w1461, "Step"=w1460, "Total Points"=w1459, "Integration Time"=w1458) -> (w1466:T21)  [unwired: 1 in]
                                n979 = Bundle("Var1 sweep settings"=w1430, "Var1 sweep settings 2"=w1457, "Var2 step settings"=w1456, "Var2 step settings 2"=w1455) -> (w1454:T17)  [unwired: 1 in]
                                n980 = local read "Gate Current Cluster"() -> (w1400:T6)
                                n981 = Bundle("Wait Countdown"=w1452, "Wait Time (s)"=w1451) -> (w1453:T14)  [unwired: 1 in]
                                n982 = Unbundle By Name(w1430) -> ("compliance (A)"=w1424:dbl)
                                n983 = local read "Dielectric Constant:"() -> (w1402:dbl)
                                n984 = local read "Gated SMU4 is..."() -> (w1391:bool)
                                n985 = Multiply(x=w1424, y=0.05) -> (x*y=w1425:dbl)
                                n986 = Subtract(x=w1424, y=w1425) -> (x-y=w1423:dbl)
                                n987 = Add(x=w1424, y=w1425) -> (x+y=w1426:dbl)
                                n988 = local read "Stop \nCountdown"() -> (w1449:bool)
                                n989 = call "Sub Super Duper_14_02_18_JWa.vi"("VISA resource name"=w1448, "Sample Properties:"=w1480, "Gated SMU4 is..."=w1391, "TRF Cluster"=w1467, "TSP Cluster"=w1466, "Compliance Cluster"=w1454, "error in"=w1399, "Saved Folder:"=w1481, "Wait Cluster"=w1453, "Stop \nCountdown"=w1449, "Loop Count"=w1390, "Gate Current Cluster"=w1400, "Dielectric Constant (BG)"=w1402) -> ("Status Indicator"=w1447:bool, "Vt Cluster"=w1431:T23, "VISA resource name out"=w1396:refnum<visa-resource-name>, "Graph Cluster"=w1410:T18, "Char Cluster"=w1450:T19, "error out"=w1397:errorcluster)  [unwired: 7 in, 2 out]
                                n990 = while {
                                tunnel: w1447 -> [w1570]
                                tunnel: w1443 -> [w1575]
                                tunnel: w1442 -> [w1574]
                                shift-right: [w1558] -> w1446
                                shift-left: w1445 -> [w1560]
                                shift-right: [w1557] -> w1441
                                shift-left: w1444 -> [w1559]
                                i -> [w1535]
                                stop <- w1569 continue-if-true
                                w1543 = 1
                                w1548 = TRUE
                                n991 = local read "Time Iteration (s)"() -> (w1562:dbl)
                                n992 = call "Elapsed Time6"("Time Target (s)"=w1562, "Auto Reset"=TRUE) -> ("Present (s)"=w1564:dbl, "Time has Elapsed"=w1566:bool)  [unwired: 10 in, 6 out]
                                n993 = call "Lakeshore_monitor.vi"("error? 2"=w1574, "VISA Resource (TPX)"=w1575) -> ("error?"=w1572:errorcluster, "Outputs"=w1578:T12, "Inputs"=w1579:T13, "VISA resource name"=w1573:refnum<visa-resource-name>)  [unwired: 5 in]
                                n994 = local read "Start Time Num"() -> (w1563:dbl)
                                n995 = Unbundle(w1578) -> ("P"=w1595:dbl, "I"=w1594:dbl, "D"=w1593:dbl, "SetPoint Out2"=w1592:dbl, "1"=w1591:bool, "2"=w1590:bool, "output control loop"=w1589:dbl, "AutoTune Error"=w1597:bool, "AutoTune Active"=w1596:bool, "AutoTune Stage"=w1588:dbl, "Out1 Active"=w1587:bool, "Out1 Ramp On"=w1586:bool, "Out2 Active"=w1585:bool, "Out2 Ramp On"=w1584:bool, "Heater 2 Output 1"=w1583:dbl, "Heater 1 Output 2"=w1580:dbl, "Out1 Ramp"=w1582:dbl, "Out2 Ramp"=w1581:dbl)  [unwired: 1 out]
                                n996 = Unbundle(w1579) -> ("A:  Sample Stage"=w1554:dbl, "B:  Rad Shield"=w1556:dbl, "B: Probe Arm"=w1555:dbl, "Temp Max Alarm"=w1577:bool, "Temp Min Alarm"=w1576:bool)
                                n997 = Greater Than 0?(x=w1554) -> (x > 0?=w1568:bool)
                                n998 = Subtract(x=w1564, y=w1563) -> (x-y=w1565:dbl)
                                n999 = case shown="True" w1568 {
                                tunnel: w1565 -> [_ w1617]
                                tunnel: [_ w1615] -> w1557
                                tunnel: [_ w1614] -> w1558
                                tunnel: w1560 -> [_ w1610]
                                tunnel: w1559 -> [_ w1613]
                                tunnel: w1554 -> [_ w1612]
                                frame False {
                                }
                                frame True {
                                n1000 = Build Array (concatenate)(w1613, w1617) -> (w1615:dbl[])
                                n1001 = Build Array (concatenate)(w1610, w1612) -> (w1614:dbl[])
                                n1002 = Bundle(w1615, w1614) -> (w1616:cluster{dbl[], dbl[]})  [unwired: 1 in]
                                n1003 = Build Array(w1616) -> (w1611:cluster{dbl[], dbl[]}[])
                                n1004 = local write "Temp Graph"(w1611) -> ()
                                }
                                }
                                n1005 = local write "Elapsed Time"(w1565) -> ()
                                n1006 = local write "A:  Sample Stage"(w1554) -> ()
                                n1007 = local write "1"(w1591) -> ()
                                n1008 = local write "AutoTune Error"(w1597) -> ()
                                n1009 = local write "B:  Rad Shield"(w1556) -> ()
                                n1010 = And(x=w1568, y=w1566) -> (x .and. y?=w1567:bool)
                                n1011 = local write "Temp Max Alarm"(w1577) -> ()
                                n1012 = local write "Temp Min Alarm"(w1576) -> ()
                                n1013 = local write "P"(w1595) -> ()
                                n1014 = local write "C:  Probe Arm"(w1555) -> ()
                                n1015 = local write "Heater 1 Output2"(w1580) -> ()
                                n1016 = local write "AutoTune Stage"(w1588) -> ()
                                n1017 = local write "Heater 2 Output1"(w1583) -> ()
                                n1018 = local write "Out2 Ramp"(w1581) -> ()
                                n1019 = local write "Out1 Ramp"(w1582) -> ()
                                n1020 = local write "2"(w1590) -> ()
                                n1021 = local write "I"(w1594) -> ()
                                n1022 = local write "output control loop"(w1589) -> ()
                                n1023 = local write "Setpoint (K)"(w1592) -> ()
                                n1024 = local write "D"(w1593) -> ()
                                n1025 = local write "AutoTune Active"(w1596) -> ()
                                n1026 = local read "A: Low Alarm"() -> (w1546:dbl)
                                n1027 = local read "A: High Alarm"() -> (w1547:dbl)
                                n1028 = local read "Abort?"() -> (w1514:bool)
                                n1029 = Compound Arithmetic op=OR(w1577, w1576, w1514) -> (w1517:bool)
                                n1030 = local write "Out 2\nRamp On"(w1584) -> ()
                                n1031 = local write "Out 2\nActive"(w1585) -> ()
                                n1032 = local write "Out 1\nActive"(w1587) -> ()
                                n1033 = call "Configure Alarm.vi"("VISA resource name"=w1573, "High Value (0.00000)"=w1547, "Low Value (0.00000)"=w1546, "Enable Alarm (F: Off)"=w1548, "Enable Latching (F: Off)"=w1548, "error in (no error)"=w1572, "Enable Beep (F: Off)"=w1548, "Enable Display (F: Off)"=w1517) -> ("VISA resource name out"=w1552:refnum<visa-resource-name>, "error out"=w1551:errorcluster)  [unwired: 6 in]
                                n1034 = Not(x=w1514) -> (.not. x?=w1571:bool)
                                n1035 = local write "Out 1\nRamp On"(w1586) -> ()
                                n1036 = local write "Abort?"(w1517) -> ()
                                n1037 = local read "Out 2\nRamp On"() -> (w1516:bool)
                                n1038 = local read "Out 1\nRamp On"() -> (w1515:bool)
                                n1039 = call "Configure Alarm.vi"("VISA resource name"=w1552, "High Value (0.00000)"=w1547, "Low Value (0.00000)"=w1546, "Input (0:A)"=w1543, "Enable Alarm (F: Off)"=w1548, "Enable Latching (F: Off)"=w1548, "error in (no error)"=w1551, "Enable Beep (F: Off)"=w1548, "Enable Display (F: Off)"=w1517) -> ("VISA resource name out"=w1550:refnum<visa-resource-name>, "error out"=w1549:errorcluster)  [unwired: 5 in]
                                n1040 = And(x=w1570, y=w1571) -> (x .and. y?=w1569:bool)
                                n1041 = case shown="True" w1515 {
                                frame False {
                                n1042 = property on="1" class="Bool (strict)"("BoolText.Text"="") -> ()  [unwired: 2 in, 2 out]
                                }
                                frame True {
                                n1043 = local read "Out 1\nActive"() -> (w1603:bool)
                                n1044 = case shown="False" w1603 {
                                frame False {
                                n1045 = property on="1" class="Bool (strict)"("BoolText.Text"="Ramp\nOn") -> ()  [unwired: 2 in, 2 out]
                                }
                                frame True {
                                n1046 = property on="1" class="Bool (strict)"("BoolText.Text"="Ramp\nActive") -> ()  [unwired: 2 in, 2 out]
                                }
                                }
                                }
                                }
                                n1047 = case shown="False" w1516 {
                                frame False {
                                n1048 = property on="2" class="Bool (strict)"("BoolText.Text"="") -> ()  [unwired: 2 in, 2 out]
                                }
                                frame True {
                                n1049 = local read "Out 2\nActive"() -> (w1599:bool)
                                n1050 = case shown="True" w1599 {
                                frame False {
                                n1051 = property on="2" class="Bool (strict)"("BoolText.Text"="Ramp\nOn") -> ()  [unwired: 2 in, 2 out]
                                }
                                frame True {
                                n1052 = property on="2" class="Bool (strict)"("BoolText.Text"="Ramp\nActive") -> ()  [unwired: 2 in, 2 out]
                                }
                                }
                                }
                                }
                                n1053 = local read "Name/Email List Location"() -> (w1533:path)
                                n1054 = local read "Text Editor Location"() -> (w1534:path)
                                n1055 = local read "User's Name"() -> (w1532:u16)
                                n1056 = Quotient & Remainder(x=w1535, y=3) -> (x-y*floor(x/y)=w1538:i32)  [unwired: 1 out]
                                n1057 = local read "Edit Users"() -> (w1529:bool)
                                n1058 = Get Date/Time In Seconds() -> (seconds since 1Jan1904=w1526:timestamp)
                                n1059 = case shown="True" w1529 {
                                frame False {
                                }
                                frame True {
                                n1060 = local write "Edit Users"(FALSE) -> ()
                                }
                                }
                                n1061 = case shown="2" w1538 {
                                tunnel: ["." ".." "..."] -> w1537
                                frame 0, Default {
                                }
                                frame 1 {
                                }
                                frame 2 {
                                }
                                }
                                n1062 = Get Date/Time String(seconds (now)=w1526, want seconds? (F)=TRUE) -> (time string=w1528:string)  [unwired: 1 in, 1 out]
                                n1063 = local read "Status Table"() -> (w1523:string[][])
                                n1064 = call "Email_List_subvi.vi"("Open File"=w1529, "Name Ring In"=w1532, "List Location"=w1533, "Text Editor Location"=w1534) -> ("String"=w1531:string, "Names Out"=w1530:string[])  [unwired: 5 in, 1 out]
                                n1065 = Array Size(array=w1523) -> (size(s)=w1524:i32[])
                                n1066 = Concatenate Strings("Measuring", w1537) -> (w1521:string)
                                n1067 = Build Array(w1528, w1521) -> (w1522:string[])
                                n1068 = local write "User's Email"(w1531) -> ()
                                n1069 = property on="User's Name" class="Ring (strict)"("Strings []"=w1530) -> ()  [unwired: 2 in, 2 out]
                                n1070 = Index Array(array=w1524, index=0) -> (element=w1519:i32)
                                n1071 = Decrement(x=w1519) -> (x-1=w1520:i32)
                                n1072 = Replace Array Subset(array=w1523, new element=w1522, index (row)=w1520) -> (w1518:string[][])  [unwired: 1 in]
                                n1073 = case shown="True" w1567 {
                                tunnel: w1565 -> [_ w1633]
                                tunnel: w1554 -> [_ w1622]
                                tunnel: w1556 -> [_ w1621]
                                tunnel: w1555 -> [_ w1620]
                                tunnel: w1518 -> [_ w1618]
                                frame False {
                                }
                                frame True {
                                n1074 = local read "Temperature Measurements"() -> (w1634:path)
                                n1075 = Number To Decimal String(number=w1633) -> (decimal integer string=w1629:string)  [unwired: 1 in]
                                n1076 = Number To Fractional String(number=w1622) -> (F-format string=w1628:string)  [unwired: 3 in]
                                n1077 = Get Date/Time In Seconds() -> (seconds since 1Jan1904=w1630:timestamp)
                                n1078 = Number To Fractional String(number=w1621) -> (F-format string=w1625:string)  [unwired: 3 in]
                                n1079 = Number To Fractional String(number=w1620) -> (F-format string=w1624:string)  [unwired: 3 in]
                                n1080 = Get Date/Time String(seconds (now)=w1630, want seconds? (F)=TRUE) -> (date string=w1626:string, time string=w1627:string)  [unwired: 1 in]
                                n1081 = Build Array(w1629, w1628, w1625, w1624, w1627, w1626) -> (w1632:string[])
                                n1082 = call-poly <vilib>:"Write To Spreadsheet File.vi"("append to file? (new file:F)"=TRUE, "1D data"=w1632, "file path (dialog if empty)"=w1634) -> ()  [unwired: 5 in, 1 out]
                                n1083 = local read "Status"() -> (w1619:path)
                                n1084 = call-poly <vilib>:"Write To Spreadsheet File.vi"("2D data"=w1618, "file path (dialog if empty)"=w1619) -> ()  [unwired: 6 in, 1 out]
                                }
                                }
                                n1085 = local write "Status Table"(w1518) -> ()
                                n1086 = local read "P 2"() -> (w1542:dbl)
                                n1087 = local read "D 2"() -> (w1540:dbl)
                                n1088 = local read "I 2"() -> (w1541:dbl)
                                n1089 = call "Configure PID.vi"("VISA resource name"=w1550, "Output's Control Loop (1:1)"=2, "Gain (P) (50.0)"=w1542, "Reset (I) (20.0)"=w1541, "error in (no error)"=w1549, "Rate (D) (0.0 %)"=w1540) -> ("VISA resource name out"=w1545:refnum<visa-resource-name>, "error out"=w1544:errorcluster)  [unwired: 8 in]
                                n1090 = call "Configure PID.vi"("VISA resource name"=w1545, "Output's Control Loop (1:1)"=w1543, "Gain (P) (50.0)"=w1542, "Reset (I) (20.0)"=w1541, "error in (no error)"=w1544, "Rate (D) (0.0 %)"=w1540) -> ()  [unwired: 8 in, 2 out]
                                }
                                n1091 = Unbundle By Name(w1431) -> ("Vt Ratio"=w1428:i32)  [unwired: 1 out]
                                n1092 = Greater?(x=w1428, y=3) -> (0:w1421:bool)
                                n1093 = local write "Status LED"(w1447) -> ()
                                n1094 = Unbundle By Name(w1450) -> ("Mobility-Sat"=w1420:dbl, "Mobility-Lin"=w1419:dbl, "On/Off"=w1414:dbl, "Off I"=w1413:dbl, "Vt"=w1418:dbl, "STS"=w1417:dbl, "Trap Density-VT"=w1416:dbl, "Trap Density-STS"=w1415:dbl)
                                n1095 = Multiply(x=w1414, y=w1413) -> (x*y=w1412:dbl)
                                n1096 = In Range and Coerce(upper limit=w1426, x=w1412, lower limit=w1423) -> (In Range?=w1422:bool)  [unwired: 1 out]
                                n1097 = Or(x=w1421, y=w1422) -> (x .or. y?=w1411:bool)
                                n1098 = local write "Measurement Error"(w1411) -> ()
                                n1099 = case shown="True" w1411 {
                                tunnel: w1421 -> [_ w1485]
                                frame False {
                                n1100 = local write "Measurement Repeat"(FALSE) -> ()
                                n1101 = local write "Error Loop #"(0) -> ()
                                }
                                frame True {
                                n1102 = flat-sequence {
                                tunnel: w1485 -> [w1487]
                                tunnel: [w1486] -> w1484
                                tunnel: w1484 -> [w1499]
                                frame #0 {
                                n1103 = disable-structure shown="Disabled" {
                                disable-tunnel: w1487 -> [w1491 _]
                                disable-tunnel: [w1488 _] -> w1486
                                frame Disabled {
                                n1104 = local read "User's Email"() -> (w1493:string)
                                n1105 = property on="User's Name" class="Ring (strict)"() -> ("RingText.Text"=w1494:string)  [unwired: 2 in, 2 out]
                                n1106 = Select(t="Your measurement indicates an open circuit.  \nPlease fix before continuing the measurements", s=w1491, f="Your measurement has reached the compliance current.  \nPlease fix before continuing the measurements") -> (s? t:f=w1488:string)
                                n1107 = call "subgmail.vi"("Recipient's Email Address Address"=w1493, "Recipient's Name"=w1494, "Subject"="TPX - Measurement Error", "Body"=w1488) -> ()  [unwired: 12 in]
                                }
                                frame Enabled {
                                }
                                }
                                }
                                frame #1 {
                                n1108 = local read "Error Loop #"() -> (w1496:dbl)
                                n1109 = local read "Repeat if error?"() -> (w1497:bool)
                                n1110 = Equal To 0?(x=w1496) -> (x = 0?=w1495:bool)
                                n1111 = And(x=w1497, y=w1495) -> (x .and. y?=w1498:bool)
                                n1112 = case shown="False" w1498 {
                                tunnel: w1499 -> [w1502 _]
                                frame False {
                                n1113 = local read "Continue if error?"() -> (w1500:bool)
                                n1114 = case shown="False" w1500 {
                                tunnel: w1502 -> [w1506 _]
                                frame False {
                                n1115 = Two Button Dialog(message=w1506, 1:"Continue without Repeat?", 2:"Repeat Measurement?") -> (T button?=w1503:bool)
                                n1116 = local write "Measurement Repeat"(w1503) -> ()
                                }
                                frame True {
                                n1117 = local write "Measurement Repeat"(FALSE) -> ()
                                }
                                }
                                n1118 = local write "Error Loop #"(0) -> ()
                                }
                                frame True {
                                n1119 = local read "Error Loop #"() -> (w1509:dbl)
                                n1120 = local write "Measurement Repeat"(TRUE) -> ()
                                n1121 = Increment(x=w1509) -> (x+1=w1508:dbl)
                                n1122 = local write "Error Loop #"(w1508) -> ()
                                }
                                }
                                }
                                }
                                }
                                }
                                n1123 = Unbundle By Name(w1410) -> ("Linear Transfer"=w1407:cluster{dbl[], "trace":dbl[]}[], "Linear Raw"=w1408:cluster{dbl[], dbl[]}[], "Saturation Transfer"=w1406:cluster{dbl[], "trace":dbl[]}[], "Saturation Raw"=w1409:cluster{dbl[], dbl[]}[], "Transport"=w1405:cluster{dbl[], dbl[]}[], "TRF Gate Current"=w1401:cluster{dbl[], dbl[]}[])
                                n1124 = local write "Mobility-Sat"(w1420) -> ()
                                n1125 = local write "Mobility-Lin"(w1419) -> ()
                                n1126 = local write "Trap Density-VT"(w1416) -> ()
                                n1127 = local write "Trap Density-STS"(w1415) -> ()
                                n1128 = local write "Off Current"(w1413) -> ()
                                n1129 = local write "On/Off"(w1414) -> ()
                                n1130 = local write "STS"(w1417) -> ()
                                n1131 = local write "Vt"(w1418) -> ()
                                n1132 = local write "Transport Graph"(w1405) -> ()
                                n1133 = local write "Saturation Raw"(w1409) -> ()
                                n1134 = local write "Linear Raw"(w1408) -> ()
                                n1135 = local write "Mobility-Sat TPX"(w1420) -> ()
                                n1136 = local write "Mobility-Lin TPX"(w1419) -> ()
                                n1137 = local write "Trap Density VT TPX"(w1416) -> ()
                                n1138 = local write "Off Current TPX"(w1413) -> ()
                                n1139 = local write "On/Off TPX"(w1414) -> ()
                                n1140 = local write "STS TPX"(w1417) -> ()
                                n1141 = local write "Vt TPX"(w1418) -> ()
                                n1142 = local write "Trap Density STS TPX"(w1415) -> ()
                                n1143 = local write "Linear Transfer"(w1407) -> ()
                                n1144 = Index Array(array=w1405, index=0) -> (element=w1403:cluster{dbl[], dbl[]})
                                n1145 = local read "Light Bathe Cluster"() -> (w1393:T2)
                                n1146 = local write "TSF Gate Current"(w1401) -> ()
                                n1147 = local write "TPX Transport Graph"(w1403) -> ()
                                n1148 = Unbundle By Name(w1393) -> ("Post Measure:"=w1392:bool)
                                n1149 = local write "TPX Transfer Graph"(w1406) -> ()
                                n1150 = local read "Time Iteration (s)"() -> (w1394:dbl)
                                n1151 = call "Elapsed Time9"("Time Target (s)"=w1394, "error in (no error)"=w1397) -> ("Present (s)"=w1398:dbl, "error out"=w1395:errorcluster)  [unwired: 10 in, 6 out]
                                n1152 = local write "Delay Start"(w1398) -> ()
                                n1153 = case shown="True" w1392 {
                                tunnel: w1396 -> [_ w1512]
                                tunnel: w1395 -> [_ w1511]
                                frame False {
                                }
                                frame True {
                                w1513 = u32 1 items=["positive pulse  ", "negative pulse  ", "level high  ", "level low  "] ("trigger signal")
                                n1154 = call "HP415xA Op-Trigger Output.vi"("error in (no error)"=w1511, "trigger signal"=w1513, "VISA session"=w1512) -> ()  [unwired: 1 in, 1 out]
                                }
                                }
                                n1155 = Index Array(array=w1406, index=0) -> (element=w1439:cluster{dbl[], "trace":dbl[]})
                                n1156 = Unbundle(w1439) -> ("trace"=w1437:dbl[])  [unwired: 1 out]
                                n1157 = To Double Precision Float(number=1) -> (double precision float=w1435:dbl)
                                n1158 = Array Max & Min(array=w1437) -> (max value=w1434:dbl, min value=w1433:dbl)  [unwired: 2 out]
                                n1159 = Bundle(w1433, w1434, w1435, w1435, w1435) -> (w1432:cluster{dbl, dbl, dbl, dbl, dbl})  [unwired: 1 in]
                                n1160 = property on="TPX Transfer Graph" class="XYGraph (strict)"("Active Plot"=1, "YScale.Range"=w1432) -> ()  [unwired: 2 in, 2 out]
                                }
                                frame #2 {
                                # "Integer from for loop"
                                # "Number of looops"
                                n1161 = node-c288(100) -> (w1641:T9)  [unwired: 3 in]
                                n1162 = timed-loop {
                                timing: w1641 -> [_]
                                timing-out: [_] -> w1640
                                tunnel: w1637 -> [w1651]
                                tunnel: w1638 -> [w1650]
                                tunnel: [w1643] -> _
                                i -> [w1655]
                                stop <- w1646 stop-if-true
                                n1163 = node-c288() -> ()  [unwired: 1 in, 1 out]
                                n1164 = local read "Loop Wait 2"() -> (w1645:dbl)
                                n1165 = Multiply(x=0.1, y=w1655) -> (x*y=w1653:dbl)
                                n1166 = Equal?(x=w1650, y=w1651) -> (x = y?=w1652:bool)
                                n1167 = Select(t=0, s=w1652, f=w1645) -> (s? t:f=w1648:dbl)
                                n1168 = Subtract(x=w1648, y=w1653) -> (x-y=w1644:dbl)
                                n1169 = Less Or Equal To 0?(x=w1644) -> (x <= 0?=w1647:bool)
                                n1170 = local read "Stop \nCountdown 2"() -> (w1643:bool)
                                n1171 = Or(x=w1647, y=w1643) -> (x .or. y?=w1646:bool)
                                n1172 = local write "Wait Countdown 2"(w1644) -> ()
                                n1173 = property on="Status LED" class="Bool (strict)"("BoolText.Text"="Waiting...") -> ()  [unwired: 2 in, 2 out]
                                n1174 = node-c288() -> ()  [unwired: 1 in, 1 out]
                                }
                                n1175 = node-c288(w1640) -> (w1636:errorcluster)
                                n1176 = property on="Status LED" class="Bool (strict)"(error in=w1636, "BoolText.Text"="Ready") -> ()  [unwired: 1 in, 2 out]
                                }
                                }
                                }
                                }
                                frame True {
                                n1177 = case shown="True" w1665 {
                                frame False {
                                }
                                frame True {
                                n1178 = local write "# Steps"(-1) -> ()
                                }
                                }
                                }
                                }
                              }
                              frame #3 {
                                n1179 = local read "Measurement Error"() -> (w1672:bool)
                                n1180 = local read "Measurement Repeat"() -> (w1670:bool)
                                n1181 = Select(t=" Complete WITH ERROR", s=w1672, f=" Complete") -> (s? t:f=w1671:string)
                                n1182 = local read "Current Step"() -> (w1669:dbl)
                                n1183 = Select(t=" Repeating...", s=w1670, f=w1671) -> (s? t:f=w1676:string)
                                n1184 = local read "# Steps"() -> (w1692:dbl)
                                n1185 = local read "Time Iteration (s)"() -> (w1716:dbl)
                                n1186 = local read "Start Time Num"() -> (w1715:dbl)
                                n1187 = call "Lakeshore_monitor.vi"("error? 2"=w1701, "VISA Resource (TPX)"=w1702) -> ("Inputs"=w1709:T13)  [unwired: 5 in, 3 out]
                                n1188 = call "Elapsed Time8"("Time Target (s)"=w1716, "Auto Reset"=TRUE) -> ("Present (s)"=w1714:dbl)  [unwired: 10 in, 7 out]
                                n1189 = Unbundle(w1709) -> ("A:  Sample Stage"=w1681:dbl, "B:  Rad Shield"=w1708:dbl, "B: Probe Arm"=w1707:dbl)  [unwired: 2 out]
                                n1190 = Subtract(x=w1714, y=w1715) -> (x-y=w1705:dbl)
                                n1191 = Increment(x=w1669) -> (x+1=w1668:dbl)
                                n1192 = local write "A:  Sample Stage"(w1681) -> ()
                                n1193 = Number To Decimal String(number=w1669) -> (decimal integer string=w1695:string)  [unwired: 1 in]
                                n1194 = local read "Temperature Measurements"() -> (w1711:path)
                                n1195 = local write "B:  Rad Shield"(w1708) -> ()
                                n1196 = Number To Decimal String(number=w1692) -> (decimal integer string=w1691:string)  [unwired: 1 in]
                                n1197 = local write "C:  Probe Arm"(w1707) -> ()
                                n1198 = Build Array (concatenate)(w1699, w1705) -> (w1697:dbl[])
                                n1199 = Build Array (concatenate)(w1700, w1681) -> (w1698:dbl[])
                                n1200 = Select(t=w1669, s=w1670, f=w1668) -> (s? t:f=w1667:dbl)
                                n1201 = Bundle(w1697, w1698) -> (w1706:cluster{dbl[], dbl[]})  [unwired: 1 in]
                                n1202 = Concatenate Strings("Loop #", w1695, " of ", w1691, w1676) -> (w1696:string)
                                n1203 = local write "Current Step"(w1667) -> ()
                                n1204 = Build Array(w1706) -> (w1704:cluster{dbl[], dbl[]}[])
                                n1205 = Build Array("", w1696) -> (w1678:string[])
                                n1206 = Build Array("Measurement Finished") -> (w1703:string[])
                                n1207 = Get Date/Time In Seconds() -> (seconds since 1Jan1904=w1688:timestamp)
                                n1208 = local read "Status Table"() -> (w1685:string[][])
                                n1209 = local write "Temp Graph"(w1704) -> ()
                                n1210 = Get Date/Time String(seconds (now)=w1688, want seconds? (F)=TRUE) -> (time string=w1690:string)  [unwired: 1 in, 1 out]
                                n1211 = Build Array(w1690, "Measurement Complete") -> (w1684:string[])
                                n1212 = local read "Status"() -> (w1682:path)
                                n1213 = Array Size(array=w1685) -> (size(s)=w1686:i32[])
                                n1214 = Insert Into Array(array=w1685, new element=w1684) -> (w1680:string[][])  [unwired: 2 in]
                                n1215 = Insert Into Array(array=w1680, new element=w1678) -> (w1677:string[][])  [unwired: 2 in]
                                n1216 = local write "Status Table"(w1677) -> ()
                                n1217 = call-poly <vilib>:"Write To Spreadsheet File.vi"("2D data"=w1677, "file path (dialog if empty)"=w1682) -> ()  [unwired: 6 in, 1 out]
                                n1218 = Index Array(array=w1686, index=0) -> ()  [unwired: 1 out]
                                n1219 = Number To Fractional String(number=w1681) -> (F-format string=w1719:string)  [unwired: 3 in]
                                n1220 = Number To Decimal String(number=w1705) -> (decimal integer string=w1724:string)  [unwired: 1 in]
                                n1221 = Get Date/Time In Seconds() -> (seconds since 1Jan1904=w1718:timestamp)
                                n1222 = Number To Fractional String(number=w1708) -> (F-format string=w1722:string)  [unwired: 3 in]
                                n1223 = Number To Fractional String(number=w1707) -> (F-format string=w1723:string)  [unwired: 3 in]
                                n1224 = Get Date/Time String(seconds (now)=w1718, want seconds? (F)=TRUE) -> (date string=w1721:string, time string=w1720:string)  [unwired: 1 in]
                                n1225 = Build Array(w1724, w1719, w1722, w1723, w1720, w1721) -> (w1726:string[])
                                n1226 = Build Array(w1726, w1703) -> (w1713:string[][])
                                n1227 = call-poly <vilib>:"Write To Spreadsheet File.vi"("append to file? (new file:F)"=TRUE, "2D data"=w1713, "file path (dialog if empty)"=w1711) -> ()  [unwired: 5 in, 1 out]
                              }
                            }
                          }
                          frame True {
                          }
                        }
                      }
                    }
                  }
                  n1228 = local write "Array"(w419) -> ()
                  n1229 = local write "Array 2"(w418) -> ()
                }
                frame #1 {
                  n1230 = local read "Reverse Scan (Y/N)"() -> (w1727:bool)
                  n1231 = case shown="True" w1727 {
                    frame False {
                      w1733 = TRUE
                      n1232 = local read "Post Rate (K/min)"() -> (w1729:dbl)
                      n1233 = local read "VISA Resource (TPX)"() -> (w1734:refnum<visa-resource-name>)
                      n1234 = local read "Post Temp (K)"() -> (w1730:dbl)
                      n1235 = call "Configure Setpoint and Ramp.vi"("VISA resource name"=w1734, "Output's Control Loop (1:1)"=2, "Setpoint (0.00000)"=w1730, "Setpoint Ramping \nEnable (F: Off)"=w1733, "Ramp Rate (0.0)"=w1729) -> ("VISA resource name out"=w1728:refnum<visa-resource-name>)  [unwired: 9 in, 1 out]
                      n1236 = call "Configure Setpoint and Ramp.vi"("VISA resource name"=w1728, "Output's Control Loop (1:1)"=1, "Setpoint (0.00000)"=w1730, "Setpoint Ramping \nEnable (F: Off)"=w1733, "Ramp Rate (0.0)"=w1729) -> ()  [unwired: 9 in, 2 out]
                    }
                    frame True {
                      n1237 = flat-sequence {
                        frame #0 {
                          n1238 = local read "Start (K)"() -> (w1736:dbl)
                          n1239 = local read "Stop (K)"() -> (w1737:dbl)
                          n1240 = local write "Start buffer"(w1736) -> ()
                          n1241 = local write "Stop buffer"(w1737) -> ()
                        }
                        frame #1 {
                          n1242 = local read "Start buffer"() -> (w1739:dbl)
                          n1243 = local read "Stop buffer"() -> (w1738:dbl)
                          n1244 = local write "Stop (K)"(w1739) -> ()
                          n1245 = local write "Start (K)"(w1738) -> ()
                        }
                      }
                      n1246 = local write "Current Step"(0) -> ()
                    }
                  }
                }
              }
            }
            n1247 = local read "VISA Resource (TPX)"() -> (w411:refnum<visa-resource-name>)
            n1248 = local read "Abort?"() -> (w410:bool)
            n1249 = call "Kill All.vi"("STOP"=w410, "VISA resource in"=w411) -> ("STOP out"=w409:bool)  [unwired: 2 in, 1 out]
          }
          frame #2 {
            n1250 = Get Date/Time In Seconds() -> (seconds since 1Jan1904=w1749:timestamp)
            n1251 = Get Date/Time String(seconds (now)=w1749, want seconds? (F)=TRUE) -> (time string=w1747:string)  [unwired: 1 in, 1 out]
            n1252 = local read "Status Table"() -> (w1752:string[][])
            n1253 = Concatenate Strings("Finished") -> (w1746:string)
            n1254 = Build Array(w1747, w1746) -> (w1753:string[])
            n1255 = Array Size(array=w1752) -> (size(s)=w1751:i32[])
            n1256 = Insert Into Array(array=w1752, new element=w1753) -> (w1754:string[][])  [unwired: 2 in]
            n1257 = Index Array(array=w1751, index=0) -> ()  [unwired: 1 out]
            n1258 = case shown="True" TRUE {
              selector: TRUE -> [w1756 w1767]
              tunnel: [w1756 w1767] -> _
              frame False {
              }
              frame True {
                n1259 = local read "Temp Min Alarm"() -> (w1764:bool)
                n1260 = local read "Temp Max Alarm"() -> (w1765:bool)
                n1261 = local read "Abort?"() -> (w1762:bool)
                n1262 = property on="User's Name" class="Ring (strict)"() -> ("RingText.Text"=w1766:string)  [unwired: 2 in, 2 out]
                n1263 = Or(x=w1765, y=w1764) -> (x .or. y?=w1763:bool)
                n1264 = case shown="True" w1763 {
                  tunnel: ["" "Temperature Alarm!!!"] -> w1759
                  frame False {
                  }
                  frame True {
                  }
                }
                n1265 = case shown="False" w1762 {
                  tunnel: [w1772 w1774] -> w1761
                  tunnel: ["TPX Notification" "TPX WARNING"] -> w1757
                  frame False {
                    w1772 = "Note: Your measurement is complete!!"  # Note: Your measurement is complete!!
                  }
                  frame True {
                    w1774 = "Note: Your measurement was ABORTED!!"  # Note: Your measurement was ABORTED!!
                  }
                }
                n1266 = local read "User's Email"() -> (w1768:string)
                n1267 = Concatenate Strings(w1761, "\r", w1759) -> (w1758:string)
                n1268 = call "subgmail.vi"("Recipient's Email Address Address"=w1768, "Recipient's Name"=w1766, "Subject"=w1757, "Body"=w1758) -> ()  [unwired: 12 in]
              }
            }
            n1269 = local write "Status Table"(w1754) -> ()
            n1270 = local read "VISA Resource (TPX)"() -> (w1740:refnum<visa-resource-name>)
            n1271 = local read "Temp Min Alarm"() -> (w1742:bool)
            n1272 = local read "Temp Max Alarm"() -> (w1743:bool)
            n1273 = local read "Abort?"() -> (w1744:bool)
            n1274 = Compound Arithmetic op=OR(w1744, w1743, w1742) -> (w1741:bool)
            n1275 = call "Kill All.vi"("STOP"=w1741, "VISA resource in"=w1740) -> ()  [unwired: 2 in, 2 out]
          }
        }
      }
      event "stop": Value Change {
        n1276 = event-data() -> ("NewVal"=w1776:bool)  [unwired: 1 in, 4 out]
        n1277 = local read "stop"() -> (w1775:bool)
        n1278 = local write "Status LED"(FALSE) -> ()
        n1279 = local write "Loop Wait"(0) -> ()
      }
    }
    n1280 = local write "1"(w39) -> ()
    n1281 = local write "P"(w43) -> ()
    n1282 = local write "A:  Sample Stage"(w64) -> ()
    n1283 = local write "AutoTune Error"(w36) -> ()
    n1284 = local write "B:  Rad Shield"(w45) -> ()
    n1285 = local write "Temp Max Alarm"(w25) -> ()
    n1286 = local write "Temp Min Alarm"(w24) -> ()
    n1287 = local write "C:  Probe Arm"(w44) -> ()
    n1288 = local write "Heater 1 Output2"(w30) -> ()
    n1289 = local write "AutoTune Stage"(w34) -> ()
    n1290 = local write "Heater 2 Output1"(w33) -> ()
    n1291 = local write "Out2 Ramp"(w31) -> ()
    n1292 = local write "Out1 Ramp"(w32) -> ()
    n1293 = local write "2"(w38) -> ()
    n1294 = local write "I"(w42) -> ()
    n1295 = local write "output control loop"(w37) -> ()
    n1296 = local write "Setpoint (K)"(w40) -> ()
    n1297 = local write "D"(w41) -> ()
    n1298 = local write "AutoTune Active"(w35) -> ()
    n1299 = local read "A: Low Alarm"() -> (w21:dbl)
    n1300 = local read "A: High Alarm"() -> (w22:dbl)
    n1301 = Or(x=w25, y=w24) -> (x .or. y?=w11:bool)
    n1302 = local write "Out 2\nRamp On"(w17) -> ()
    n1303 = local write "Out 2\nActive"(w18) -> ()
    n1304 = local write "Out 1\nRamp On"(w19) -> ()
    n1305 = local write "Out 1\nActive"(w20) -> ()
    n1306 = call "Configure Alarm.vi"("VISA resource name"=w26, "High Value (0.00000)"=w22, "Low Value (0.00000)"=w21, "Enable Alarm (F: Off)"=w23, "Enable Latching (F: Off)"=w23, "Enable Beep (F: Off)"=w23, "Enable Display (F: Off)"=w11) -> ("VISA resource name out"=w13:refnum<visa-resource-name>)  [unwired: 7 in, 1 out]
    n1307 = local read "B: Low Alarm"() -> (w16:dbl)
    n1308 = local read "B: High Alarm"() -> (w15:dbl)
    n1309 = call "Configure Alarm.vi"("VISA resource name"=w13, "High Value (0.00000)"=w15, "Low Value (0.00000)"=w16, "Input (0:A)"=1, "Enable Alarm (F: Off)"=w14, "Enable Latching (F: Off)"=w14, "Enable Beep (F: Off)"=w14, "Enable Display (F: Off)"=w11) -> ()  [unwired: 6 in, 2 out]
    n1310 = disable-structure shown="Disabled" {
      disable-tunnel: w63 -> [w68 _]
      disable-tunnel: w26 -> [w66 _]
      frame Disabled {
        n1311 = event shown="[3] \"Abort?\": Value Change" {
          selector: _ -> [_ _ _ _]
          dyn-events: _ -> [_ _ _ _]
          timeout: 100 -> [_ _ _ _]
          tunnel: [_ _ _ TRUE] -> _
          tunnel: w66 -> [_ w70 w72 _]
          tunnel: w68 -> [_ w69 w71 _]
          event Timeout {
            n1312 = event-data() -> ()  [unwired: 1 in, 2 out]
          }
          event "Reset": Value Change {
            n1313 = event-data() -> ()  [unwired: 1 in, 5 out]
            n1314 = call "Reset Alarm.vi"("error in (no error)"=w69, "VISA resource name"=w70) -> ()  [unwired: 8 in, 2 out]
          }
          event "Alarm Reset 2": Value Change {
            n1315 = event-data() -> ()  [unwired: 1 in, 5 out]
            n1316 = call "Reset Alarm.vi"("error in (no error)"=w71, "VISA resource name"=w72) -> ()  [unwired: 8 in, 2 out]
          }
          event "Abort?": Value Change {
            n1317 = event-data() -> ()  [unwired: 1 in, 6 out]
          }
        }
      }
      frame Enabled {
      }
    }
    n1318 = local read "PT OVR"() -> (w50:bool)
    n1319 = local read "PR OVR"() -> (w49:bool)
    n1320 = case shown="False" w50 {
      frame False {
        n1321 = local read "Start (K)"() -> (w83:dbl)
        n1322 = local write "Post Temp (K)"(w83) -> ()
      }
      frame True {
      }
    }
    n1323 = case shown="False" w49 {
      frame False {
        n1324 = local read "Rate (K/min)"() -> (w82:dbl)
        n1325 = local write "Post Rate (K/min)"(w82) -> ()
      }
      frame True {
      }
    }
    n1326 = local read "Reverse Scan (Y/N)"() -> (w51:bool)
    n1327 = case shown="False" w51 {
      frame False {
        w84 = 0
        n1328 = property on="Post Rate (K/min)" class="DigNum (strict)"("DisabledEnum"=w84) -> ()  [unwired: 2 in, 2 out]
        n1329 = property on="Post Temp (K)" class="DigNum (strict)"("DisabledEnum"=w84) -> ()  [unwired: 2 in, 2 out]
      }
      frame True {
        w85 = 2
        n1330 = property on="Post Rate (K/min)" class="DigNum (strict)"("DisabledEnum"=w85) -> ()  [unwired: 2 in, 2 out]
        n1331 = property on="Post Temp (K)" class="DigNum (strict)"("DisabledEnum"=w85) -> ()  [unwired: 2 in, 2 out]
      }
    }
    n1332 = local write "Error Loop #"(0) -> ()
    n1333 = local read "Name/Email List Location"() -> (w56:path)
    n1334 = local read "Text Editor Location"() -> (w57:path)
    n1335 = local read "User's Name"() -> (w55:u16)
    n1336 = local read "Edit Users"() -> (w52:bool)
    n1337 = local read "Out 2\nRamp On"() -> (w47:bool)
    n1338 = local read "Out 1\nRamp On"() -> (w48:bool)
    n1339 = call "Email_List_subvi.vi"("Open File"=w52, "Name Ring In"=w55, "List Location"=w56, "Text Editor Location"=w57) -> ("String"=w54:string, "Names Out"=w53:string[])  [unwired: 5 in, 1 out]
    n1340 = property on="User's Name" class="Ring (strict)"("Strings []"=w53) -> ()  [unwired: 2 in, 2 out]
    n1341 = case shown="True" w52 {
      frame False {
      }
      frame True {
        n1342 = local write "Edit Users"(FALSE) -> ()
      }
    }
    n1343 = case shown="True" w47 {
      frame False {
        n1344 = property on="2" class="Bool (strict)"("BoolText.Text"="") -> ()  [unwired: 2 in, 2 out]
      }
      frame True {
        n1345 = local read "Out 2\nActive"() -> (w75:bool)
        n1346 = case shown="False" w75 {
          frame False {
            n1347 = property on="2" class="Bool (strict)"("BoolText.Text"="Ramp\nOn") -> ()  [unwired: 2 in, 2 out]
          }
          frame True {
            n1348 = property on="2" class="Bool (strict)"("BoolText.Text"="Ramp\nActive") -> ()  [unwired: 2 in, 2 out]
          }
        }
      }
    }
    n1349 = case shown="True" w48 {
      frame False {
        n1350 = property on="1" class="Bool (strict)"("BoolText.Text"="") -> ()  [unwired: 2 in, 2 out]
      }
      frame True {
        n1351 = local read "Out 1\nActive"() -> (w79:bool)
        n1352 = case shown="False" w79 {
          frame False {
            n1353 = property on="1" class="Bool (strict)"("BoolText.Text"="Ramp\nOn") -> ()  [unwired: 2 in, 2 out]
          }
          frame True {
            n1354 = property on="1" class="Bool (strict)"("BoolText.Text"="Ramp\nActive") -> ()  [unwired: 2 in, 2 out]
          }
        }
      }
    }
    n1355 = local write "User's Email"(w54) -> ()
    n1356 = local read "Temp Max Alarm"() -> (w60:bool)
    n1357 = local read "Temp Min Alarm"() -> (w62:bool)
    n1358 = Or(x=w60, y=w62) -> (x .or. y?=w61:bool)
    n1359 = local write "Alarm"(w61) -> ()
    n1360 = case shown="False" w61 {
      tunnel: w60 -> [_ w89]
      tunnel: ["" w88] -> w59
      frame False {
      }
      frame True {
        n1361 = Select(t="MAX", s=w89, f="MIN") -> (s? t:f=w88:string)
      }
    }
    n1362 = property on="Alarm" class="Bool (strict)"("BoolText.Text"=w59) -> ()  [unwired: 2 in, 2 out]
  }
  n1363 = call "Build XY Graph"() -> ("XY Graph"=→"Temp Graph":cluster{"Y":dbl[], "Y":dbl[]}[])  [unwired: 5 in, 6 out]
